vi "Autonomous Independent.vi"() -> ()   [LabVIEW 2016]
doc: "This VI is called when autonomous begins, and will automatically be terminated when autonomous ends. You can carry out timed or sensor driven robot movement independently without needing to return to the caller."
uses:
  <vilib>/Rock Robotics/WPI/Solenoid/WPI_SolenoidValue.ctl
  <vilib>/Rock Robotics/WPI/ThirdParty/CanMotor/TalonSRX/WPI_CANTalonSRX_APIControlMode.ctl
  <vilib>/Rock Robotics/Network Tables/NT Read String.vi
  Robot Global Data.vi
  <vilib>/Rock Robotics/WPI/Solenoid/WPI_SolenoidSetEnum.vi
  <vilib>/Rock Robotics/WPI/Utilities/WPI_GetSetVariantRefNum.vi
  <vilib>/addons/control/pid/pid.llb/PID (DBL).vi
  <vilib>/Rock Robotics/Network Tables/NT Read Number.vi
  <vilib>/addons/control/pid/NI_PID_pid.lvlib
  navX Library v2/navX Library v2.lvlib
panel:
  out "DriveStraight 3":T1(graph)
  out "DriveStraight 2":T1(graph)
  in  "ForwardPID 2":T2={"proportional gain (Kc)"=0.001, "integral time (Ti, min)"=0.1, "derivative time (Td, min)"=0.0}
  in  "YawFactor":dbl=0.01 format="%#_13g"
  out "YawCorrection":dbl(graph)
  out "Left V 5":cluster{"output":dbl, dbl, "Numeric":dbl}(graph)
  out "Right V 5":cluster{"output":dbl, dbl, "Numeric":dbl}(graph)
  out "Yaw 5":cluster{"Numeric":dbl, "Yaw":dbl}(graph)
  out "DriveStraight 7":T1(graph)
  out "Left V 4":cluster{"output":dbl, dbl, "Numeric":dbl}(graph)
  out "Right V 4":cluster{"output":dbl, dbl, "Numeric":dbl}(graph)
  out "Yaw 4":cluster{"Numeric":dbl, "Yaw":dbl}(graph)
  out "DriveStraight 6":T1(graph)
  out "Left V 3":cluster{"output":dbl, dbl, "Numeric":dbl}(graph)
  out "Right V 3":cluster{"output":dbl, dbl, "Numeric":dbl}(graph)
  out "Yaw 3":cluster{"Numeric":dbl, "Yaw":dbl}(graph)
  out "DriveStraight 5":T1(graph)
  out "Left V 2":cluster{"output":dbl, dbl, "Numeric":dbl}(graph)
  out "Right V 2":cluster{"output":dbl, dbl, "Numeric":dbl}(graph)
  out "Yaw 2":cluster{"Numeric":dbl, "Yaw":dbl}(graph)
  in  "RightPID":T2
  out "DriveStraight 4":T1(graph)
  out "Yaw":cluster{"Numeric":dbl, "Yaw":dbl}(graph)
  in  "ForwardPID":T2={"proportional gain (Kc)"=0.001, "integral time (Ti, min)"=0.1, "derivative time (Td, min)"=0.0}
  out "DriveStraight":T1(graph)
  in  "Center":dbl=160.0 format="%#_13g"
  in  "MOE":dbl=25.0 format="%#_13g"
  in  "Speed 2":dbl=0.45 format="%#_13g"
  in  "PID gains L":T2={"proportional gain (Kc)"=0.65, "integral time (Ti, min)"=0.01, "derivative time (Td, min)"=0.0} {"derivative time (Td, min)" format="%.3f"; "integral time (Ti, min)" format="%.6f"; "proportional gain (Kc)" format="%.6f"}
  in  "PID gains R":T2={"proportional gain (Kc)"=0.65, "integral time (Ti, min)"=0.01, "derivative time (Td, min)"=0.0} {"derivative time (Td, min)" format="%.3f"; "integral time (Ti, min)" format="%.6f"; "proportional gain (Kc)" format="%.6f"}
  in  "Range":cluster{"output high":dbl, "output low":dbl}={"output high"=1.0, "output low"=-0.5} {"output low" format="%.2f"; "output high" format="%.2f"}
  out "Left V":cluster{"output":dbl, dbl, "Numeric":dbl}(graph)
  out "Right V":cluster{"output":dbl, dbl, "Numeric":dbl}(graph)
  in  "Speed":dbl=1.0 format="%#_13g"
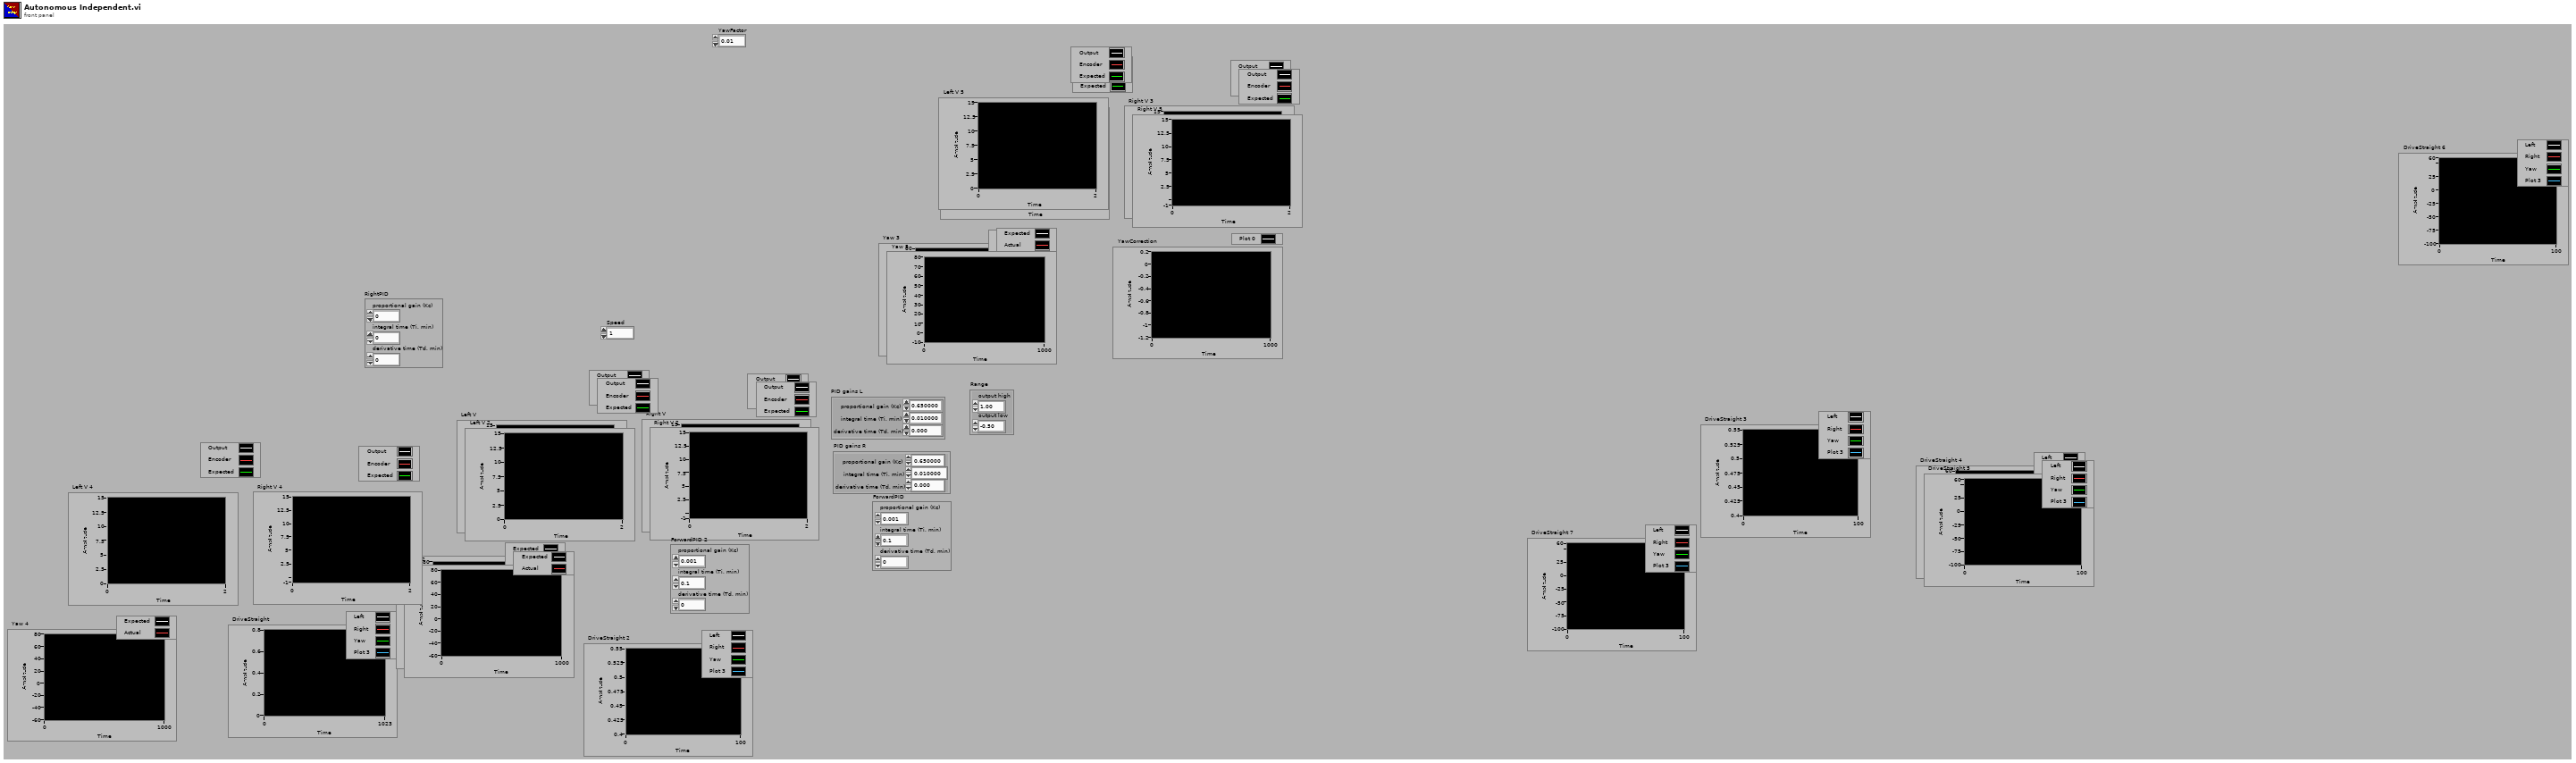
[diagram p1: front panel]
types:
  T1 = cluster{"[0]":dbl, "[1]":dbl, "[2]":dbl, "[3]":dbl, "[4]":dbl, "[5]":dbl, "[6]":dbl, "[7]":dbl, "[8]":dbl}
  T2 = cluster{"proportional gain (Kc)":dbl, "integral time (Ti, min)":dbl, "derivative time (Td, min)":dbl}
  T3 = typedef "WPI_SolenoidValue.ctl" = enum16{"Off", "On", "Forward", "Reverse"}
  T4 = typedef "WPI_CANTalonSRX_APIControlMode.ctl" = enum8{"Percent VBus", "Speed", "Position", "Slave", "Unchanged / Invalid", "Voltage Compensation", "Current", "Motion Profile", "Motion Magic"}
  T5 = typedef "WPI_SolenoidDevRef.ctl" = cluster{"DevStatus":errorcluster, "Pneumatics Control Module":u8, "Forward Solenoid Channel":T6, "Reverse Solenoid Channel":T6}
  T6 = typedef "WPI_SolenoidChannel.ctl" = enum8{"Solenoid 0", "Solenoid 1", "Solenoid 2", "Solenoid 3", "Solenoid 4", "Solenoid 5", "Solenoid 6", "Solenoid 7", "Invalid"}
  T7 = typedef "WPI_EncoderDevRef.ctl" = cluster{"DevStatus":errorcluster, "EncoderIndex":T8, "CounterIndex":T9, "DistancePerCount":dbl, "Decoding Type":T10}
  T8 = typedef "FPGA_EncoderIdx.ctl" = enum8{"Enc 0", "Enc 1", "Enc 2", "Enc 3", "Enc 4", "Enc 5", "Enc 6", "Enc 7", "Invalid"}
  T9 = typedef "FPGA_CounterCtrSystemIndex.ctl" = enum8{"Ctr 0", "Ctr 1", "Ctr 2", "Ctr 3", "Ctr 4", "Ctr 5", "Ctr 6", "Ctr 7", "Invalid"}
  T10 = typedef "WPI_EncoderType.ctl" = enum16{"1x", "2x", "4x"}
  T11 = typedef "navX Library v2.lvlib/Z900_navX_DeviceTypeDef.ctl" = cluster{"Interface":cluster{"Protocol":T12, "Update Rate (4Hz-100Hz)":u8, "navX Open TypeDef":variant}, "Notify Packet":refnum<notifier>, "Loop VI Refnum":refnum<vi>, "Ready to Close Occurrence Refnum":refnum<k4>}
  T12 = typedef "navX Library v2.lvlib/Z900_navX_ProtocolTypeDef.ctl" = enum16{"SERIAL", "I2C", "SPI"}
  T13 = typedef "WPI_RobotDriveDevRef.ctl" = cluster{"DevStatus":errorcluster, "Motors[]":T14[], "Square Inputs":bool, "Max Output":dbl}
  T14 = typedef "WPI_MotorControlDeviceRef.ctl" = cluster{"DeviceStatus":errorcluster, "Type":T15, "PWM":cluster{"PWM Channel":T16, "DeadBand":T17}, "CAN":cluster{"Device Number":u8, "SetOutput VI Ref":variant, "GetOutput VI Ref":variant, "Enable VI Ref":variant, "Disable VI Ref":variant, "Data":variant}, "Invert":bool}
  T15 = typedef "WPI_MotorControlType.ctl" = enum16{"PWM", "CAN"}
  T16 = typedef "FPGA_DIOPWMChannel.ctl" = enum8{"PWM 0", "PWM 1", "PWM 2", "PWM 3", "PWM 4", "PWM 5", "PWM 6", "PWM 7", "PWM 8", "PWM 9", "PWM MXP 0", "PWM MXP 1", "PWM MXP 2", "PWM MXP 3", "PWM MXP 4", "PWM MXP 5", "PWM MXP 6", "PWM MXP 7", "PWM MXP 8", "PWM MXP 9", "Invalid"}
  T17 = typedef "WPI_PWMDeadband.ctl" = cluster{"Name":string, "maxPositivePwm":i32, "minPositivePwm":i32, "centerPwm":i32, "maxNegativePwm":i32, "minNegativePwm":i32, "angularRange":u16}
  T18 = cluster{"Yaw":dbl, "Roll":dbl, "Pitch":dbl, "Heading":dbl, "Fused Heading":dbl}
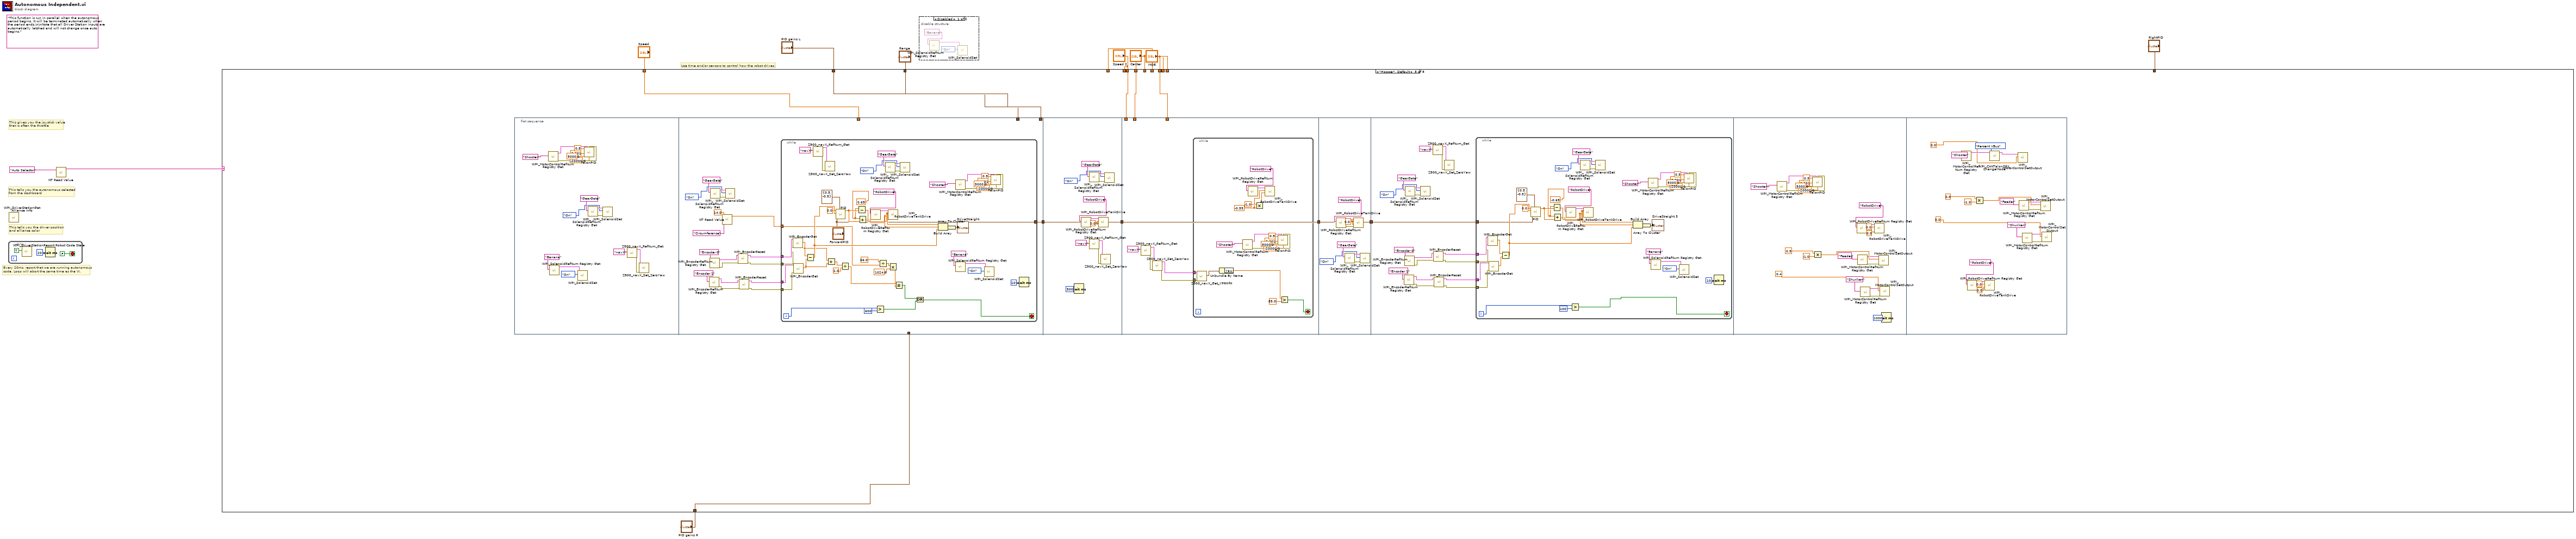
[diagram p0: block diagram]
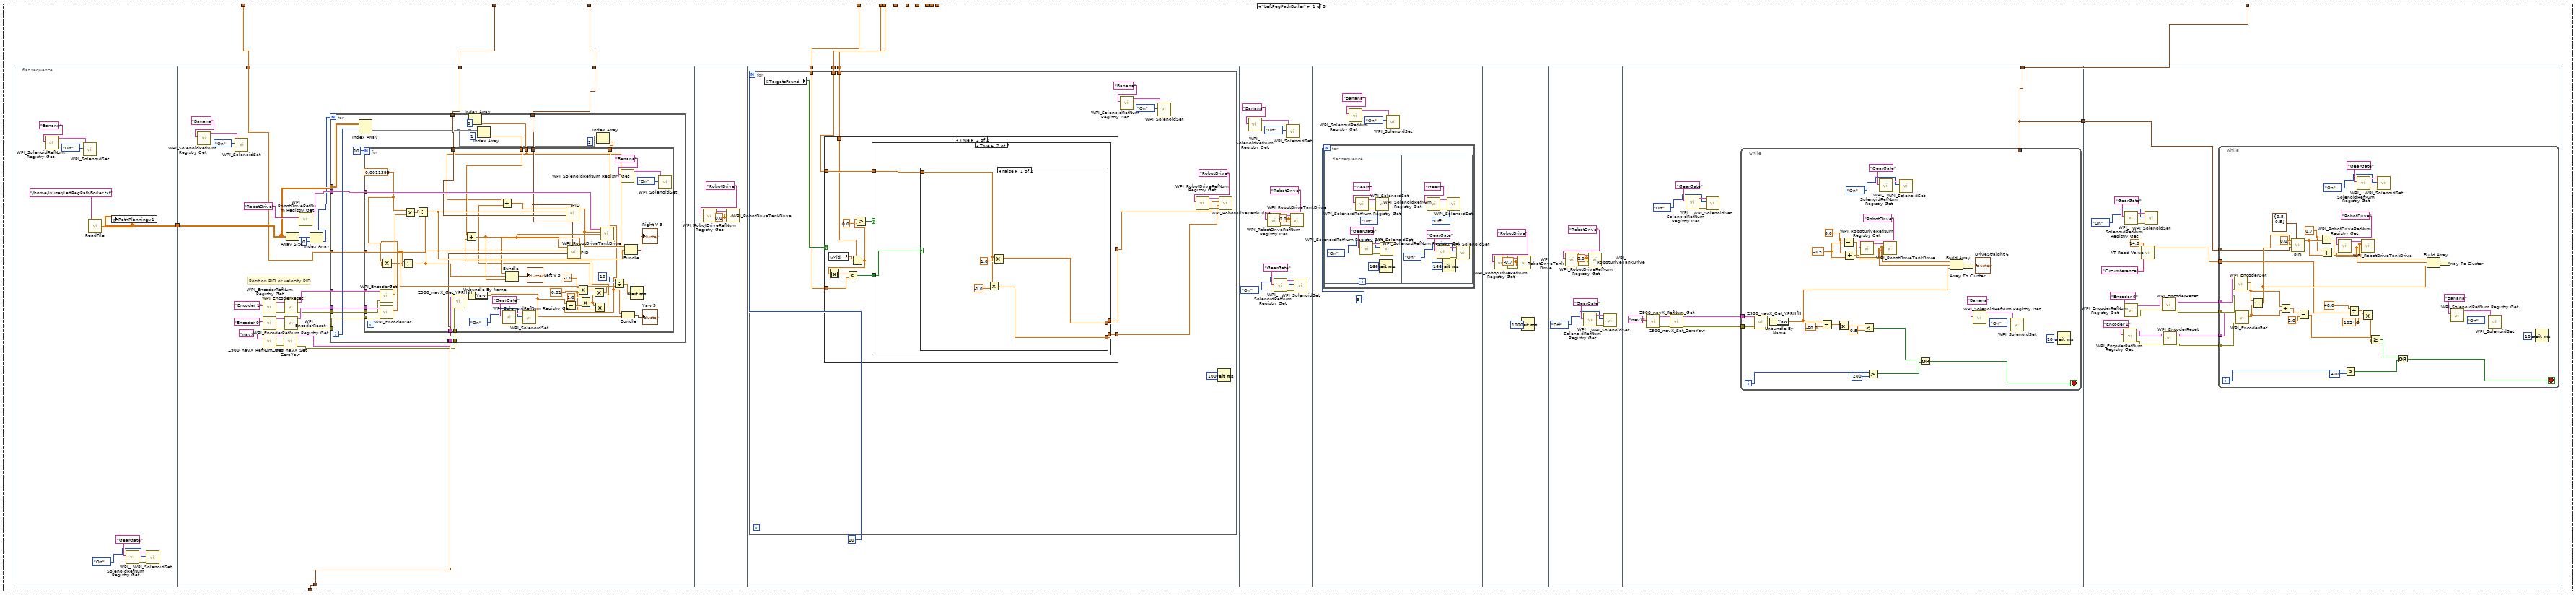
[diagram p3: hidden frame]
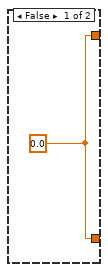
[diagram p4: hidden frame]
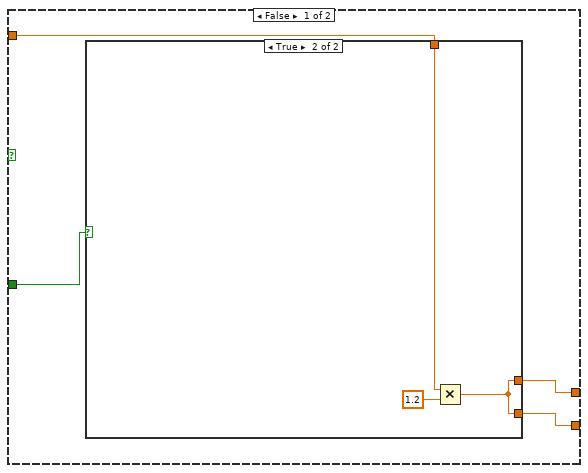
[diagram p5: hidden frame]
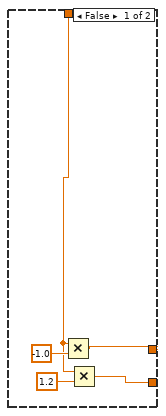
[diagram p6: hidden frame]
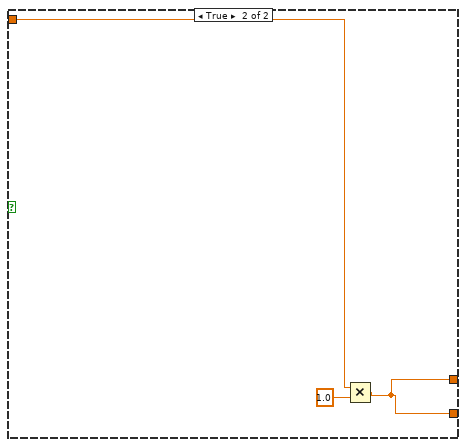
[diagram p7: hidden frame]
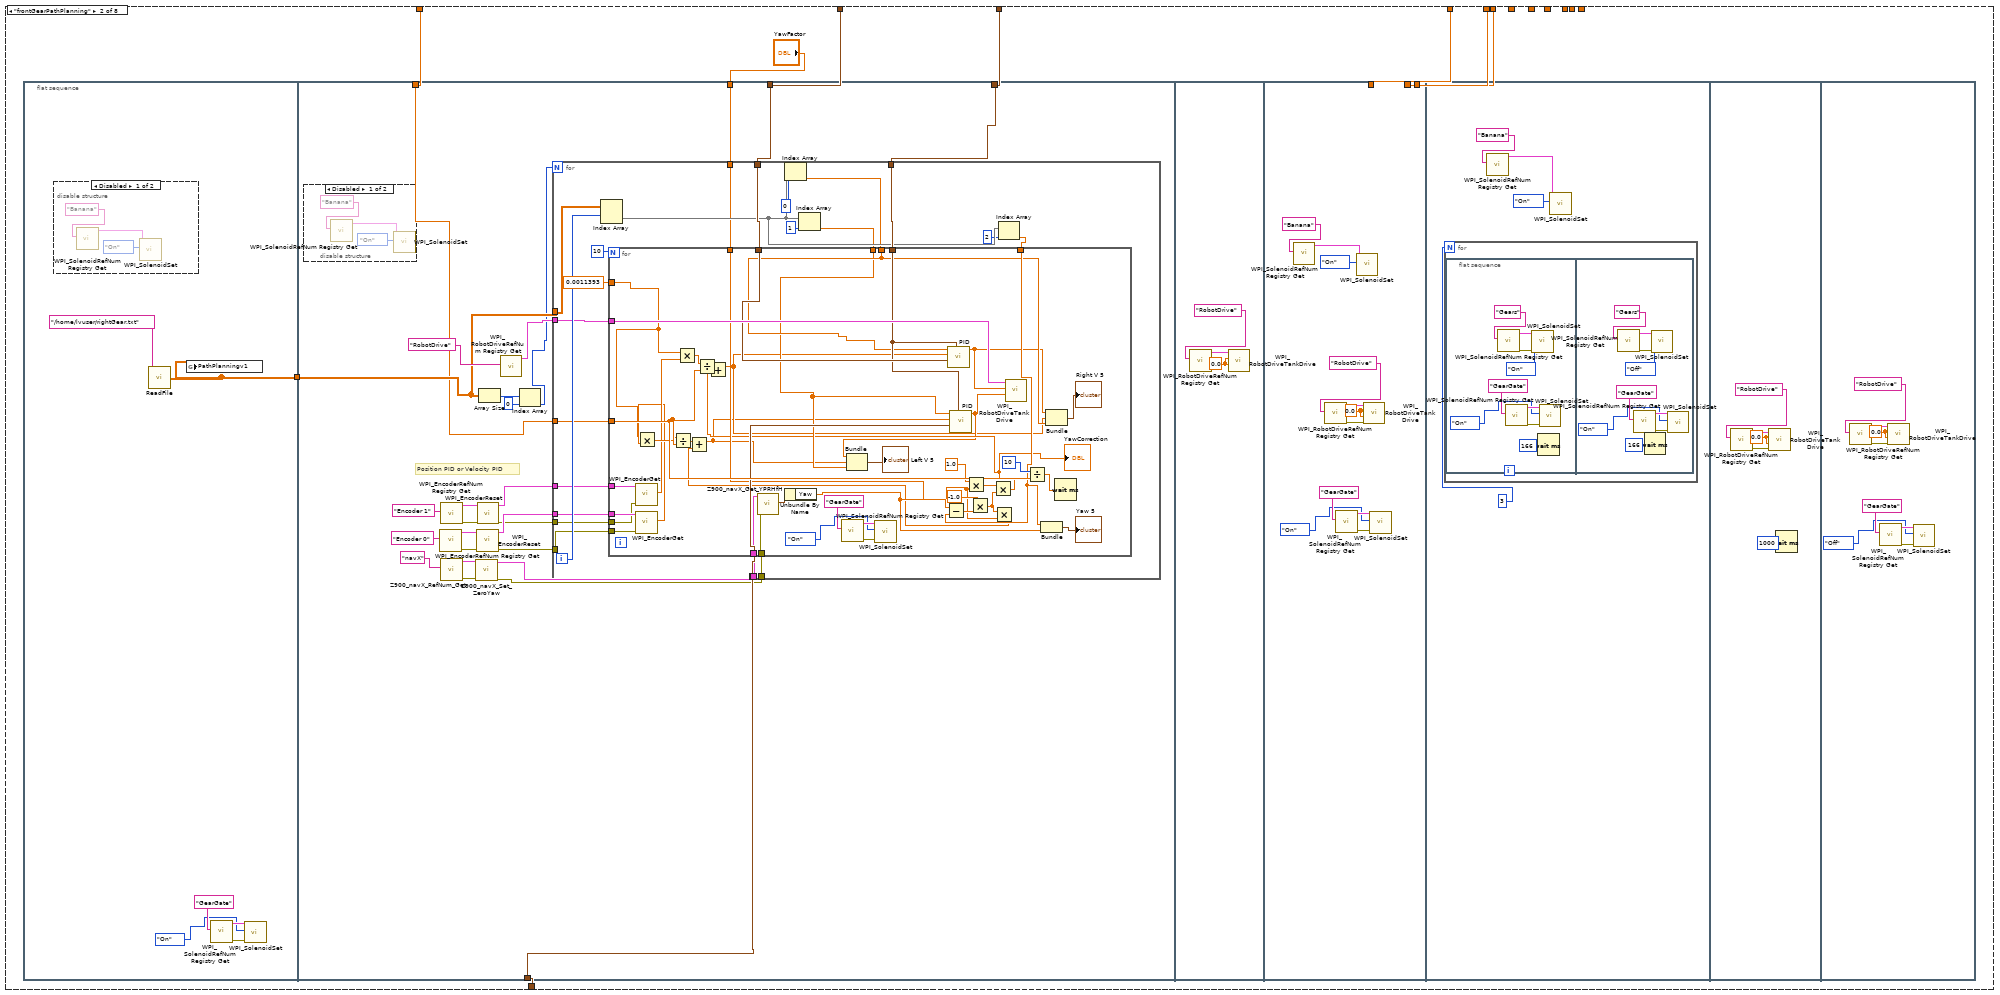
[diagram p8: hidden frame]
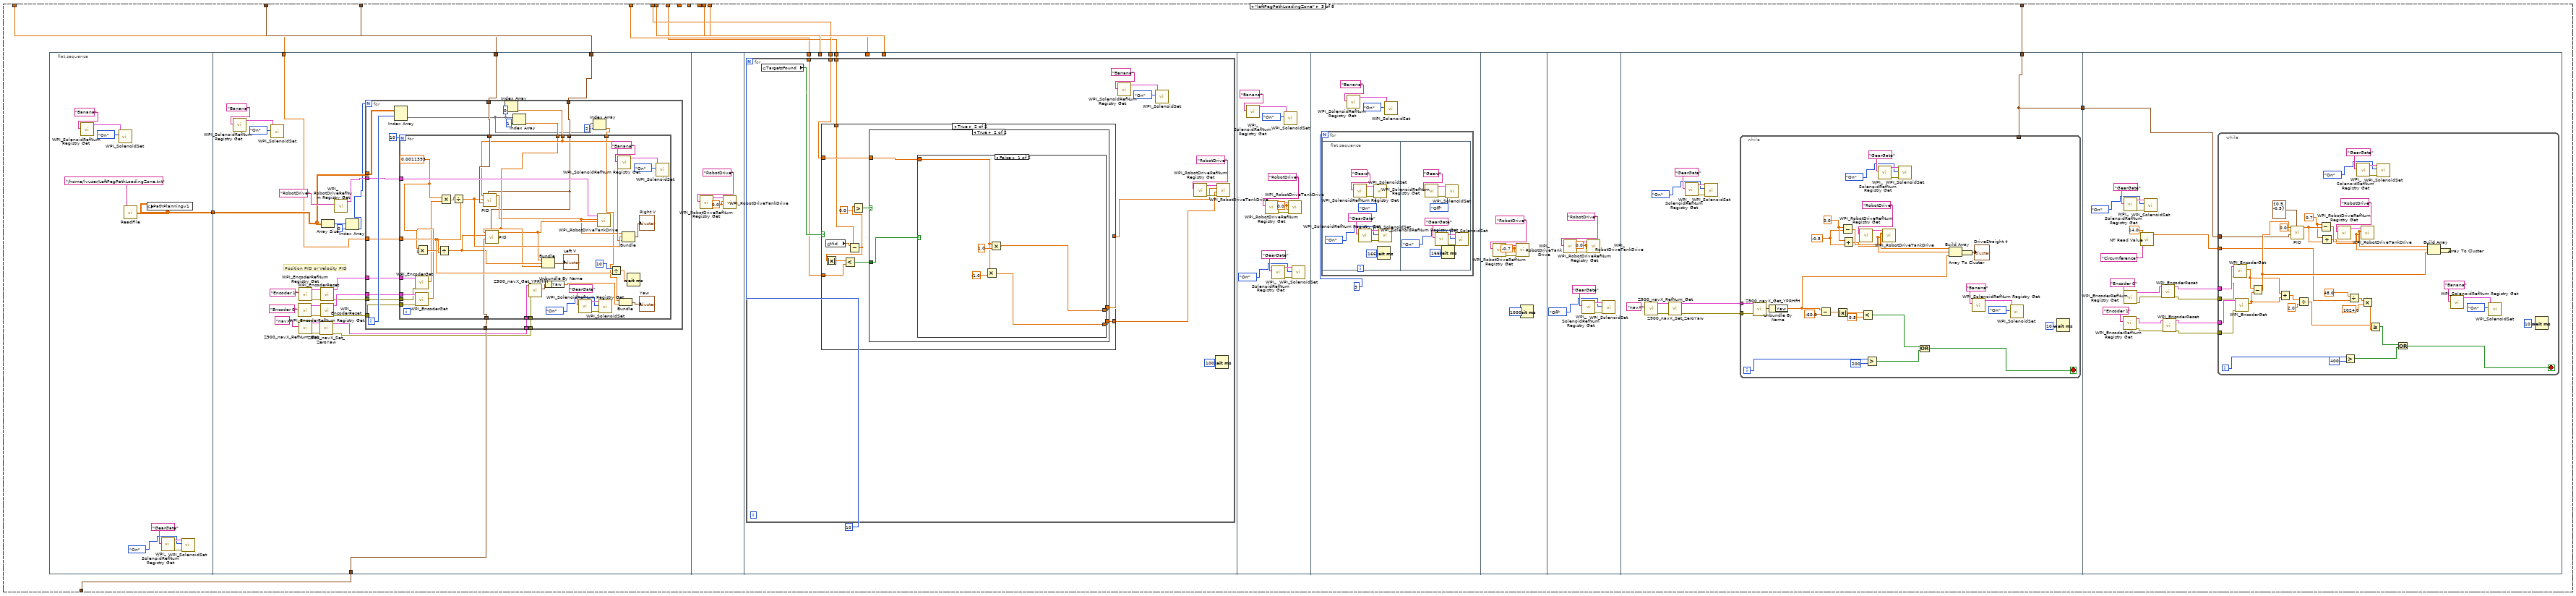
[diagram p11: hidden frame]
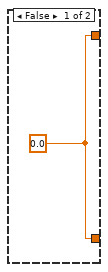
[diagram p12: hidden frame]
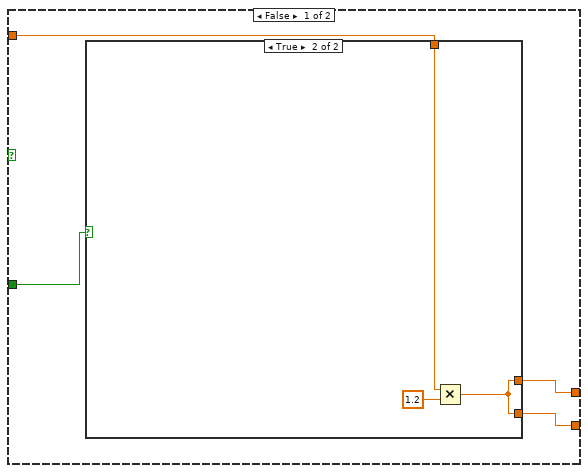
[diagram p13: hidden frame]
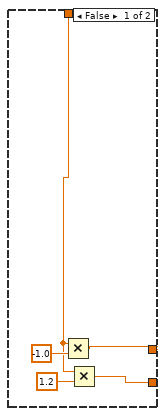
[diagram p14: hidden frame]
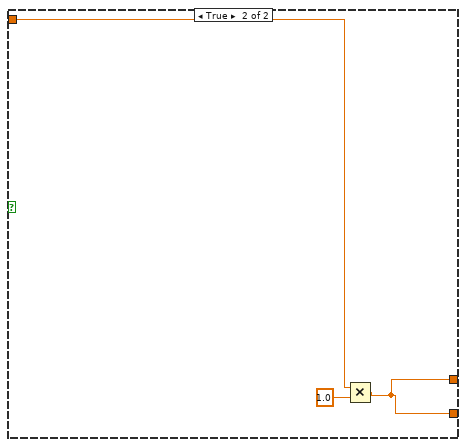
[diagram p15: hidden frame]
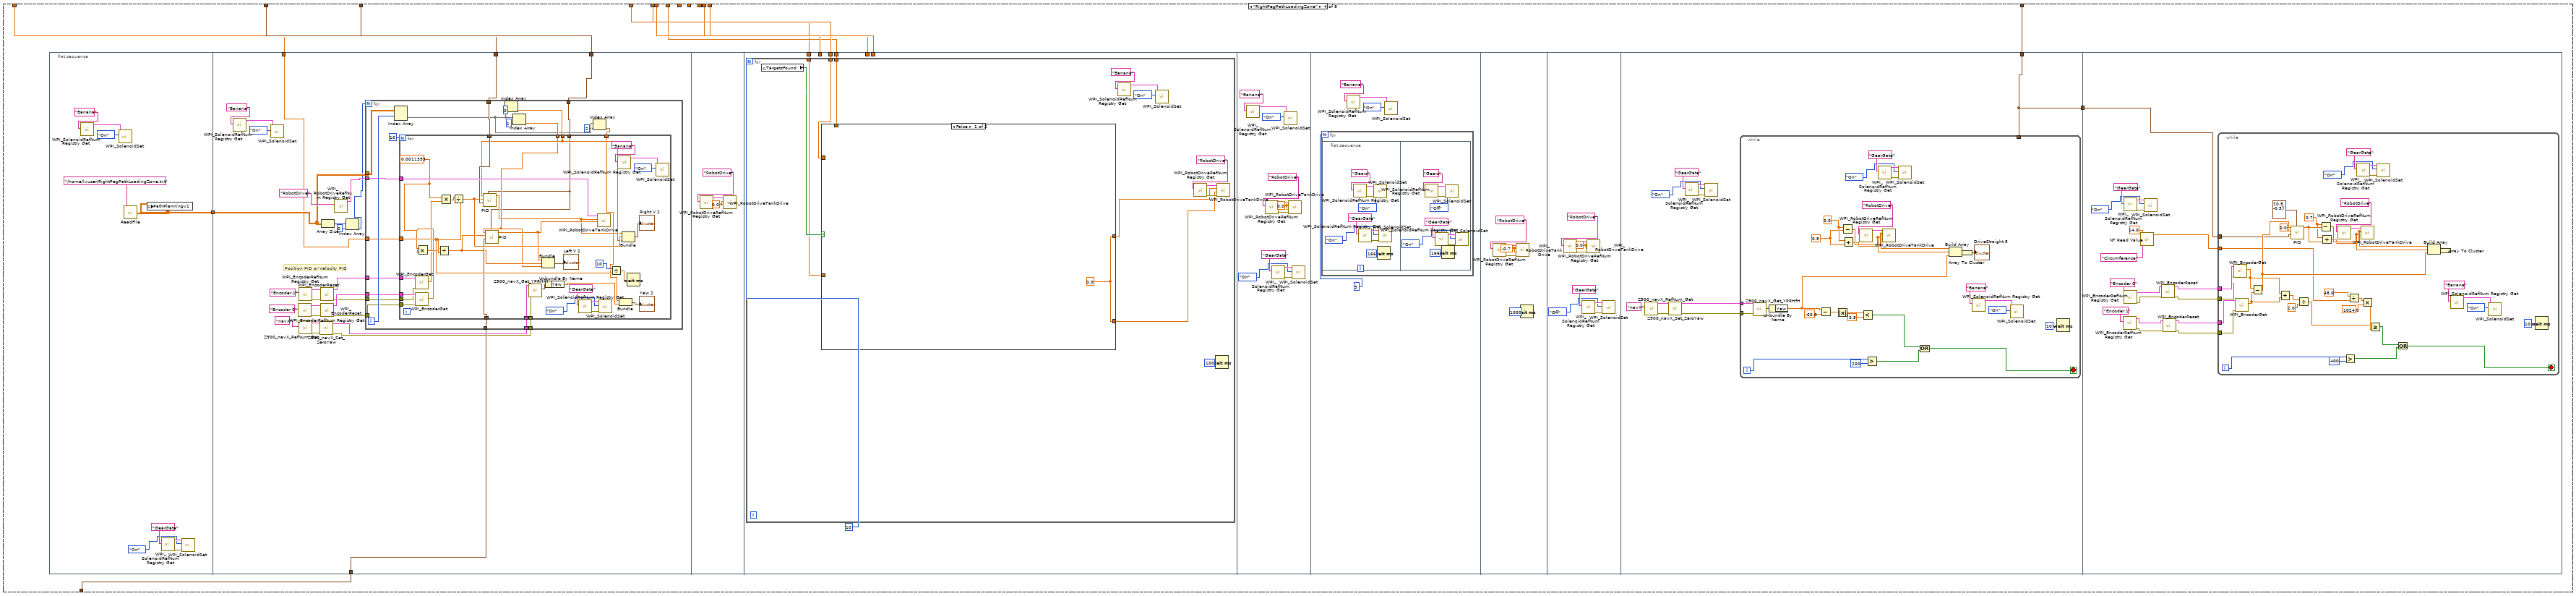
[diagram p16: hidden frame]
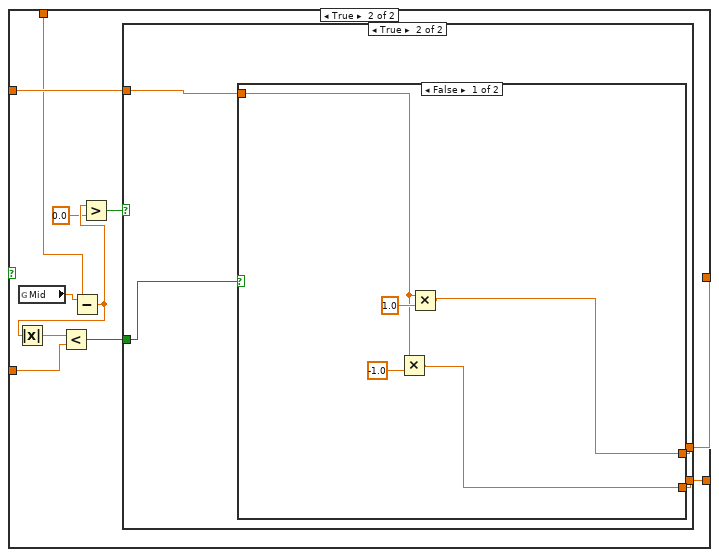
[diagram p17: hidden frame]
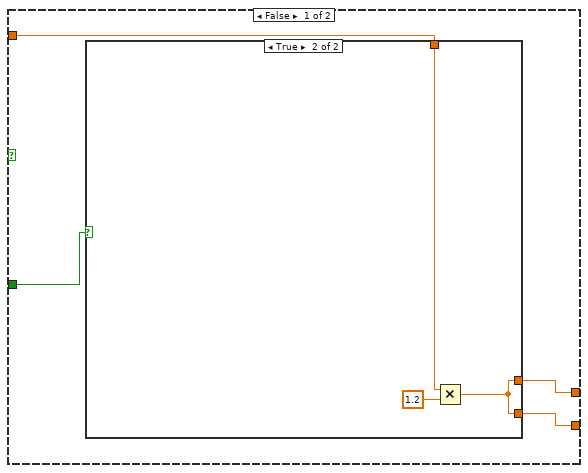
[diagram p18: hidden frame]
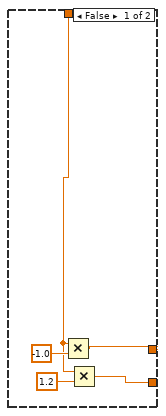
[diagram p19: hidden frame]
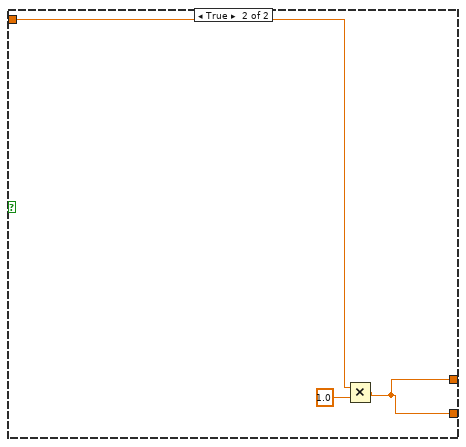
[diagram p20: hidden frame]
diagram:
  (unwired) "This function is run in parallel when the autonomous period begins. It will be terminated automatically when the period ends.\n\nNote that all Driver Station inputs are automatically latched and will not change once auto begins."
  # "This tells you the autonomous selected\nfrom the dashboard"
  # "Every 20ms, report that we are running autonomous\ncode. Loop will abort the same time as the VI."
  # "This gives you the joystick value\nthat is often the throttle"
  # "Use time and/or sensors to control how the robot drives."
  # "This tells you the driver position\nand alliance color"
  n1 = while {
    stop <- FALSE stop-if-true
    n2 = call <vilib>:"WPI_DriverStationReport Robot Code State.vi"("Autonomous"=TRUE) -> ()  [unwired: 10 in, 1 out]
    n3 = Wait (ms)(milliseconds to wait=u32 20) -> ()  [unwired: 1 out]
  }
  n4 = call <vilib>:"WPI_DriverStationGet Alliance Info.vi"() -> ()  [unwired: 12 out]
  n5 = call-poly <vilib>:"NT Read Value.vi"("Name"="Auto Selector") -> ("String"=w9:string)  [unwired: 9 in, 1 out]
  n6 = case shown="\"Hopper\", Default" w9 {
    tunnel: "Range" -> [w19 w331 w500 w805 w1109 w1341 w1587 _]
    tunnel: "PID gains L" -> [w20 w332 w499 w804 w1108 w1340 w1588 _]
    tunnel: "Speed 2" -> [w15 w328 w498 w803 w1107 w1339 w1584 _]
    tunnel: "Center" -> [_ _ w497 w802 _ _ _ _]
    tunnel: "MOE" -> [_ _ w496 w801 _ _ _ _]
    tunnel: "Speed" -> [w21 w333 w489 w800 w1104 w1336 w1589 _]
    tunnel: "Center" -> [_ _ _ _ _ _ _ _]
    tunnel: "MOE" -> [_ _ _ _ _ _ _ _]
    tunnel: "Center" -> [_ _ w493 w797 w1106 w1338 _ _]
    tunnel: "MOE" -> [_ _ _ _ w1105 w1337 _ _]
    tunnel: "PID gains R" -> [w14 w327 w495 w799 w1103 w1335 w1582 _]
    tunnel: "Speed 2" -> [w16 w329 w494 w798 _ _ w1585 _]
    tunnel: "MOE" -> [w17 w330 w492 w796 _ _ w1586 _]
    tunnel: "RightPID" -> [w18 _ w491 w795 _ _ w1583 _]
    frame "LeftPegPathBoiler" {
      n7 = flat-sequence {
        tunnel: [w31] -> w23
        tunnel: w23 -> [w56]
        tunnel: w19 -> [w55]
        tunnel: w20 -> [w54]
        tunnel: w21 -> [w53]
        tunnel: w14 -> [w52]
        tunnel: w16 -> [w134]
        tunnel: w15 -> [w133]
        tunnel: w17 -> [w132]
        tunnel: w18 -> [w231]
        tunnel: [w231] -> w22
        tunnel: w22 -> [w270]
        frame #0 {
          n8 = call <vilib>:"WPI_SolenoidRefNum Registry Get.vi"("refnum name"="Banana") -> ("SolenoidDevRef"=w26:T5)  [unwired: 9 in, 1 out]
          n9 = call-poly <vilib>:"WPI_SolenoidSet.vi"("Value"=WPI_SolenoidValue."On", "SolenoidDevRef"=w26) -> ()  [unwired: 8 in, 2 out]
          n10 = call "ReadFile.vi"("Name"="/home/lvuser/LeftPegPathBoiler.txt") -> ("Array - Numeric"=w31:dbl[][])
          n11 = global write "Robot Global Data.vi" "PathPlanningv1"(w31) -> ()
          n12 = call <vilib>:"WPI_SolenoidRefNum Registry Get.vi"("refnum name"="GearGate") -> ("error out"=w30:errorcluster, "SolenoidDevRef"=w29:T5)  [unwired: 9 in]
          n13 = call-poly <vilib>:"WPI_SolenoidSet.vi"("error in (no error)"=w30, "Value"=WPI_SolenoidValue."On", "SolenoidDevRef"=w29) -> ()  [unwired: 7 in, 2 out]
        }
        frame #1 {
          # "Position PID or Velocity PID"
          n14 = call <vilib>:"WPI_SolenoidRefNum Registry Get.vi"("refnum name"="Banana") -> ("SolenoidDevRef"=w51:T5)  [unwired: 9 in, 1 out]
          n15 = call-poly <vilib>:"WPI_SolenoidSet.vi"("Value"=WPI_SolenoidValue."On", "SolenoidDevRef"=w51) -> ()  [unwired: 8 in, 2 out]
          n16 = call <vilib>:"WPI_EncoderRefNum Registry Get.vi"("refnum name"="Encoder 0") -> ("error out"=w45:errorcluster, "EncoderDevRef"=w44:T7)  [unwired: 9 in]
          n17 = call <vilib>:"WPI_EncoderRefNum Registry Get.vi"("refnum name"="Encoder 1") -> ("error out"=w47:errorcluster, "EncoderDevRef"=w46:T7)  [unwired: 9 in]
          n18 = call "Z900_navX_RefNum_Get.vi"("refnum name"="navX") -> ("error out"=w36:errorcluster, "navX Device"=w37:T11)  [unwired: 9 in]
          n19 = call "Z900_navX_Set_ZeroYaw.vi"("error in (no error)"=w36, "navX Device"=w37) -> ("error out"=w34:errorcluster, "navX Device"=w35:T11)  [unwired: 8 in]
          n20 = call <vilib>:"WPI_EncoderReset.vi"("error in (no error)"=w45, "EncoderDevRef"=w44) -> ("error out"=w41:errorcluster, "EncoderDevRef"=w42:T7)  [unwired: 8 in]
          n21 = call <vilib>:"WPI_EncoderReset.vi"("error in (no error)"=w47, "EncoderDevRef"=w46) -> ("error out"=w40:errorcluster, "EncoderDevRef"=w43:T7)  [unwired: 8 in]
          n22 = Array Size(array=w56) -> (size(s)=w60:i32[])
          n23 = call <vilib>:"WPI_RobotDriveRefNum Registry Get.vi"("refnum name"="RobotDrive") -> ("RobotDriveDevRef"=w57:T13)  [unwired: 9 in, 1 out]
          n24 = Index Array(array=w60, index=0) -> (element=w48:i32)
          n25 = for {
            N: w48 -> [_]
            tunnel: w56 -> [w79]
            tunnel: w52 -> [w76]
            tunnel: w54 -> [w75]
            tunnel: w55 -> [w74]
            tunnel: w57 -> [w73]
            tunnel: w53 -> [w72]
            tunnel: w43 -> [w71]
            tunnel: w42 -> [w70]
            tunnel: w41 -> [w69]
            tunnel: w40 -> [w68]
            tunnel: w35 -> [w65]
            tunnel: w34 -> [w64]
            i -> [w78]
            n26 = Index Array(array=w79, index (row)=w78) -> (element=w63:dbl[])  [unwired: 1 in]
            n27 = Index Array(array=w63, index=0) -> (element=w66:dbl)
            n28 = Index Array(array=w63, index=1) -> (element=w67:dbl)
            n29 = Index Array(array=w63, index=2) -> (element=w61:dbl)
            n30 = for {
              N: 10 -> [_]
              tunnel: w76 -> [w113]
              tunnel: w75 -> [w127]
              tunnel: w74 -> [w100]
              tunnel: w73 -> [w128]
              tunnel: w72 -> [w114]
              tunnel: w71 -> [w108]
              tunnel: w70 -> [w107]
              tunnel: w69 -> [w104]
              tunnel: w68 -> [w103]
              tunnel: w66 -> [w83]
              tunnel: w67 -> [w86]
              tunnel: w65 -> [w99]
              tunnel: w64 -> [w98]
              tunnel: w61 -> [w94]
              w88 = 0.01
              w109 = 0.0011393 ("x")
              n31 = call <vilib>:"WPI_EncoderGet.vi"("error in (no error)"=w103, "EncoderDevRef"=w108) -> ("Distance"=w105:dbl)  [unwired: 4 in, 5 out]
              n32 = call <vilib>:"WPI_EncoderGet.vi"("error in (no error)"=w104, "EncoderDevRef"=w107) -> ("Distance"=w106:dbl)  [unwired: 4 in, 5 out]
              n33 = Multiply(x=w109, y=w106) -> (x*y=w110:dbl)
              n34 = Divide(x=w110, y=w114) -> (x/y=w112:dbl)
              n35 = Multiply(x=w109, y=w105) -> (x*y=w111:dbl)
              n36 = Divide(x=w111, y=w114) -> (x/y=w124:dbl)
              n37 = call "Z900_navX_Get_YPRHfH.vi"("error in (no error)"=w98, "navX Device"=w99) -> ("YRPHfH"=w97:T18)  [unwired: 6 in, 3 out]
              n38 = Unbundle By Name(w97) -> ("Yaw"=w95:dbl)
              n39 = call <vilib>:"WPI_SolenoidRefNum Registry Get.vi"("refnum name"="GearGate") -> ("error out"=w123:errorcluster, "SolenoidDevRef"=w122:T5)  [unwired: 9 in]
              n40 = call-poly <vilib>:"WPI_SolenoidSet.vi"("error in (no error)"=w123, "Value"=WPI_SolenoidValue."On", "SolenoidDevRef"=w122) -> ()  [unwired: 7 in, 2 out]
              n41 = Subtract(x=w95, y=w94) -> (x-y=w93:dbl)
              n42 = Multiply(x=-1.0 ("Speed"), y=w88) -> (x*y=w90:dbl)
              n43 = Multiply(x=1.0, y=w93) -> (x*y=w91:dbl)
              n44 = Multiply(x=w90, y=w91) -> (x*y=w82:dbl)
              n45 = Add(x=w83, y=w82) -> (x+y=w84:dbl)
              n46 = call-poly <vilib>:"PID.vi"("output range"=w100, "PID gains"=w127, "process variable"=w124, "setpoint"=w84) -> ("output"=w101:dbl)  [unwired: 6 in, 1 out]
              n47 = Multiply(x=w91, y=w88) -> (x*y=w85:dbl)
              n48 = Add(x=w86, y=w85) -> (x+y=w87:dbl)
              n49 = call-poly <vilib>:"PID.vi"("output range"=w100, "PID gains"=w113, "process variable"=w112, "setpoint"=w87) -> ("output"=w102:dbl)  [unwired: 6 in, 1 out]
              n50 = Bundle("output"=w102, w112, w87) -> (→"Left V 3":cluster{"output":dbl, dbl, dbl})  [unwired: 1 in]
              n51 = call <vilib>:"WPI_RobotDriveTankDrive.vi"("Right axis value"=w102, "Left axis value"=w101, "RobotDriveDevRef"=w128) -> ()  [unwired: 6 in, 3 out]
              n52 = Divide(x=10, y=w114) -> (x/y=w115:dbl)
              n53 = call <vilib>:"WPI_SolenoidRefNum Registry Get.vi"("refnum name"="Banana") -> ("SolenoidDevRef"=w119:T5)  [unwired: 9 in, 1 out]
              n54 = Bundle("Numeric"=w94, "Yaw"=w95) -> (→"Yaw 3":cluster{"Numeric":dbl, "Yaw":dbl})  [unwired: 1 in]
              n55 = Bundle("output"=w101, w124, "Numeric"=w83) -> (→"Right V 3":cluster{"output":dbl, dbl, "Numeric":dbl})  [unwired: 1 in]
              n56 = Wait (ms)(milliseconds to wait=w115) -> ()  [unwired: 1 out]
              n57 = call-poly <vilib>:"WPI_SolenoidSet.vi"("Value"=WPI_SolenoidValue."On", "SolenoidDevRef"=w119) -> ()  [unwired: 8 in, 2 out]
            }
          }
        }
        frame #2 {
          w130 = 0.0 ("Right axis value")
          n58 = call <vilib>:"WPI_RobotDriveRefNum Registry Get.vi"("refnum name"="RobotDrive") -> ("RobotDriveDevRef"=w131:T13)  [unwired: 9 in, 1 out]
          n59 = call <vilib>:"WPI_RobotDriveTankDrive.vi"("Right axis value"=w130, "Left axis value"=w130, "RobotDriveDevRef"=w131) -> ()  [unwired: 6 in, 3 out]
        }
        frame #3 {
          n60 = for {
            N: 10 -> [_]
            tunnel: w134 -> [w138]
            tunnel: w133 -> [w137]
            tunnel: w132 -> [w136]
            n61 = global read "Robot Global Data.vi" "TargetsFound"() -> (w141:bool)
            n62 = case shown="True" w141 {
              tunnel: [w149 w157] -> w140
              tunnel: [w149 w156] -> w139
              tunnel: w138 -> [_ w152]
              tunnel: w137 -> [_ w151]
              tunnel: w136 -> [_ w150]
              frame False {
                w149 = 0.0
              }
              frame True {
                n63 = global read "Robot Global Data.vi" "Mid"() -> (w160:dbl)
                n64 = Subtract(x=w160, y=w151) -> (x-y=w154:dbl)
                n65 = Absolute Value(x=w154) -> (abs(x)=w159:dbl)
                n66 = Less?(x=w159, y=w150) -> (x < y?=w158:bool)
                n67 = Greater?(x=w154, y=0.0) -> (0:w155:bool)
                n68 = case shown="True" w155 {
                  tunnel: w158 -> [w163 w176]
                  tunnel: [w161 w174] -> w157
                  tunnel: [w162 w175] -> w156
                  tunnel: w152 -> [w164 w173]
                  frame False {
                    n69 = case shown="True" w163 {
                      tunnel: [w169 w172] -> w162
                      tunnel: [w167 w172] -> w161
                      tunnel: w164 -> [w165 w170]
                      frame False {
                        n70 = Multiply(x=w165, y=-1.0) -> (x*y=w169:dbl)
                        n71 = Multiply(x=w165, y=1.2) -> (x*y=w167:dbl)
                      }
                      frame True {
                        n72 = Multiply(x=w170, y=1.2) -> (x*y=w172:dbl)
                      }
                    }
                  }
                  frame True {
                    n73 = case shown="False" w176 {
                      tunnel: [w181 w184] -> w175
                      tunnel: [w179 w184] -> w174
                      tunnel: w173 -> [w177 w182]
                      frame False {
                        n74 = Multiply(x=w177, y=-1.0) -> (x*y=w179:dbl)
                        n75 = Multiply(x=w177, y=1.0) -> (x*y=w181:dbl)
                      }
                      frame True {
                        n76 = Multiply(x=w182, y=1.0) -> (x*y=w184:dbl)
                      }
                    }
                  }
                }
              }
            }
            n77 = call <vilib>:"WPI_SolenoidRefNum Registry Get.vi"("refnum name"="Banana") -> ("SolenoidDevRef"=w144:T5)  [unwired: 9 in, 1 out]
            n78 = call-poly <vilib>:"WPI_SolenoidSet.vi"("Value"=WPI_SolenoidValue."On", "SolenoidDevRef"=w144) -> ()  [unwired: 8 in, 2 out]
            n79 = call <vilib>:"WPI_RobotDriveRefNum Registry Get.vi"("refnum name"="RobotDrive") -> ("error out"=w147:errorcluster, "RobotDriveDevRef"=w148:T13)  [unwired: 9 in]
            n80 = Wait (ms)(milliseconds to wait=100) -> ()  [unwired: 1 out]
            n81 = call <vilib>:"WPI_RobotDriveTankDrive.vi"("error in (no error)"=w147, "Right axis value"=w140, "Left axis value"=w139, "RobotDriveDevRef"=w148) -> ()  [unwired: 5 in, 3 out]
          }
        }
        frame #4 {
          w193 = 0.0 ("Left axis value")
          n82 = call <vilib>:"WPI_SolenoidRefNum Registry Get.vi"("refnum name"="Banana") -> ("SolenoidDevRef"=w187:T5)  [unwired: 9 in, 1 out]
          n83 = call <vilib>:"WPI_RobotDriveRefNum Registry Get.vi"("refnum name"="RobotDrive") -> ("error out"=w194:errorcluster, "RobotDriveDevRef"=w195:T13)  [unwired: 9 in]
          n84 = call <vilib>:"WPI_SolenoidRefNum Registry Get.vi"("refnum name"="GearGate") -> ("error out"=w191:errorcluster, "SolenoidDevRef"=w190:T5)  [unwired: 9 in]
          n85 = call-poly <vilib>:"WPI_SolenoidSet.vi"("Value"=WPI_SolenoidValue."On", "SolenoidDevRef"=w187) -> ()  [unwired: 8 in, 2 out]
          n86 = call <vilib>:"WPI_RobotDriveTankDrive.vi"("error in (no error)"=w194, "Right axis value"=w193, "Left axis value"=w193, "RobotDriveDevRef"=w195) -> ()  [unwired: 5 in, 3 out]
          n87 = call-poly <vilib>:"WPI_SolenoidSet.vi"("error in (no error)"=w191, "Value"=WPI_SolenoidValue."On", "SolenoidDevRef"=w190) -> ()  [unwired: 7 in, 2 out]
        }
        frame #5 {
          n88 = for {
            N: 3 -> [_]
            n89 = flat-sequence {
              frame #0 {
                n90 = call <vilib>:"WPI_SolenoidRefNum Registry Get.vi"("refnum name"="Gears") -> ("error out"=w208:errorcluster, "SolenoidDevRef"=w207:T5)  [unwired: 9 in]
                n91 = call <vilib>:"WPI_SolenoidRefNum Registry Get.vi"("refnum name"="GearGate") -> ("error out"=w203:errorcluster, "SolenoidDevRef"=w202:T5)  [unwired: 9 in]
                n92 = call-poly <vilib>:"WPI_SolenoidSet.vi"("error in (no error)"=w208, "Value"=WPI_SolenoidValue."On", "SolenoidDevRef"=w207) -> ()  [unwired: 7 in, 2 out]
                n93 = Wait (ms)(milliseconds to wait=166) -> ()  [unwired: 1 out]
                n94 = call-poly <vilib>:"WPI_SolenoidSet.vi"("error in (no error)"=w203, "Value"=WPI_SolenoidValue."On", "SolenoidDevRef"=w202) -> ()  [unwired: 7 in, 2 out]
              }
              frame #1 {
                n95 = call <vilib>:"WPI_SolenoidRefNum Registry Get.vi"("refnum name"="Gears") -> ("error out"=w217:errorcluster, "SolenoidDevRef"=w216:T5)  [unwired: 9 in]
                n96 = call <vilib>:"WPI_SolenoidRefNum Registry Get.vi"("refnum name"="GearGate") -> ("error out"=w212:errorcluster, "SolenoidDevRef"=w211:T5)  [unwired: 9 in]
                n97 = Wait (ms)(milliseconds to wait=166) -> ()  [unwired: 1 out]
                n98 = call-poly <vilib>:"WPI_SolenoidSet.vi"("error in (no error)"=w217, "Value"=WPI_SolenoidValue."Off", "SolenoidDevRef"=w216) -> ()  [unwired: 7 in, 2 out]
                n99 = call-poly <vilib>:"WPI_SolenoidSet.vi"("error in (no error)"=w212, "Value"=WPI_SolenoidValue."On", "SolenoidDevRef"=w211) -> ()  [unwired: 7 in, 2 out]
              }
            }
          }
          n100 = call <vilib>:"WPI_SolenoidRefNum Registry Get.vi"("refnum name"="Banana") -> ("SolenoidDevRef"=w198:T5)  [unwired: 9 in, 1 out]
          n101 = call-poly <vilib>:"WPI_SolenoidSet.vi"("Value"=WPI_SolenoidValue."On", "SolenoidDevRef"=w198) -> ()  [unwired: 8 in, 2 out]
        }
        frame #6 {
          w220 = -0.7 ("Left axis value")
          n102 = call <vilib>:"WPI_RobotDriveRefNum Registry Get.vi"("refnum name"="RobotDrive") -> ("error out"=w221:errorcluster, "RobotDriveDevRef"=w222:T13)  [unwired: 9 in]
          n103 = call <vilib>:"WPI_RobotDriveTankDrive.vi"("error in (no error)"=w221, "Right axis value"=w220, "Left axis value"=w220, "RobotDriveDevRef"=w222) -> ()  [unwired: 5 in, 3 out]
          n104 = Wait (ms)(milliseconds to wait=1000) -> ()  [unwired: 1 out]
        }
        frame #7 {
          w228 = 0.0 ("Left axis value")
          n105 = call <vilib>:"WPI_RobotDriveRefNum Registry Get.vi"("refnum name"="RobotDrive") -> ("error out"=w229:errorcluster, "RobotDriveDevRef"=w230:T13)  [unwired: 9 in]
          n106 = call <vilib>:"WPI_SolenoidRefNum Registry Get.vi"("refnum name"="GearGate") -> ("error out"=w226:errorcluster, "SolenoidDevRef"=w225:T5)  [unwired: 9 in]
          n107 = call <vilib>:"WPI_RobotDriveTankDrive.vi"("error in (no error)"=w229, "Right axis value"=w228, "Left axis value"=w228, "RobotDriveDevRef"=w230) -> ()  [unwired: 5 in, 3 out]
          n108 = call-poly <vilib>:"WPI_SolenoidSet.vi"("error in (no error)"=w226, "Value"=WPI_SolenoidValue."Off", "SolenoidDevRef"=w225) -> ()  [unwired: 7 in, 2 out]
        }
        frame #8 {
          n109 = call "Z900_navX_RefNum_Get.vi"("refnum name"="navX") -> ("error out"=w235:errorcluster, "navX Device"=w236:T11)  [unwired: 9 in]
          n110 = call "Z900_navX_Set_ZeroYaw.vi"("error in (no error)"=w235, "navX Device"=w236) -> ("error out"=w232:errorcluster, "navX Device"=w233:T11)  [unwired: 8 in]
          n111 = call <vilib>:"WPI_SolenoidRefNum Registry Get.vi"("refnum name"="GearGate") -> ("error out"=w240:errorcluster, "SolenoidDevRef"=w239:T5)  [unwired: 9 in]
          n112 = call-poly <vilib>:"WPI_SolenoidSet.vi"("error in (no error)"=w240, "Value"=WPI_SolenoidValue."On", "SolenoidDevRef"=w239) -> ()  [unwired: 7 in, 2 out]
          n113 = while {
            tunnel: w233 -> [w250]
            tunnel: w232 -> [w249]
            tunnel: w231 -> [_]
            i -> [w254]
            stop <- w251 stop-if-true
            w241 = -0.5
            w267 = 0.0
            n114 = call "Z900_navX_Get_YPRHfH.vi"("error in (no error)"=w249, "navX Device"=w250) -> ("YRPHfH"=w248:T18)  [unwired: 6 in, 3 out]
            n115 = Unbundle By Name(w248) -> ("Yaw"=w247:dbl)
            n116 = Subtract(x=w247, y=-60.0) -> (x-y=w245:dbl)
            n117 = Absolute Value(x=w245) -> (abs(x)=w244:dbl)
            n118 = Subtract(x=w267, y=w241) -> (x-y=w265:dbl)
            n119 = Add(x=w267, y=w241) -> (x+y=w264:dbl)
            n120 = call <vilib>:"WPI_RobotDriveRefNum Registry Get.vi"("refnum name"="RobotDrive") -> ("RobotDriveDevRef"=w269:T13)  [unwired: 9 in, 1 out]
            n121 = Less?(x=w244, y=0.5) -> (x < y?=w242:bool)
            n122 = Greater?(x=w254, y=200) -> (0:w252:bool)
            n123 = call <vilib>:"WPI_SolenoidRefNum Registry Get.vi"("refnum name"="GearGate") -> ("error out"=w261:errorcluster, "SolenoidDevRef"=w260:T5)  [unwired: 9 in]
            n124 = call <vilib>:"WPI_RobotDriveTankDrive.vi"("Right axis value"=w264, "Left axis value"=w265, "RobotDriveDevRef"=w269) -> ()  [unwired: 6 in, 3 out]
            n125 = call-poly <vilib>:"WPI_SolenoidSet.vi"("error in (no error)"=w261, "Value"=WPI_SolenoidValue."On", "SolenoidDevRef"=w260) -> ()  [unwired: 7 in, 2 out]
            n126 = Or(x=w242, y=w252) -> (x .or. y?=w251:bool)
            n127 = Build Array(w265, w264, w247) -> (w262:dbl[])
            n128 = Array To Cluster(array=w262) -> (cluster=→"DriveStraight 6":T1)
            n129 = call <vilib>:"WPI_SolenoidRefNum Registry Get.vi"("refnum name"="Banana") -> ("SolenoidDevRef"=w257:T5)  [unwired: 9 in, 1 out]
            n130 = call-poly <vilib>:"WPI_SolenoidSet.vi"("Value"=WPI_SolenoidValue."On", "SolenoidDevRef"=w257) -> ()  [unwired: 8 in, 2 out]
            n131 = Wait (ms)(milliseconds to wait=10) -> ()  [unwired: 1 out]
          }
        }
        frame #9 {
          n132 = call <vilib>:"WPI_EncoderRefNum Registry Get.vi"("refnum name"="Encoder 1") -> ("error out"=w282:errorcluster, "EncoderDevRef"=w284:T7)  [unwired: 9 in]
          n133 = call <vilib>:"WPI_EncoderRefNum Registry Get.vi"("refnum name"="Encoder 0") -> ("error out"=w283:errorcluster, "EncoderDevRef"=w285:T7)  [unwired: 9 in]
          n134 = call <vilib>:"WPI_SolenoidRefNum Registry Get.vi"("refnum name"="GearGate") -> ("error out"=w281:errorcluster, "SolenoidDevRef"=w280:T5)  [unwired: 9 in]
          n135 = call-poly <vilib>:"NT Read Value.vi"("Default Value"=14.0, "Name"="Circumference") -> ("Numeric"=w271:dbl)  [unwired: 8 in, 1 out]
          n136 = call-poly <vilib>:"WPI_SolenoidSet.vi"("error in (no error)"=w281, "Value"=WPI_SolenoidValue."On", "SolenoidDevRef"=w280) -> ()  [unwired: 7 in, 2 out]
          n137 = call <vilib>:"WPI_EncoderReset.vi"("error in (no error)"=w283, "EncoderDevRef"=w285) -> ("error out"=w276:errorcluster, "EncoderDevRef"=w277:T7)  [unwired: 8 in]
          n138 = call <vilib>:"WPI_EncoderReset.vi"("error in (no error)"=w282, "EncoderDevRef"=w284) -> ("error out"=w274:errorcluster, "EncoderDevRef"=w275:T7)  [unwired: 8 in]
          n139 = while {
            tunnel: w277 -> [w307]
            tunnel: w276 -> [w306]
            tunnel: w275 -> [w305]
            tunnel: w274 -> [w304]
            tunnel: w271 -> [w289]
            tunnel: w270 -> [w288]
            i -> [w294]
            stop <- w290 stop-if-true
            w322 = 0.7
            n140 = call <vilib>:"WPI_EncoderGet.vi"("error in (no error)"=w306, "EncoderDevRef"=w307) -> ("Distance"=w303:dbl)  [unwired: 4 in, 5 out]
            n141 = call <vilib>:"WPI_EncoderGet.vi"("error in (no error)"=w304, "EncoderDevRef"=w305) -> ("Distance"=w302:dbl)  [unwired: 4 in, 5 out]
            n142 = Subtract(x=w303, y=w302) -> (x-y=w316:dbl)
            n143 = Add(x=w303, y=w302) -> (x+y=w301:dbl)
            n144 = call-poly <vilib>:"PID.vi"("output range"=cluster{"output high":dbl, "output low":dbl} {"output high"=0.5, "output low"=-0.5}, "PID gains"=w288, "process variable"=w316, "setpoint"=0.0) -> ("output"=w323:dbl)  [unwired: 6 in, 1 out]
            n145 = Divide(x=w301, y=2.0) -> (x/y=w296:dbl)
            n146 = Subtract(x=w322, y=w323) -> (x-y=w318:dbl)
            n147 = Add(x=w322, y=w323) -> (x+y=w317:dbl)
            n148 = call <vilib>:"WPI_RobotDriveRefNum Registry Get.vi"("refnum name"="RobotDrive") -> ("RobotDriveDevRef"=w325:T13)  [unwired: 9 in, 1 out]
            n149 = Greater?(x=w294, y=400) -> (0:w291:bool)
            n150 = Divide(x=48.0, y=w289) -> (x/y=w298:dbl)
            n151 = call <vilib>:"WPI_SolenoidRefNum Registry Get.vi"("refnum name"="GearGate") -> ("error out"=w314:errorcluster, "SolenoidDevRef"=w313:T5)  [unwired: 9 in]
            n152 = call <vilib>:"WPI_RobotDriveTankDrive.vi"("Right axis value"=w317, "Left axis value"=w318, "RobotDriveDevRef"=w325) -> ()  [unwired: 6 in, 3 out]
            n153 = Multiply(x=w298, y=1024.0) -> (x*y=w295:dbl)
            n154 = Greater Or Equal?(x=w296, y=w295) -> (x >= y?=w292:bool)
            n155 = call-poly <vilib>:"WPI_SolenoidSet.vi"("error in (no error)"=w314, "Value"=WPI_SolenoidValue."On", "SolenoidDevRef"=w313) -> ()  [unwired: 7 in, 2 out]
            n156 = Or(x=w292, y=w291) -> (x .or. y?=w290:bool)
            n157 = Build Array(w318, w317, w316) -> (w315:dbl[])
            n158 = Array To Cluster(array=w315) -> ()  [unwired: 1 out]
            n159 = call <vilib>:"WPI_SolenoidRefNum Registry Get.vi"("refnum name"="Banana") -> ("SolenoidDevRef"=w310:T5)  [unwired: 9 in, 1 out]
            n160 = call-poly <vilib>:"WPI_SolenoidSet.vi"("Value"=WPI_SolenoidValue."On", "SolenoidDevRef"=w310) -> ()  [unwired: 8 in, 2 out]
            n161 = Wait (ms)(milliseconds to wait=10) -> ()  [unwired: 1 out]
          }
        }
      }
    }
    frame "frontGearPathPlanning" {
      n162 = flat-sequence {
        tunnel: [w339] -> w334
        tunnel: w334 -> [w365]
        tunnel: w331 -> [w364]
        tunnel: w332 -> [w363]
        tunnel: w333 -> [w362]
        tunnel: w327 -> [w361]
        tunnel: "YawFactor" -> [w344]
        tunnel: w330 -> [_]
        tunnel: w328 -> [_]
        tunnel: w329 -> [_]
        frame #0 {
          n163 = disable-structure shown="Disabled" {
            frame Disabled {
              n164 = call <vilib>:"WPI_SolenoidRefNum Registry Get.vi"("refnum name"="Banana") -> ("SolenoidDevRef"=w343:T5)  [unwired: 9 in, 1 out]
              n165 = call-poly <vilib>:"WPI_SolenoidSet.vi"("Value"=WPI_SolenoidValue."On", "SolenoidDevRef"=w343) -> ()  [unwired: 8 in, 2 out]
            }
            frame Enabled {
            }
          }
          n166 = call "ReadFile.vi"("Name"="/home/lvuser/rightGear.txt") -> ("Array - Numeric"=w339:dbl[][])
          n167 = global write "Robot Global Data.vi" "PathPlanningv1"(w339) -> ()
          n168 = call <vilib>:"WPI_SolenoidRefNum Registry Get.vi"("refnum name"="GearGate") -> ("error out"=w338:errorcluster, "SolenoidDevRef"=w337:T5)  [unwired: 9 in]
          n169 = call-poly <vilib>:"WPI_SolenoidSet.vi"("error in (no error)"=w338, "Value"=WPI_SolenoidValue."On", "SolenoidDevRef"=w337) -> ()  [unwired: 7 in, 2 out]
        }
        frame #1 {
          # "Position PID or Velocity PID"
          n170 = disable-structure shown="Disabled" {
            frame Disabled {
              n171 = call <vilib>:"WPI_SolenoidRefNum Registry Get.vi"("refnum name"="Banana") -> ("SolenoidDevRef"=w372:T5)  [unwired: 9 in, 1 out]
              n172 = call-poly <vilib>:"WPI_SolenoidSet.vi"("Value"=WPI_SolenoidValue."On", "SolenoidDevRef"=w372) -> ()  [unwired: 8 in, 2 out]
            }
            frame Enabled {
            }
          }
          n173 = call <vilib>:"WPI_EncoderRefNum Registry Get.vi"("refnum name"="Encoder 0") -> ("error out"=w357:errorcluster, "EncoderDevRef"=w356:T7)  [unwired: 9 in]
          n174 = call <vilib>:"WPI_EncoderRefNum Registry Get.vi"("refnum name"="Encoder 1") -> ("error out"=w359:errorcluster, "EncoderDevRef"=w358:T7)  [unwired: 9 in]
          n175 = call "Z900_navX_RefNum_Get.vi"("refnum name"="navX") -> ("error out"=w348:errorcluster, "navX Device"=w349:T11)  [unwired: 9 in]
          n176 = call "Z900_navX_Set_ZeroYaw.vi"("error in (no error)"=w348, "navX Device"=w349) -> ("error out"=w346:errorcluster, "navX Device"=w347:T11)  [unwired: 8 in]
          n177 = call <vilib>:"WPI_EncoderReset.vi"("error in (no error)"=w357, "EncoderDevRef"=w356) -> ("error out"=w353:errorcluster, "EncoderDevRef"=w354:T7)  [unwired: 8 in]
          n178 = call <vilib>:"WPI_EncoderReset.vi"("error in (no error)"=w359, "EncoderDevRef"=w358) -> ("error out"=w352:errorcluster, "EncoderDevRef"=w355:T7)  [unwired: 8 in]
          n179 = Array Size(array=w365) -> (size(s)=w369:i32[])
          n180 = call <vilib>:"WPI_RobotDriveRefNum Registry Get.vi"("refnum name"="RobotDrive") -> ("RobotDriveDevRef"=w366:T13)  [unwired: 9 in, 1 out]
          n181 = Index Array(array=w369, index=0) -> (element=w360:i32)
          n182 = for {
            N: w360 -> [_]
            tunnel: w365 -> [w393]
            tunnel: w361 -> [w390]
            tunnel: w363 -> [w389]
            tunnel: w364 -> [w388]
            tunnel: w366 -> [w387]
            tunnel: w362 -> [w386]
            tunnel: w355 -> [w377]
            tunnel: w354 -> [w376]
            tunnel: w353 -> [w374]
            tunnel: w352 -> [w375]
            tunnel: w347 -> [w385]
            tunnel: w346 -> [w384]
            tunnel: w344 -> [w380]
            i -> [w392]
            n183 = Index Array(array=w393, index (row)=w392) -> (element=w383:dbl[])  [unwired: 1 in]
            n184 = Index Array(array=w383, index=0) -> (element=w379:dbl)
            n185 = Index Array(array=w383, index=1) -> (element=w378:dbl)
            n186 = Index Array(array=w383, index=2) -> (element=w381:dbl)
            n187 = for {
              N: 10 -> [_]
              tunnel: w390 -> [w427]
              tunnel: w389 -> [w438]
              tunnel: w388 -> [w419]
              tunnel: w387 -> [w439]
              tunnel: w386 -> [w428]
              tunnel: w377 -> [w423]
              tunnel: w376 -> [w422]
              tunnel: w374 -> [w421]
              tunnel: w375 -> [w420]
              tunnel: w379 -> [w407]
              tunnel: w378 -> [w406]
              tunnel: w385 -> [w418]
              tunnel: w384 -> [w417]
              tunnel: w381 -> [w413]
              tunnel: w380 -> [w405]
              tunnel: 0.0011393 ("x") -> [w396]
              n188 = call <vilib>:"WPI_EncoderGet.vi"("error in (no error)"=w420, "EncoderDevRef"=w423) -> ("Distance"=w398:dbl)  [unwired: 4 in, 5 out]
              n189 = call <vilib>:"WPI_EncoderGet.vi"("error in (no error)"=w421, "EncoderDevRef"=w422) -> ("Distance"=w397:dbl)  [unwired: 4 in, 5 out]
              n190 = Multiply(x=w396, y=w397) -> (x*y=w424:dbl)
              n191 = Divide(x=w424, y=w428) -> (x/y=w426:dbl)
              n192 = Multiply(x=w396, y=w398) -> (x*y=w425:dbl)
              n193 = Divide(x=w425, y=w428) -> (x/y=w435:dbl)
              n194 = call "Z900_navX_Get_YPRHfH.vi"("error in (no error)"=w417, "navX Device"=w418) -> ("YRPHfH"=w416:T18)  [unwired: 6 in, 3 out]
              n195 = Unbundle By Name(w416) -> ("Yaw"=w414:dbl)
              n196 = call <vilib>:"WPI_SolenoidRefNum Registry Get.vi"("refnum name"="GearGate") -> ("error out"=w434:errorcluster, "SolenoidDevRef"=w433:T5)  [unwired: 9 in]
              n197 = call-poly <vilib>:"WPI_SolenoidSet.vi"("error in (no error)"=w434, "Value"=WPI_SolenoidValue."On", "SolenoidDevRef"=w433) -> ()  [unwired: 7 in, 2 out]
              n198 = Subtract(x=w414, y=w413) -> (x-y=w412:dbl)
              n199 = Multiply(x=1.0 ("Speed"), y=w405) -> (x*y=w409:dbl)
              n200 = Multiply(x=-1.0, y=w412) -> (x*y=w410:dbl)
              n201 = Multiply(x=w409, y=w410) -> (x*y=w403:dbl)
              "YawCorrection" <- w403
              n202 = Add(x=w435, y=w403) -> (x+y=w400:dbl)
              n203 = call-poly <vilib>:"PID.vi"("output range"=w419, "PID gains"=w438, "process variable"=w400, "setpoint"=w407) -> ("output"=w402:dbl)  [unwired: 6 in, 1 out]
              n204 = Multiply(x=w410, y=w405) -> (x*y=w404:dbl)
              n205 = Add(x=w426, y=w404) -> (x+y=w399:dbl)
              n206 = call-poly <vilib>:"PID.vi"("output range"=w419, "PID gains"=w427, "process variable"=w399, "setpoint"=w406) -> ("output"=w401:dbl)  [unwired: 6 in, 1 out]
              n207 = Bundle("output"=w401, w399, "Numeric"=w406) -> (→"Left V 5":cluster{"output":dbl, dbl, "Numeric":dbl})  [unwired: 1 in]
              n208 = call <vilib>:"WPI_RobotDriveTankDrive.vi"("Right axis value"=w401, "Left axis value"=w402, "RobotDriveDevRef"=w439) -> ()  [unwired: 6 in, 3 out]
              n209 = Divide(x=10, y=w428) -> (x/y=w429:dbl)
              n210 = Bundle("Numeric"=w413, "Yaw"=w414) -> (→"Yaw 5":cluster{"Numeric":dbl, "Yaw":dbl})  [unwired: 1 in]
              n211 = Bundle("output"=w402, w400, "Numeric"=w407) -> (→"Right V 5":cluster{"output":dbl, dbl, "Numeric":dbl})  [unwired: 1 in]
              n212 = Wait (ms)(milliseconds to wait=w429) -> ()  [unwired: 1 out]
            }
          }
        }
        frame #2 {
          w441 = 0.0 ("Right axis value")
          n213 = call <vilib>:"WPI_RobotDriveRefNum Registry Get.vi"("refnum name"="RobotDrive") -> ("RobotDriveDevRef"=w442:T13)  [unwired: 9 in, 1 out]
          n214 = call <vilib>:"WPI_RobotDriveTankDrive.vi"("Right axis value"=w441, "Left axis value"=w441, "RobotDriveDevRef"=w442) -> ()  [unwired: 6 in, 3 out]
        }
        frame #3 {
          w451 = 0.0 ("Left axis value")
          n215 = call <vilib>:"WPI_SolenoidRefNum Registry Get.vi"("refnum name"="Banana") -> ("SolenoidDevRef"=w445:T5)  [unwired: 9 in, 1 out]
          n216 = call <vilib>:"WPI_RobotDriveRefNum Registry Get.vi"("refnum name"="RobotDrive") -> ("error out"=w452:errorcluster, "RobotDriveDevRef"=w453:T13)  [unwired: 9 in]
          n217 = call <vilib>:"WPI_SolenoidRefNum Registry Get.vi"("refnum name"="GearGate") -> ("error out"=w449:errorcluster, "SolenoidDevRef"=w448:T5)  [unwired: 9 in]
          n218 = call-poly <vilib>:"WPI_SolenoidSet.vi"("Value"=WPI_SolenoidValue."On", "SolenoidDevRef"=w445) -> ()  [unwired: 8 in, 2 out]
          n219 = call <vilib>:"WPI_RobotDriveTankDrive.vi"("error in (no error)"=w452, "Right axis value"=w451, "Left axis value"=w451, "RobotDriveDevRef"=w453) -> ()  [unwired: 5 in, 3 out]
          n220 = call-poly <vilib>:"WPI_SolenoidSet.vi"("error in (no error)"=w449, "Value"=WPI_SolenoidValue."On", "SolenoidDevRef"=w448) -> ()  [unwired: 7 in, 2 out]
        }
        frame #4 {
          n221 = for {
            N: 3 -> [_]
            n222 = flat-sequence {
              frame #0 {
                n223 = call <vilib>:"WPI_SolenoidRefNum Registry Get.vi"("refnum name"="Gears") -> ("error out"=w466:errorcluster, "SolenoidDevRef"=w465:T5)  [unwired: 9 in]
                n224 = call <vilib>:"WPI_SolenoidRefNum Registry Get.vi"("refnum name"="GearGate") -> ("error out"=w461:errorcluster, "SolenoidDevRef"=w460:T5)  [unwired: 9 in]
                n225 = call-poly <vilib>:"WPI_SolenoidSet.vi"("error in (no error)"=w466, "Value"=WPI_SolenoidValue."On", "SolenoidDevRef"=w465) -> ()  [unwired: 7 in, 2 out]
                n226 = Wait (ms)(milliseconds to wait=166) -> ()  [unwired: 1 out]
                n227 = call-poly <vilib>:"WPI_SolenoidSet.vi"("error in (no error)"=w461, "Value"=WPI_SolenoidValue."On", "SolenoidDevRef"=w460) -> ()  [unwired: 7 in, 2 out]
              }
              frame #1 {
                n228 = call <vilib>:"WPI_SolenoidRefNum Registry Get.vi"("refnum name"="Gears") -> ("error out"=w475:errorcluster, "SolenoidDevRef"=w474:T5)  [unwired: 9 in]
                n229 = call <vilib>:"WPI_SolenoidRefNum Registry Get.vi"("refnum name"="GearGate") -> ("error out"=w470:errorcluster, "SolenoidDevRef"=w469:T5)  [unwired: 9 in]
                n230 = Wait (ms)(milliseconds to wait=166) -> ()  [unwired: 1 out]
                n231 = call-poly <vilib>:"WPI_SolenoidSet.vi"("error in (no error)"=w475, "Value"=WPI_SolenoidValue."Off", "SolenoidDevRef"=w474) -> ()  [unwired: 7 in, 2 out]
                n232 = call-poly <vilib>:"WPI_SolenoidSet.vi"("error in (no error)"=w470, "Value"=WPI_SolenoidValue."On", "SolenoidDevRef"=w469) -> ()  [unwired: 7 in, 2 out]
              }
            }
          }
          n233 = call <vilib>:"WPI_SolenoidRefNum Registry Get.vi"("refnum name"="Banana") -> ("SolenoidDevRef"=w456:T5)  [unwired: 9 in, 1 out]
          n234 = call-poly <vilib>:"WPI_SolenoidSet.vi"("Value"=WPI_SolenoidValue."On", "SolenoidDevRef"=w456) -> ()  [unwired: 8 in, 2 out]
        }
        frame #5 {
          w478 = 0.0 ("Left axis value")
          n235 = call <vilib>:"WPI_RobotDriveRefNum Registry Get.vi"("refnum name"="RobotDrive") -> ("error out"=w479:errorcluster, "RobotDriveDevRef"=w480:T13)  [unwired: 9 in]
          n236 = call <vilib>:"WPI_RobotDriveTankDrive.vi"("error in (no error)"=w479, "Right axis value"=w478, "Left axis value"=w478, "RobotDriveDevRef"=w480) -> ()  [unwired: 5 in, 3 out]
          n237 = Wait (ms)(milliseconds to wait=1000) -> ()  [unwired: 1 out]
        }
        frame #6 {
          w486 = 0.0 ("Left axis value")
          n238 = call <vilib>:"WPI_RobotDriveRefNum Registry Get.vi"("refnum name"="RobotDrive") -> ("error out"=w487:errorcluster, "RobotDriveDevRef"=w488:T13)  [unwired: 9 in]
          n239 = call <vilib>:"WPI_SolenoidRefNum Registry Get.vi"("refnum name"="GearGate") -> ("error out"=w484:errorcluster, "SolenoidDevRef"=w483:T5)  [unwired: 9 in]
          n240 = call <vilib>:"WPI_RobotDriveTankDrive.vi"("error in (no error)"=w487, "Right axis value"=w486, "Left axis value"=w486, "RobotDriveDevRef"=w488) -> ()  [unwired: 5 in, 3 out]
          n241 = call-poly <vilib>:"WPI_SolenoidSet.vi"("error in (no error)"=w484, "Value"=WPI_SolenoidValue."Off", "SolenoidDevRef"=w483) -> ()  [unwired: 7 in, 2 out]
        }
      }
    }
    frame "leftPegPathLoadingZone" {
      n242 = flat-sequence {
        tunnel: [w509] -> w501
        tunnel: w501 -> [w534]
        tunnel: w500 -> [w533]
        tunnel: w499 -> [w532]
        tunnel: w489 -> [w531]
        tunnel: w495 -> [w530]
        tunnel: w498 -> [_]
        tunnel: w497 -> [_]
        tunnel: w496 -> [_]
        tunnel: w494 -> [w602]
        tunnel: w493 -> [w601]
        tunnel: w492 -> [w600]
        tunnel: w491 -> [w699]
        tunnel: [w699] -> w490
        tunnel: w490 -> [w738]
        frame #0 {
          n243 = call <vilib>:"WPI_SolenoidRefNum Registry Get.vi"("refnum name"="Banana") -> ("SolenoidDevRef"=w504:T5)  [unwired: 9 in, 1 out]
          n244 = call-poly <vilib>:"WPI_SolenoidSet.vi"("Value"=WPI_SolenoidValue."On", "SolenoidDevRef"=w504) -> ()  [unwired: 8 in, 2 out]
          n245 = call "ReadFile.vi"("Name"="/home/lvuser/LeftPegPathLoadingZone.txt") -> ("Array - Numeric"=w509:dbl[][])
          n246 = global write "Robot Global Data.vi" "PathPlanningv1"(w509) -> ()
          n247 = call <vilib>:"WPI_SolenoidRefNum Registry Get.vi"("refnum name"="GearGate") -> ("error out"=w508:errorcluster, "SolenoidDevRef"=w507:T5)  [unwired: 9 in]
          n248 = call-poly <vilib>:"WPI_SolenoidSet.vi"("error in (no error)"=w508, "Value"=WPI_SolenoidValue."On", "SolenoidDevRef"=w507) -> ()  [unwired: 7 in, 2 out]
        }
        frame #1 {
          # "Position PID or Velocity PID"
          n249 = call <vilib>:"WPI_SolenoidRefNum Registry Get.vi"("refnum name"="Banana") -> ("SolenoidDevRef"=w529:T5)  [unwired: 9 in, 1 out]
          n250 = call-poly <vilib>:"WPI_SolenoidSet.vi"("Value"=WPI_SolenoidValue."On", "SolenoidDevRef"=w529) -> ()  [unwired: 8 in, 2 out]
          n251 = call <vilib>:"WPI_EncoderRefNum Registry Get.vi"("refnum name"="Encoder 0") -> ("error out"=w523:errorcluster, "EncoderDevRef"=w522:T7)  [unwired: 9 in]
          n252 = call <vilib>:"WPI_EncoderRefNum Registry Get.vi"("refnum name"="Encoder 1") -> ("error out"=w525:errorcluster, "EncoderDevRef"=w524:T7)  [unwired: 9 in]
          n253 = call "Z900_navX_RefNum_Get.vi"("refnum name"="navX") -> ("error out"=w514:errorcluster, "navX Device"=w515:T11)  [unwired: 9 in]
          n254 = call "Z900_navX_Set_ZeroYaw.vi"("error in (no error)"=w514, "navX Device"=w515) -> ("error out"=w512:errorcluster, "navX Device"=w513:T11)  [unwired: 8 in]
          n255 = call <vilib>:"WPI_EncoderReset.vi"("error in (no error)"=w523, "EncoderDevRef"=w522) -> ("error out"=w519:errorcluster, "EncoderDevRef"=w520:T7)  [unwired: 8 in]
          n256 = call <vilib>:"WPI_EncoderReset.vi"("error in (no error)"=w525, "EncoderDevRef"=w524) -> ("error out"=w518:errorcluster, "EncoderDevRef"=w521:T7)  [unwired: 8 in]
          n257 = Array Size(array=w534) -> (size(s)=w538:i32[])
          n258 = call <vilib>:"WPI_RobotDriveRefNum Registry Get.vi"("refnum name"="RobotDrive") -> ("RobotDriveDevRef"=w535:T13)  [unwired: 9 in, 1 out]
          n259 = Index Array(array=w538, index=0) -> (element=w526:i32)
          n260 = for {
            N: w526 -> [_]
            tunnel: w534 -> [w557]
            tunnel: w530 -> [w554]
            tunnel: w532 -> [w553]
            tunnel: w533 -> [w552]
            tunnel: w535 -> [w551]
            tunnel: w531 -> [w550]
            tunnel: w521 -> [w549]
            tunnel: w520 -> [w548]
            tunnel: w519 -> [w547]
            tunnel: w518 -> [w546]
            tunnel: w513 -> [w543]
            tunnel: w512 -> [w542]
            i -> [w556]
            n261 = Index Array(array=w557, index (row)=w556) -> (element=w541:dbl[])  [unwired: 1 in]
            n262 = Index Array(array=w541, index=0) -> (element=w544:dbl)
            n263 = Index Array(array=w541, index=1) -> (element=w545:dbl)
            n264 = Index Array(array=w541, index=2) -> (element=w539:dbl)
            n265 = for {
              N: 10 -> [_]
              tunnel: w554 -> [w581]
              tunnel: w553 -> [w595]
              tunnel: w552 -> [w566]
              tunnel: w551 -> [w596]
              tunnel: w550 -> [w582]
              tunnel: w549 -> [w576]
              tunnel: w548 -> [w575]
              tunnel: w547 -> [w572]
              tunnel: w546 -> [w571]
              tunnel: w544 -> [w570]
              tunnel: w545 -> [w569]
              tunnel: w543 -> [w565]
              tunnel: w542 -> [w564]
              tunnel: w539 -> [w560]
              w577 = 0.0011393 ("x")
              n266 = call <vilib>:"WPI_EncoderGet.vi"("error in (no error)"=w571, "EncoderDevRef"=w576) -> ("Distance"=w573:dbl)  [unwired: 4 in, 5 out]
              n267 = call <vilib>:"WPI_EncoderGet.vi"("error in (no error)"=w572, "EncoderDevRef"=w575) -> ("Distance"=w574:dbl)  [unwired: 4 in, 5 out]
              n268 = Multiply(x=w577, y=w574) -> (x*y=w578:dbl)
              n269 = Divide(x=w578, y=w582) -> (x/y=w580:dbl)
              n270 = Multiply(x=w577, y=w573) -> (x*y=w579:dbl)
              n271 = Divide(x=w579, y=w582) -> (x/y=w592:dbl)
              n272 = call-poly <vilib>:"PID.vi"("output range"=w566, "PID gains"=w595, "process variable"=w592, "setpoint"=w570) -> ("output"=w567:dbl)  [unwired: 6 in, 1 out]
              n273 = call-poly <vilib>:"PID.vi"("output range"=w566, "PID gains"=w581, "process variable"=w580, "setpoint"=w569) -> ("output"=w568:dbl)  [unwired: 6 in, 1 out]
              n274 = call "Z900_navX_Get_YPRHfH.vi"("error in (no error)"=w564, "navX Device"=w565) -> ("YRPHfH"=w563:T18)  [unwired: 6 in, 3 out]
              n275 = Bundle("output"=w568, w580, "Numeric"=w569) -> (→"Left V":cluster{"output":dbl, dbl, "Numeric":dbl})  [unwired: 1 in]
              n276 = Unbundle By Name(w563) -> ("Yaw"=w561:dbl)
              n277 = call <vilib>:"WPI_SolenoidRefNum Registry Get.vi"("refnum name"="GearGate") -> ("error out"=w591:errorcluster, "SolenoidDevRef"=w590:T5)  [unwired: 9 in]
              n278 = call <vilib>:"WPI_RobotDriveTankDrive.vi"("Right axis value"=w568, "Left axis value"=w567, "RobotDriveDevRef"=w596) -> ()  [unwired: 6 in, 3 out]
              n279 = call-poly <vilib>:"WPI_SolenoidSet.vi"("error in (no error)"=w591, "Value"=WPI_SolenoidValue."On", "SolenoidDevRef"=w590) -> ()  [unwired: 7 in, 2 out]
              n280 = Divide(x=10, y=w582) -> (x/y=w583:dbl)
              n281 = call <vilib>:"WPI_SolenoidRefNum Registry Get.vi"("refnum name"="Banana") -> ("SolenoidDevRef"=w587:T5)  [unwired: 9 in, 1 out]
              n282 = Bundle("Numeric"=w560, "Yaw"=w561) -> (→"Yaw":cluster{"Numeric":dbl, "Yaw":dbl})  [unwired: 1 in]
              n283 = Bundle("output"=w567, w592, "Numeric"=w570) -> (→"Right V":cluster{"output":dbl, dbl, "Numeric":dbl})  [unwired: 1 in]
              n284 = Wait (ms)(milliseconds to wait=w583) -> ()  [unwired: 1 out]
              n285 = call-poly <vilib>:"WPI_SolenoidSet.vi"("Value"=WPI_SolenoidValue."On", "SolenoidDevRef"=w587) -> ()  [unwired: 8 in, 2 out]
            }
          }
        }
        frame #2 {
          w598 = 0.0 ("Right axis value")
          n286 = call <vilib>:"WPI_RobotDriveRefNum Registry Get.vi"("refnum name"="RobotDrive") -> ("RobotDriveDevRef"=w599:T13)  [unwired: 9 in, 1 out]
          n287 = call <vilib>:"WPI_RobotDriveTankDrive.vi"("Right axis value"=w598, "Left axis value"=w598, "RobotDriveDevRef"=w599) -> ()  [unwired: 6 in, 3 out]
        }
        frame #3 {
          n288 = for {
            N: 10 -> [_]
            tunnel: w602 -> [w606]
            tunnel: w601 -> [w605]
            tunnel: w600 -> [w604]
            n289 = global read "Robot Global Data.vi" "TargetsFound"() -> (w609:bool)
            n290 = case shown="True" w609 {
              tunnel: [w617 w625] -> w608
              tunnel: [w617 w624] -> w607
              tunnel: w606 -> [_ w620]
              tunnel: w605 -> [_ w619]
              tunnel: w604 -> [_ w618]
              frame False {
                w617 = 0.0
              }
              frame True {
                n291 = global read "Robot Global Data.vi" "Mid"() -> (w628:dbl)
                n292 = Subtract(x=w628, y=w619) -> (x-y=w622:dbl)
                n293 = Absolute Value(x=w622) -> (abs(x)=w627:dbl)
                n294 = Less?(x=w627, y=w618) -> (x < y?=w626:bool)
                n295 = Greater?(x=w622, y=0.0) -> (0:w623:bool)
                n296 = case shown="True" w623 {
                  tunnel: w626 -> [w631 w644]
                  tunnel: [w629 w642] -> w625
                  tunnel: [w630 w643] -> w624
                  tunnel: w620 -> [w632 w641]
                  frame False {
                    n297 = case shown="True" w631 {
                      tunnel: [w637 w640] -> w630
                      tunnel: [w635 w640] -> w629
                      tunnel: w632 -> [w633 w638]
                      frame False {
                        n298 = Multiply(x=w633, y=-1.0) -> (x*y=w637:dbl)
                        n299 = Multiply(x=w633, y=1.2) -> (x*y=w635:dbl)
                      }
                      frame True {
                        n300 = Multiply(x=w638, y=1.2) -> (x*y=w640:dbl)
                      }
                    }
                  }
                  frame True {
                    n301 = case shown="False" w644 {
                      tunnel: [w649 w652] -> w643
                      tunnel: [w647 w652] -> w642
                      tunnel: w641 -> [w645 w650]
                      frame False {
                        n302 = Multiply(x=w645, y=-1.0) -> (x*y=w647:dbl)
                        n303 = Multiply(x=w645, y=1.0) -> (x*y=w649:dbl)
                      }
                      frame True {
                        n304 = Multiply(x=w650, y=1.0) -> (x*y=w652:dbl)
                      }
                    }
                  }
                }
              }
            }
            n305 = call <vilib>:"WPI_SolenoidRefNum Registry Get.vi"("refnum name"="Banana") -> ("SolenoidDevRef"=w612:T5)  [unwired: 9 in, 1 out]
            n306 = call-poly <vilib>:"WPI_SolenoidSet.vi"("Value"=WPI_SolenoidValue."On", "SolenoidDevRef"=w612) -> ()  [unwired: 8 in, 2 out]
            n307 = call <vilib>:"WPI_RobotDriveRefNum Registry Get.vi"("refnum name"="RobotDrive") -> ("error out"=w615:errorcluster, "RobotDriveDevRef"=w616:T13)  [unwired: 9 in]
            n308 = Wait (ms)(milliseconds to wait=100) -> ()  [unwired: 1 out]
            n309 = call <vilib>:"WPI_RobotDriveTankDrive.vi"("error in (no error)"=w615, "Right axis value"=w608, "Left axis value"=w607, "RobotDriveDevRef"=w616) -> ()  [unwired: 5 in, 3 out]
          }
        }
        frame #4 {
          w661 = 0.0 ("Left axis value")
          n310 = call <vilib>:"WPI_SolenoidRefNum Registry Get.vi"("refnum name"="Banana") -> ("SolenoidDevRef"=w655:T5)  [unwired: 9 in, 1 out]
          n311 = call <vilib>:"WPI_RobotDriveRefNum Registry Get.vi"("refnum name"="RobotDrive") -> ("error out"=w662:errorcluster, "RobotDriveDevRef"=w663:T13)  [unwired: 9 in]
          n312 = call <vilib>:"WPI_SolenoidRefNum Registry Get.vi"("refnum name"="GearGate") -> ("error out"=w659:errorcluster, "SolenoidDevRef"=w658:T5)  [unwired: 9 in]
          n313 = call-poly <vilib>:"WPI_SolenoidSet.vi"("Value"=WPI_SolenoidValue."On", "SolenoidDevRef"=w655) -> ()  [unwired: 8 in, 2 out]
          n314 = call <vilib>:"WPI_RobotDriveTankDrive.vi"("error in (no error)"=w662, "Right axis value"=w661, "Left axis value"=w661, "RobotDriveDevRef"=w663) -> ()  [unwired: 5 in, 3 out]
          n315 = call-poly <vilib>:"WPI_SolenoidSet.vi"("error in (no error)"=w659, "Value"=WPI_SolenoidValue."On", "SolenoidDevRef"=w658) -> ()  [unwired: 7 in, 2 out]
        }
        frame #5 {
          n316 = for {
            N: 3 -> [_]
            n317 = flat-sequence {
              frame #0 {
                n318 = call <vilib>:"WPI_SolenoidRefNum Registry Get.vi"("refnum name"="Gears") -> ("error out"=w676:errorcluster, "SolenoidDevRef"=w675:T5)  [unwired: 9 in]
                n319 = call <vilib>:"WPI_SolenoidRefNum Registry Get.vi"("refnum name"="GearGate") -> ("error out"=w671:errorcluster, "SolenoidDevRef"=w670:T5)  [unwired: 9 in]
                n320 = call-poly <vilib>:"WPI_SolenoidSet.vi"("error in (no error)"=w676, "Value"=WPI_SolenoidValue."On", "SolenoidDevRef"=w675) -> ()  [unwired: 7 in, 2 out]
                n321 = Wait (ms)(milliseconds to wait=166) -> ()  [unwired: 1 out]
                n322 = call-poly <vilib>:"WPI_SolenoidSet.vi"("error in (no error)"=w671, "Value"=WPI_SolenoidValue."On", "SolenoidDevRef"=w670) -> ()  [unwired: 7 in, 2 out]
              }
              frame #1 {
                n323 = call <vilib>:"WPI_SolenoidRefNum Registry Get.vi"("refnum name"="Gears") -> ("error out"=w685:errorcluster, "SolenoidDevRef"=w684:T5)  [unwired: 9 in]
                n324 = call <vilib>:"WPI_SolenoidRefNum Registry Get.vi"("refnum name"="GearGate") -> ("error out"=w680:errorcluster, "SolenoidDevRef"=w679:T5)  [unwired: 9 in]
                n325 = Wait (ms)(milliseconds to wait=166) -> ()  [unwired: 1 out]
                n326 = call-poly <vilib>:"WPI_SolenoidSet.vi"("error in (no error)"=w685, "Value"=WPI_SolenoidValue."Off", "SolenoidDevRef"=w684) -> ()  [unwired: 7 in, 2 out]
                n327 = call-poly <vilib>:"WPI_SolenoidSet.vi"("error in (no error)"=w680, "Value"=WPI_SolenoidValue."On", "SolenoidDevRef"=w679) -> ()  [unwired: 7 in, 2 out]
              }
            }
          }
          n328 = call <vilib>:"WPI_SolenoidRefNum Registry Get.vi"("refnum name"="Banana") -> ("SolenoidDevRef"=w666:T5)  [unwired: 9 in, 1 out]
          n329 = call-poly <vilib>:"WPI_SolenoidSet.vi"("Value"=WPI_SolenoidValue."On", "SolenoidDevRef"=w666) -> ()  [unwired: 8 in, 2 out]
        }
        frame #6 {
          w688 = -0.7 ("Left axis value")
          n330 = call <vilib>:"WPI_RobotDriveRefNum Registry Get.vi"("refnum name"="RobotDrive") -> ("error out"=w689:errorcluster, "RobotDriveDevRef"=w690:T13)  [unwired: 9 in]
          n331 = call <vilib>:"WPI_RobotDriveTankDrive.vi"("error in (no error)"=w689, "Right axis value"=w688, "Left axis value"=w688, "RobotDriveDevRef"=w690) -> ()  [unwired: 5 in, 3 out]
          n332 = Wait (ms)(milliseconds to wait=1000) -> ()  [unwired: 1 out]
        }
        frame #7 {
          w696 = 0.0 ("Left axis value")
          n333 = call <vilib>:"WPI_RobotDriveRefNum Registry Get.vi"("refnum name"="RobotDrive") -> ("error out"=w697:errorcluster, "RobotDriveDevRef"=w698:T13)  [unwired: 9 in]
          n334 = call <vilib>:"WPI_SolenoidRefNum Registry Get.vi"("refnum name"="GearGate") -> ("error out"=w694:errorcluster, "SolenoidDevRef"=w693:T5)  [unwired: 9 in]
          n335 = call <vilib>:"WPI_RobotDriveTankDrive.vi"("error in (no error)"=w697, "Right axis value"=w696, "Left axis value"=w696, "RobotDriveDevRef"=w698) -> ()  [unwired: 5 in, 3 out]
          n336 = call-poly <vilib>:"WPI_SolenoidSet.vi"("error in (no error)"=w694, "Value"=WPI_SolenoidValue."Off", "SolenoidDevRef"=w693) -> ()  [unwired: 7 in, 2 out]
        }
        frame #8 {
          n337 = call "Z900_navX_RefNum_Get.vi"("refnum name"="navX") -> ("error out"=w703:errorcluster, "navX Device"=w704:T11)  [unwired: 9 in]
          n338 = call "Z900_navX_Set_ZeroYaw.vi"("error in (no error)"=w703, "navX Device"=w704) -> ("error out"=w700:errorcluster, "navX Device"=w701:T11)  [unwired: 8 in]
          n339 = call <vilib>:"WPI_SolenoidRefNum Registry Get.vi"("refnum name"="GearGate") -> ("error out"=w708:errorcluster, "SolenoidDevRef"=w707:T5)  [unwired: 9 in]
          n340 = call-poly <vilib>:"WPI_SolenoidSet.vi"("error in (no error)"=w708, "Value"=WPI_SolenoidValue."On", "SolenoidDevRef"=w707) -> ()  [unwired: 7 in, 2 out]
          n341 = while {
            tunnel: w701 -> [w718]
            tunnel: w700 -> [w717]
            tunnel: w699 -> [_]
            i -> [w722]
            stop <- w719 stop-if-true
            w709 = -0.5
            w735 = 0.0
            n342 = call "Z900_navX_Get_YPRHfH.vi"("error in (no error)"=w717, "navX Device"=w718) -> ("YRPHfH"=w716:T18)  [unwired: 6 in, 3 out]
            n343 = Unbundle By Name(w716) -> ("Yaw"=w715:dbl)
            n344 = Subtract(x=w715, y=-60.0) -> (x-y=w713:dbl)
            n345 = Absolute Value(x=w713) -> (abs(x)=w712:dbl)
            n346 = Subtract(x=w735, y=w709) -> (x-y=w733:dbl)
            n347 = Add(x=w735, y=w709) -> (x+y=w732:dbl)
            n348 = call <vilib>:"WPI_RobotDriveRefNum Registry Get.vi"("refnum name"="RobotDrive") -> ("RobotDriveDevRef"=w737:T13)  [unwired: 9 in, 1 out]
            n349 = Less?(x=w712, y=0.5) -> (x < y?=w710:bool)
            n350 = Greater?(x=w722, y=200) -> (0:w720:bool)
            n351 = call <vilib>:"WPI_SolenoidRefNum Registry Get.vi"("refnum name"="GearGate") -> ("error out"=w729:errorcluster, "SolenoidDevRef"=w728:T5)  [unwired: 9 in]
            n352 = call <vilib>:"WPI_RobotDriveTankDrive.vi"("Right axis value"=w732, "Left axis value"=w733, "RobotDriveDevRef"=w737) -> ()  [unwired: 6 in, 3 out]
            n353 = call-poly <vilib>:"WPI_SolenoidSet.vi"("error in (no error)"=w729, "Value"=WPI_SolenoidValue."On", "SolenoidDevRef"=w728) -> ()  [unwired: 7 in, 2 out]
            n354 = Or(x=w710, y=w720) -> (x .or. y?=w719:bool)
            n355 = Build Array(w733, w732, w715) -> (w730:dbl[])
            n356 = Array To Cluster(array=w730) -> (cluster=→"DriveStraight 4":T1)
            n357 = call <vilib>:"WPI_SolenoidRefNum Registry Get.vi"("refnum name"="Banana") -> ("SolenoidDevRef"=w725:T5)  [unwired: 9 in, 1 out]
            n358 = call-poly <vilib>:"WPI_SolenoidSet.vi"("Value"=WPI_SolenoidValue."On", "SolenoidDevRef"=w725) -> ()  [unwired: 8 in, 2 out]
            n359 = Wait (ms)(milliseconds to wait=10) -> ()  [unwired: 1 out]
          }
        }
        frame #9 {
          n360 = call <vilib>:"WPI_EncoderRefNum Registry Get.vi"("refnum name"="Encoder 1") -> ("error out"=w750:errorcluster, "EncoderDevRef"=w752:T7)  [unwired: 9 in]
          n361 = call <vilib>:"WPI_EncoderRefNum Registry Get.vi"("refnum name"="Encoder 0") -> ("error out"=w751:errorcluster, "EncoderDevRef"=w753:T7)  [unwired: 9 in]
          n362 = call <vilib>:"WPI_SolenoidRefNum Registry Get.vi"("refnum name"="GearGate") -> ("error out"=w749:errorcluster, "SolenoidDevRef"=w748:T5)  [unwired: 9 in]
          n363 = call-poly <vilib>:"NT Read Value.vi"("Default Value"=14.0, "Name"="Circumference") -> ("Numeric"=w739:dbl)  [unwired: 8 in, 1 out]
          n364 = call-poly <vilib>:"WPI_SolenoidSet.vi"("error in (no error)"=w749, "Value"=WPI_SolenoidValue."On", "SolenoidDevRef"=w748) -> ()  [unwired: 7 in, 2 out]
          n365 = call <vilib>:"WPI_EncoderReset.vi"("error in (no error)"=w751, "EncoderDevRef"=w753) -> ("error out"=w744:errorcluster, "EncoderDevRef"=w745:T7)  [unwired: 8 in]
          n366 = call <vilib>:"WPI_EncoderReset.vi"("error in (no error)"=w750, "EncoderDevRef"=w752) -> ("error out"=w742:errorcluster, "EncoderDevRef"=w743:T7)  [unwired: 8 in]
          n367 = while {
            tunnel: w745 -> [w775]
            tunnel: w744 -> [w774]
            tunnel: w743 -> [w773]
            tunnel: w742 -> [w772]
            tunnel: w739 -> [w757]
            tunnel: w738 -> [w756]
            i -> [w762]
            stop <- w758 stop-if-true
            w790 = 0.7
            n368 = call <vilib>:"WPI_EncoderGet.vi"("error in (no error)"=w774, "EncoderDevRef"=w775) -> ("Distance"=w771:dbl)  [unwired: 4 in, 5 out]
            n369 = call <vilib>:"WPI_EncoderGet.vi"("error in (no error)"=w772, "EncoderDevRef"=w773) -> ("Distance"=w770:dbl)  [unwired: 4 in, 5 out]
            n370 = Subtract(x=w771, y=w770) -> (x-y=w784:dbl)
            n371 = Add(x=w771, y=w770) -> (x+y=w769:dbl)
            n372 = call-poly <vilib>:"PID.vi"("output range"=cluster{"output high":dbl, "output low":dbl} {"output high"=0.5, "output low"=-0.5}, "PID gains"=w756, "process variable"=w784, "setpoint"=0.0) -> ("output"=w791:dbl)  [unwired: 6 in, 1 out]
            n373 = Divide(x=w769, y=2.0) -> (x/y=w764:dbl)
            n374 = Subtract(x=w790, y=w791) -> (x-y=w786:dbl)
            n375 = Add(x=w790, y=w791) -> (x+y=w785:dbl)
            n376 = call <vilib>:"WPI_RobotDriveRefNum Registry Get.vi"("refnum name"="RobotDrive") -> ("RobotDriveDevRef"=w793:T13)  [unwired: 9 in, 1 out]
            n377 = Greater?(x=w762, y=400) -> (0:w759:bool)
            n378 = Divide(x=48.0, y=w757) -> (x/y=w766:dbl)
            n379 = call <vilib>:"WPI_SolenoidRefNum Registry Get.vi"("refnum name"="GearGate") -> ("error out"=w782:errorcluster, "SolenoidDevRef"=w781:T5)  [unwired: 9 in]
            n380 = call <vilib>:"WPI_RobotDriveTankDrive.vi"("Right axis value"=w785, "Left axis value"=w786, "RobotDriveDevRef"=w793) -> ()  [unwired: 6 in, 3 out]
            n381 = Multiply(x=w766, y=1024.0) -> (x*y=w763:dbl)
            n382 = Greater Or Equal?(x=w764, y=w763) -> (x >= y?=w760:bool)
            n383 = call-poly <vilib>:"WPI_SolenoidSet.vi"("error in (no error)"=w782, "Value"=WPI_SolenoidValue."On", "SolenoidDevRef"=w781) -> ()  [unwired: 7 in, 2 out]
            n384 = Or(x=w760, y=w759) -> (x .or. y?=w758:bool)
            n385 = Build Array(w786, w785, w784) -> (w783:dbl[])
            n386 = Array To Cluster(array=w783) -> ()  [unwired: 1 out]
            n387 = call <vilib>:"WPI_SolenoidRefNum Registry Get.vi"("refnum name"="Banana") -> ("SolenoidDevRef"=w778:T5)  [unwired: 9 in, 1 out]
            n388 = call-poly <vilib>:"WPI_SolenoidSet.vi"("Value"=WPI_SolenoidValue."On", "SolenoidDevRef"=w778) -> ()  [unwired: 8 in, 2 out]
            n389 = Wait (ms)(milliseconds to wait=10) -> ()  [unwired: 1 out]
          }
        }
      }
    }
    frame "RightPegPathLoadingZone" {
      n390 = flat-sequence {
        tunnel: [w814] -> w806
        tunnel: w806 -> [w839]
        tunnel: w805 -> [w838]
        tunnel: w804 -> [w837]
        tunnel: w800 -> [w836]
        tunnel: w799 -> [w835]
        tunnel: w803 -> [_]
        tunnel: w802 -> [_]
        tunnel: w801 -> [_]
        tunnel: w798 -> [w907]
        tunnel: w797 -> [w906]
        tunnel: w796 -> [w905]
        tunnel: w795 -> [w1004]
        tunnel: [w1004] -> w794
        tunnel: w794 -> [w1043]
        frame #0 {
          n391 = call <vilib>:"WPI_SolenoidRefNum Registry Get.vi"("refnum name"="Banana") -> ("SolenoidDevRef"=w809:T5)  [unwired: 9 in, 1 out]
          n392 = call-poly <vilib>:"WPI_SolenoidSet.vi"("Value"=WPI_SolenoidValue."On", "SolenoidDevRef"=w809) -> ()  [unwired: 8 in, 2 out]
          n393 = call "ReadFile.vi"("Name"="/home/lvuser/RightPegPathLoadingZone.txt") -> ("Array - Numeric"=w814:dbl[][])
          n394 = global write "Robot Global Data.vi" "PathPlanningv1"(w814) -> ()
          n395 = call <vilib>:"WPI_SolenoidRefNum Registry Get.vi"("refnum name"="GearGate") -> ("error out"=w813:errorcluster, "SolenoidDevRef"=w812:T5)  [unwired: 9 in]
          n396 = call-poly <vilib>:"WPI_SolenoidSet.vi"("error in (no error)"=w813, "Value"=WPI_SolenoidValue."On", "SolenoidDevRef"=w812) -> ()  [unwired: 7 in, 2 out]
        }
        frame #1 {
          # "Position PID or Velocity PID"
          n397 = call <vilib>:"WPI_SolenoidRefNum Registry Get.vi"("refnum name"="Banana") -> ("SolenoidDevRef"=w834:T5)  [unwired: 9 in, 1 out]
          n398 = call-poly <vilib>:"WPI_SolenoidSet.vi"("Value"=WPI_SolenoidValue."On", "SolenoidDevRef"=w834) -> ()  [unwired: 8 in, 2 out]
          n399 = call <vilib>:"WPI_EncoderRefNum Registry Get.vi"("refnum name"="Encoder 0") -> ("error out"=w828:errorcluster, "EncoderDevRef"=w827:T7)  [unwired: 9 in]
          n400 = call <vilib>:"WPI_EncoderRefNum Registry Get.vi"("refnum name"="Encoder 1") -> ("error out"=w830:errorcluster, "EncoderDevRef"=w829:T7)  [unwired: 9 in]
          n401 = call "Z900_navX_RefNum_Get.vi"("refnum name"="navX") -> ("error out"=w819:errorcluster, "navX Device"=w820:T11)  [unwired: 9 in]
          n402 = call "Z900_navX_Set_ZeroYaw.vi"("error in (no error)"=w819, "navX Device"=w820) -> ("error out"=w817:errorcluster, "navX Device"=w818:T11)  [unwired: 8 in]
          n403 = call <vilib>:"WPI_EncoderReset.vi"("error in (no error)"=w828, "EncoderDevRef"=w827) -> ("error out"=w824:errorcluster, "EncoderDevRef"=w825:T7)  [unwired: 8 in]
          n404 = call <vilib>:"WPI_EncoderReset.vi"("error in (no error)"=w830, "EncoderDevRef"=w829) -> ("error out"=w823:errorcluster, "EncoderDevRef"=w826:T7)  [unwired: 8 in]
          n405 = Array Size(array=w839) -> (size(s)=w843:i32[])
          n406 = call <vilib>:"WPI_RobotDriveRefNum Registry Get.vi"("refnum name"="RobotDrive") -> ("RobotDriveDevRef"=w840:T13)  [unwired: 9 in, 1 out]
          n407 = Index Array(array=w843, index=0) -> (element=w831:i32)
          n408 = for {
            N: w831 -> [_]
            tunnel: w839 -> [w862]
            tunnel: w835 -> [w859]
            tunnel: w837 -> [w858]
            tunnel: w838 -> [w857]
            tunnel: w840 -> [w856]
            tunnel: w836 -> [w855]
            tunnel: w826 -> [w854]
            tunnel: w825 -> [w853]
            tunnel: w824 -> [w852]
            tunnel: w823 -> [w851]
            tunnel: w818 -> [w848]
            tunnel: w817 -> [w847]
            i -> [w861]
            n409 = Index Array(array=w862, index (row)=w861) -> (element=w846:dbl[])  [unwired: 1 in]
            n410 = Index Array(array=w846, index=0) -> (element=w849:dbl)
            n411 = Index Array(array=w846, index=1) -> (element=w850:dbl)
            n412 = Index Array(array=w846, index=2) -> (element=w844:dbl)
            n413 = for {
              N: 10 -> [_]
              tunnel: w859 -> [w886]
              tunnel: w858 -> [w900]
              tunnel: w857 -> [w871]
              tunnel: w856 -> [w901]
              tunnel: w855 -> [w887]
              tunnel: w854 -> [w881]
              tunnel: w853 -> [w880]
              tunnel: w852 -> [w877]
              tunnel: w851 -> [w876]
              tunnel: w849 -> [w875]
              tunnel: w850 -> [w874]
              tunnel: w848 -> [w870]
              tunnel: w847 -> [w869]
              tunnel: w844 -> [w865]
              w882 = 0.0011393 ("x")
              n414 = call <vilib>:"WPI_EncoderGet.vi"("error in (no error)"=w876, "EncoderDevRef"=w881) -> ("Distance"=w878:dbl)  [unwired: 4 in, 5 out]
              n415 = call <vilib>:"WPI_EncoderGet.vi"("error in (no error)"=w877, "EncoderDevRef"=w880) -> ("Distance"=w879:dbl)  [unwired: 4 in, 5 out]
              n416 = Multiply(x=w882, y=w879) -> (x*y=w883:dbl)
              n417 = Divide(x=w883, y=w887) -> (x/y=w885:dbl)
              n418 = Multiply(x=w882, y=w878) -> (x*y=w884:dbl)
              n419 = Divide(x=w884, y=w887) -> (x/y=w897:dbl)
              n420 = call-poly <vilib>:"PID.vi"("output range"=w871, "PID gains"=w900, "process variable"=w897, "setpoint"=w875) -> ("output"=w872:dbl)  [unwired: 6 in, 1 out]
              n421 = call-poly <vilib>:"PID.vi"("output range"=w871, "PID gains"=w886, "process variable"=w885, "setpoint"=w874) -> ("output"=w873:dbl)  [unwired: 6 in, 1 out]
              n422 = call "Z900_navX_Get_YPRHfH.vi"("error in (no error)"=w869, "navX Device"=w870) -> ("YRPHfH"=w868:T18)  [unwired: 6 in, 3 out]
              n423 = Bundle("output"=w873, w885, "Numeric"=w874) -> (→"Left V 2":cluster{"output":dbl, dbl, "Numeric":dbl})  [unwired: 1 in]
              n424 = Unbundle By Name(w868) -> ("Yaw"=w866:dbl)
              n425 = call <vilib>:"WPI_SolenoidRefNum Registry Get.vi"("refnum name"="GearGate") -> ("error out"=w896:errorcluster, "SolenoidDevRef"=w895:T5)  [unwired: 9 in]
              n426 = call <vilib>:"WPI_RobotDriveTankDrive.vi"("Right axis value"=w873, "Left axis value"=w872, "RobotDriveDevRef"=w901) -> ()  [unwired: 6 in, 3 out]
              n427 = call-poly <vilib>:"WPI_SolenoidSet.vi"("error in (no error)"=w896, "Value"=WPI_SolenoidValue."On", "SolenoidDevRef"=w895) -> ()  [unwired: 7 in, 2 out]
              n428 = Divide(x=10, y=w887) -> (x/y=w888:dbl)
              n429 = call <vilib>:"WPI_SolenoidRefNum Registry Get.vi"("refnum name"="Banana") -> ("SolenoidDevRef"=w892:T5)  [unwired: 9 in, 1 out]
              n430 = Bundle("Numeric"=w865, "Yaw"=w866) -> (→"Yaw 2":cluster{"Numeric":dbl, "Yaw":dbl})  [unwired: 1 in]
              n431 = Bundle("output"=w872, w897, "Numeric"=w875) -> (→"Right V 2":cluster{"output":dbl, dbl, "Numeric":dbl})  [unwired: 1 in]
              n432 = Wait (ms)(milliseconds to wait=w888) -> ()  [unwired: 1 out]
              n433 = call-poly <vilib>:"WPI_SolenoidSet.vi"("Value"=WPI_SolenoidValue."On", "SolenoidDevRef"=w892) -> ()  [unwired: 8 in, 2 out]
            }
          }
        }
        frame #2 {
          w903 = 0.0 ("Right axis value")
          n434 = call <vilib>:"WPI_RobotDriveRefNum Registry Get.vi"("refnum name"="RobotDrive") -> ("RobotDriveDevRef"=w904:T13)  [unwired: 9 in, 1 out]
          n435 = call <vilib>:"WPI_RobotDriveTankDrive.vi"("Right axis value"=w903, "Left axis value"=w903, "RobotDriveDevRef"=w904) -> ()  [unwired: 6 in, 3 out]
        }
        frame #3 {
          n436 = for {
            N: 10 -> [_]
            tunnel: w907 -> [w911]
            tunnel: w906 -> [w910]
            tunnel: w905 -> [w909]
            n437 = global read "Robot Global Data.vi" "TargetsFound"() -> (w914:bool)
            n438 = case shown="False" w914 {
              tunnel: [w922 w930] -> w913
              tunnel: [w922 w929] -> w912
              tunnel: w911 -> [_ w925]
              tunnel: w910 -> [_ w924]
              tunnel: w909 -> [_ w923]
              frame False {
                w922 = 0.0
              }
              frame True {
                n439 = global read "Robot Global Data.vi" "Mid"() -> (w933:dbl)
                n440 = Subtract(x=w933, y=w924) -> (x-y=w927:dbl)
                n441 = Absolute Value(x=w927) -> (abs(x)=w932:dbl)
                n442 = Less?(x=w932, y=w923) -> (x < y?=w931:bool)
                n443 = Greater?(x=w927, y=0.0) -> (0:w928:bool)
                n444 = case shown="True" w928 {
                  tunnel: w931 -> [w936 w949]
                  tunnel: [w934 w947] -> w930
                  tunnel: [w935 w948] -> w929
                  tunnel: w925 -> [w937 w946]
                  frame False {
                    n445 = case shown="True" w936 {
                      tunnel: [w942 w945] -> w935
                      tunnel: [w940 w945] -> w934
                      tunnel: w937 -> [w938 w943]
                      frame False {
                        n446 = Multiply(x=w938, y=-1.0) -> (x*y=w942:dbl)
                        n447 = Multiply(x=w938, y=1.2) -> (x*y=w940:dbl)
                      }
                      frame True {
                        n448 = Multiply(x=w943, y=1.2) -> (x*y=w945:dbl)
                      }
                    }
                  }
                  frame True {
                    n449 = case shown="False" w949 {
                      tunnel: [w954 w957] -> w948
                      tunnel: [w952 w957] -> w947
                      tunnel: w946 -> [w950 w955]
                      frame False {
                        n450 = Multiply(x=w950, y=-1.0) -> (x*y=w952:dbl)
                        n451 = Multiply(x=w950, y=1.0) -> (x*y=w954:dbl)
                      }
                      frame True {
                        n452 = Multiply(x=w955, y=1.0) -> (x*y=w957:dbl)
                      }
                    }
                  }
                }
              }
            }
            n453 = call <vilib>:"WPI_SolenoidRefNum Registry Get.vi"("refnum name"="Banana") -> ("SolenoidDevRef"=w917:T5)  [unwired: 9 in, 1 out]
            n454 = call-poly <vilib>:"WPI_SolenoidSet.vi"("Value"=WPI_SolenoidValue."On", "SolenoidDevRef"=w917) -> ()  [unwired: 8 in, 2 out]
            n455 = call <vilib>:"WPI_RobotDriveRefNum Registry Get.vi"("refnum name"="RobotDrive") -> ("error out"=w920:errorcluster, "RobotDriveDevRef"=w921:T13)  [unwired: 9 in]
            n456 = Wait (ms)(milliseconds to wait=100) -> ()  [unwired: 1 out]
            n457 = call <vilib>:"WPI_RobotDriveTankDrive.vi"("error in (no error)"=w920, "Right axis value"=w913, "Left axis value"=w912, "RobotDriveDevRef"=w921) -> ()  [unwired: 5 in, 3 out]
          }
        }
        frame #4 {
          w966 = 0.0 ("Left axis value")
          n458 = call <vilib>:"WPI_SolenoidRefNum Registry Get.vi"("refnum name"="Banana") -> ("SolenoidDevRef"=w960:T5)  [unwired: 9 in, 1 out]
          n459 = call <vilib>:"WPI_RobotDriveRefNum Registry Get.vi"("refnum name"="RobotDrive") -> ("error out"=w967:errorcluster, "RobotDriveDevRef"=w968:T13)  [unwired: 9 in]
          n460 = call <vilib>:"WPI_SolenoidRefNum Registry Get.vi"("refnum name"="GearGate") -> ("error out"=w964:errorcluster, "SolenoidDevRef"=w963:T5)  [unwired: 9 in]
          n461 = call-poly <vilib>:"WPI_SolenoidSet.vi"("Value"=WPI_SolenoidValue."On", "SolenoidDevRef"=w960) -> ()  [unwired: 8 in, 2 out]
          n462 = call <vilib>:"WPI_RobotDriveTankDrive.vi"("error in (no error)"=w967, "Right axis value"=w966, "Left axis value"=w966, "RobotDriveDevRef"=w968) -> ()  [unwired: 5 in, 3 out]
          n463 = call-poly <vilib>:"WPI_SolenoidSet.vi"("error in (no error)"=w964, "Value"=WPI_SolenoidValue."On", "SolenoidDevRef"=w963) -> ()  [unwired: 7 in, 2 out]
        }
        frame #5 {
          n464 = for {
            N: 3 -> [_]
            n465 = flat-sequence {
              frame #0 {
                n466 = call <vilib>:"WPI_SolenoidRefNum Registry Get.vi"("refnum name"="Gears") -> ("error out"=w981:errorcluster, "SolenoidDevRef"=w980:T5)  [unwired: 9 in]
                n467 = call <vilib>:"WPI_SolenoidRefNum Registry Get.vi"("refnum name"="GearGate") -> ("error out"=w976:errorcluster, "SolenoidDevRef"=w975:T5)  [unwired: 9 in]
                n468 = call-poly <vilib>:"WPI_SolenoidSet.vi"("error in (no error)"=w981, "Value"=WPI_SolenoidValue."On", "SolenoidDevRef"=w980) -> ()  [unwired: 7 in, 2 out]
                n469 = Wait (ms)(milliseconds to wait=166) -> ()  [unwired: 1 out]
                n470 = call-poly <vilib>:"WPI_SolenoidSet.vi"("error in (no error)"=w976, "Value"=WPI_SolenoidValue."On", "SolenoidDevRef"=w975) -> ()  [unwired: 7 in, 2 out]
              }
              frame #1 {
                n471 = call <vilib>:"WPI_SolenoidRefNum Registry Get.vi"("refnum name"="Gears") -> ("error out"=w990:errorcluster, "SolenoidDevRef"=w989:T5)  [unwired: 9 in]
                n472 = call <vilib>:"WPI_SolenoidRefNum Registry Get.vi"("refnum name"="GearGate") -> ("error out"=w985:errorcluster, "SolenoidDevRef"=w984:T5)  [unwired: 9 in]
                n473 = Wait (ms)(milliseconds to wait=166) -> ()  [unwired: 1 out]
                n474 = call-poly <vilib>:"WPI_SolenoidSet.vi"("error in (no error)"=w990, "Value"=WPI_SolenoidValue."Off", "SolenoidDevRef"=w989) -> ()  [unwired: 7 in, 2 out]
                n475 = call-poly <vilib>:"WPI_SolenoidSet.vi"("error in (no error)"=w985, "Value"=WPI_SolenoidValue."On", "SolenoidDevRef"=w984) -> ()  [unwired: 7 in, 2 out]
              }
            }
          }
          n476 = call <vilib>:"WPI_SolenoidRefNum Registry Get.vi"("refnum name"="Banana") -> ("SolenoidDevRef"=w971:T5)  [unwired: 9 in, 1 out]
          n477 = call-poly <vilib>:"WPI_SolenoidSet.vi"("Value"=WPI_SolenoidValue."On", "SolenoidDevRef"=w971) -> ()  [unwired: 8 in, 2 out]
        }
        frame #6 {
          w993 = -0.7 ("Left axis value")
          n478 = call <vilib>:"WPI_RobotDriveRefNum Registry Get.vi"("refnum name"="RobotDrive") -> ("error out"=w994:errorcluster, "RobotDriveDevRef"=w995:T13)  [unwired: 9 in]
          n479 = call <vilib>:"WPI_RobotDriveTankDrive.vi"("error in (no error)"=w994, "Right axis value"=w993, "Left axis value"=w993, "RobotDriveDevRef"=w995) -> ()  [unwired: 5 in, 3 out]
          n480 = Wait (ms)(milliseconds to wait=1000) -> ()  [unwired: 1 out]
        }
        frame #7 {
          w1001 = 0.0 ("Left axis value")
          n481 = call <vilib>:"WPI_RobotDriveRefNum Registry Get.vi"("refnum name"="RobotDrive") -> ("error out"=w1002:errorcluster, "RobotDriveDevRef"=w1003:T13)  [unwired: 9 in]
          n482 = call <vilib>:"WPI_SolenoidRefNum Registry Get.vi"("refnum name"="GearGate") -> ("error out"=w999:errorcluster, "SolenoidDevRef"=w998:T5)  [unwired: 9 in]
          n483 = call <vilib>:"WPI_RobotDriveTankDrive.vi"("error in (no error)"=w1002, "Right axis value"=w1001, "Left axis value"=w1001, "RobotDriveDevRef"=w1003) -> ()  [unwired: 5 in, 3 out]
          n484 = call-poly <vilib>:"WPI_SolenoidSet.vi"("error in (no error)"=w999, "Value"=WPI_SolenoidValue."Off", "SolenoidDevRef"=w998) -> ()  [unwired: 7 in, 2 out]
        }
        frame #8 {
          n485 = call "Z900_navX_RefNum_Get.vi"("refnum name"="navX") -> ("error out"=w1008:errorcluster, "navX Device"=w1009:T11)  [unwired: 9 in]
          n486 = call "Z900_navX_Set_ZeroYaw.vi"("error in (no error)"=w1008, "navX Device"=w1009) -> ("error out"=w1005:errorcluster, "navX Device"=w1006:T11)  [unwired: 8 in]
          n487 = call <vilib>:"WPI_SolenoidRefNum Registry Get.vi"("refnum name"="GearGate") -> ("error out"=w1013:errorcluster, "SolenoidDevRef"=w1012:T5)  [unwired: 9 in]
          n488 = call-poly <vilib>:"WPI_SolenoidSet.vi"("error in (no error)"=w1013, "Value"=WPI_SolenoidValue."On", "SolenoidDevRef"=w1012) -> ()  [unwired: 7 in, 2 out]
          n489 = while {
            tunnel: w1006 -> [w1023]
            tunnel: w1005 -> [w1022]
            tunnel: w1004 -> [_]
            i -> [w1027]
            stop <- w1024 stop-if-true
            w1014 = 0.5
            w1040 = 0.0
            n490 = call "Z900_navX_Get_YPRHfH.vi"("error in (no error)"=w1022, "navX Device"=w1023) -> ("YRPHfH"=w1021:T18)  [unwired: 6 in, 3 out]
            n491 = Unbundle By Name(w1021) -> ("Yaw"=w1020:dbl)
            n492 = Subtract(x=w1020, y=-60.0) -> (x-y=w1018:dbl)
            n493 = Absolute Value(x=w1018) -> (abs(x)=w1017:dbl)
            n494 = Subtract(x=w1040, y=w1014) -> (x-y=w1038:dbl)
            n495 = Add(x=w1040, y=w1014) -> (x+y=w1037:dbl)
            n496 = call <vilib>:"WPI_RobotDriveRefNum Registry Get.vi"("refnum name"="RobotDrive") -> ("RobotDriveDevRef"=w1042:T13)  [unwired: 9 in, 1 out]
            n497 = Less?(x=w1017, y=0.5) -> (x < y?=w1015:bool)
            n498 = Greater?(x=w1027, y=200) -> (0:w1025:bool)
            n499 = call <vilib>:"WPI_SolenoidRefNum Registry Get.vi"("refnum name"="GearGate") -> ("error out"=w1034:errorcluster, "SolenoidDevRef"=w1033:T5)  [unwired: 9 in]
            n500 = call <vilib>:"WPI_RobotDriveTankDrive.vi"("Right axis value"=w1037, "Left axis value"=w1038, "RobotDriveDevRef"=w1042) -> ()  [unwired: 6 in, 3 out]
            n501 = call-poly <vilib>:"WPI_SolenoidSet.vi"("error in (no error)"=w1034, "Value"=WPI_SolenoidValue."On", "SolenoidDevRef"=w1033) -> ()  [unwired: 7 in, 2 out]
            n502 = Or(x=w1015, y=w1025) -> (x .or. y?=w1024:bool)
            n503 = Build Array(w1038, w1037, w1020) -> (w1035:dbl[])
            n504 = Array To Cluster(array=w1035) -> (cluster=→"DriveStraight 5":T1)
            n505 = call <vilib>:"WPI_SolenoidRefNum Registry Get.vi"("refnum name"="Banana") -> ("SolenoidDevRef"=w1030:T5)  [unwired: 9 in, 1 out]
            n506 = call-poly <vilib>:"WPI_SolenoidSet.vi"("Value"=WPI_SolenoidValue."On", "SolenoidDevRef"=w1030) -> ()  [unwired: 8 in, 2 out]
            n507 = Wait (ms)(milliseconds to wait=10) -> ()  [unwired: 1 out]
          }
        }
        frame #9 {
          n508 = call <vilib>:"WPI_EncoderRefNum Registry Get.vi"("refnum name"="Encoder 1") -> ("error out"=w1055:errorcluster, "EncoderDevRef"=w1057:T7)  [unwired: 9 in]
          n509 = call <vilib>:"WPI_EncoderRefNum Registry Get.vi"("refnum name"="Encoder 0") -> ("error out"=w1056:errorcluster, "EncoderDevRef"=w1058:T7)  [unwired: 9 in]
          n510 = call <vilib>:"WPI_SolenoidRefNum Registry Get.vi"("refnum name"="GearGate") -> ("error out"=w1054:errorcluster, "SolenoidDevRef"=w1053:T5)  [unwired: 9 in]
          n511 = call-poly <vilib>:"NT Read Value.vi"("Default Value"=14.0, "Name"="Circumference") -> ("Numeric"=w1044:dbl)  [unwired: 8 in, 1 out]
          n512 = call-poly <vilib>:"WPI_SolenoidSet.vi"("error in (no error)"=w1054, "Value"=WPI_SolenoidValue."On", "SolenoidDevRef"=w1053) -> ()  [unwired: 7 in, 2 out]
          n513 = call <vilib>:"WPI_EncoderReset.vi"("error in (no error)"=w1056, "EncoderDevRef"=w1058) -> ("error out"=w1049:errorcluster, "EncoderDevRef"=w1050:T7)  [unwired: 8 in]
          n514 = call <vilib>:"WPI_EncoderReset.vi"("error in (no error)"=w1055, "EncoderDevRef"=w1057) -> ("error out"=w1047:errorcluster, "EncoderDevRef"=w1048:T7)  [unwired: 8 in]
          n515 = while {
            tunnel: w1050 -> [w1080]
            tunnel: w1049 -> [w1079]
            tunnel: w1048 -> [w1078]
            tunnel: w1047 -> [w1077]
            tunnel: w1044 -> [w1062]
            tunnel: w1043 -> [w1061]
            i -> [w1067]
            stop <- w1063 stop-if-true
            w1095 = 0.7
            n516 = call <vilib>:"WPI_EncoderGet.vi"("error in (no error)"=w1079, "EncoderDevRef"=w1080) -> ("Distance"=w1076:dbl)  [unwired: 4 in, 5 out]
            n517 = call <vilib>:"WPI_EncoderGet.vi"("error in (no error)"=w1077, "EncoderDevRef"=w1078) -> ("Distance"=w1075:dbl)  [unwired: 4 in, 5 out]
            n518 = Subtract(x=w1076, y=w1075) -> (x-y=w1089:dbl)
            n519 = Add(x=w1076, y=w1075) -> (x+y=w1074:dbl)
            n520 = call-poly <vilib>:"PID.vi"("output range"=cluster{"output high":dbl, "output low":dbl} {"output high"=0.5, "output low"=-0.5}, "PID gains"=w1061, "process variable"=w1089, "setpoint"=0.0) -> ("output"=w1096:dbl)  [unwired: 6 in, 1 out]
            n521 = Divide(x=w1074, y=2.0) -> (x/y=w1069:dbl)
            n522 = Subtract(x=w1095, y=w1096) -> (x-y=w1091:dbl)
            n523 = Add(x=w1095, y=w1096) -> (x+y=w1090:dbl)
            n524 = call <vilib>:"WPI_RobotDriveRefNum Registry Get.vi"("refnum name"="RobotDrive") -> ("RobotDriveDevRef"=w1098:T13)  [unwired: 9 in, 1 out]
            n525 = Greater?(x=w1067, y=400) -> (0:w1064:bool)
            n526 = Divide(x=48.0, y=w1062) -> (x/y=w1071:dbl)
            n527 = call <vilib>:"WPI_SolenoidRefNum Registry Get.vi"("refnum name"="GearGate") -> ("error out"=w1087:errorcluster, "SolenoidDevRef"=w1086:T5)  [unwired: 9 in]
            n528 = call <vilib>:"WPI_RobotDriveTankDrive.vi"("Right axis value"=w1090, "Left axis value"=w1091, "RobotDriveDevRef"=w1098) -> ()  [unwired: 6 in, 3 out]
            n529 = Multiply(x=w1071, y=1024.0) -> (x*y=w1068:dbl)
            n530 = Greater Or Equal?(x=w1069, y=w1068) -> (x >= y?=w1065:bool)
            n531 = call-poly <vilib>:"WPI_SolenoidSet.vi"("error in (no error)"=w1087, "Value"=WPI_SolenoidValue."On", "SolenoidDevRef"=w1086) -> ()  [unwired: 7 in, 2 out]
            n532 = Or(x=w1065, y=w1064) -> (x .or. y?=w1063:bool)
            n533 = Build Array(w1091, w1090, w1089) -> (w1088:dbl[])
            n534 = Array To Cluster(array=w1088) -> ()  [unwired: 1 out]
            n535 = call <vilib>:"WPI_SolenoidRefNum Registry Get.vi"("refnum name"="Banana") -> ("SolenoidDevRef"=w1083:T5)  [unwired: 9 in, 1 out]
            n536 = call-poly <vilib>:"WPI_SolenoidSet.vi"("Value"=WPI_SolenoidValue."On", "SolenoidDevRef"=w1083) -> ()  [unwired: 8 in, 2 out]
            n537 = Wait (ms)(milliseconds to wait=10) -> ()  [unwired: 1 out]
          }
        }
      }
    }
    frame "Hopper", Default {
      n538 = flat-sequence {
        tunnel: w1109 -> [_]
        tunnel: w1108 -> [_]
        tunnel: w1104 -> [_]
        tunnel: w1103 -> [_]
        tunnel: [w1127] -> w1099
        tunnel: [w1197] -> w1100
        tunnel: w1099 -> [w1197]
        tunnel: w1107 -> [_]
        tunnel: w1106 -> [_]
        tunnel: w1105 -> [_]
        tunnel: [w1208] -> w1101
        tunnel: w1100 -> [w1208]
        tunnel: [w1230] -> w1102
        tunnel: w1101 -> [w1230]
        tunnel: w1102 -> [w1242]
        frame #0 {
          n539 = call <vilib>:"WPI_MotorControlRefNum Registry Get.vi"("refnum name"="Shooter" ("Name")) -> ("error out"=w1117:errorcluster, "MotorControlDevRef"=w1118:T14)  [unwired: 9 in]
          n540 = call <vilib>:"WPI_SolenoidRefNum Registry Get.vi"("refnum name"="Banana") -> ("SolenoidDevRef"=w1122:T5)  [unwired: 9 in, 1 out]
          n541 = call-poly <vilib>:"WPI_SolenoidSet.vi"("Value"=WPI_SolenoidValue."On", "SolenoidDevRef"=w1122) -> ()  [unwired: 8 in, 2 out]
          n542 = call "TalonPID.vi"("P"=0.5, "Ref In"=w1118, "Error in"=w1117, "I"=0.001, "I Zone"=5000.0, "Output"=-20000.0) -> ()  [unwired: 8 in, 2 out]
          n543 = call <vilib>:"WPI_SolenoidRefNum Registry Get.vi"("refnum name"="GearGate") -> ("error out"=w1126:errorcluster, "SolenoidDevRef"=w1125:T5)  [unwired: 9 in]
          n544 = call-poly <vilib>:"WPI_SolenoidSet.vi"("error in (no error)"=w1126, "Value"=WPI_SolenoidValue."On", "SolenoidDevRef"=w1125) -> ()  [unwired: 7 in, 2 out]
          n545 = call "Z900_navX_RefNum_Get.vi"("refnum name"="navX") -> ("error out"=w1111:errorcluster, "navX Device"=w1112:T11)  [unwired: 9 in]
          n546 = call "Z900_navX_Set_ZeroYaw.vi"("error in (no error)"=w1111, "navX Device"=w1112) -> ()  [unwired: 8 in, 2 out]
        }
        frame #1 {
          n547 = call <vilib>:"WPI_EncoderRefNum Registry Get.vi"("refnum name"="Encoder 1") -> ("error out"=w1139:errorcluster, "EncoderDevRef"=w1141:T7)  [unwired: 9 in]
          n548 = call <vilib>:"WPI_EncoderRefNum Registry Get.vi"("refnum name"="Encoder 0") -> ("error out"=w1140:errorcluster, "EncoderDevRef"=w1142:T7)  [unwired: 9 in]
          n549 = call <vilib>:"WPI_SolenoidRefNum Registry Get.vi"("refnum name"="GearGate") -> ("error out"=w1138:errorcluster, "SolenoidDevRef"=w1137:T5)  [unwired: 9 in]
          n550 = call-poly <vilib>:"NT Read Value.vi"("Default Value"=14.0, "Name"="Circumference") -> ("Numeric"=w1128:dbl)  [unwired: 8 in, 1 out]
          n551 = call-poly <vilib>:"WPI_SolenoidSet.vi"("error in (no error)"=w1138, "Value"=WPI_SolenoidValue."On", "SolenoidDevRef"=w1137) -> ()  [unwired: 7 in, 2 out]
          n552 = call <vilib>:"WPI_EncoderReset.vi"("error in (no error)"=w1140, "EncoderDevRef"=w1142) -> ("error out"=w1133:errorcluster, "EncoderDevRef"=w1134:T7)  [unwired: 8 in]
          n553 = call <vilib>:"WPI_EncoderReset.vi"("error in (no error)"=w1139, "EncoderDevRef"=w1141) -> ("error out"=w1131:errorcluster, "EncoderDevRef"=w1132:T7)  [unwired: 8 in]
          n554 = while {
            tunnel: w1134 -> [w1175]
            tunnel: w1133 -> [w1174]
            tunnel: w1132 -> [w1173]
            tunnel: w1131 -> [w1172]
            tunnel: w1128 -> [w1157]
            tunnel: ["ForwardPID"] -> w1127
            i -> [w1162]
            stop <- w1158 stop-if-true
            w1156 = 0.65 ("x")
            n555 = call <vilib>:"WPI_EncoderGet.vi"("error in (no error)"=w1174, "EncoderDevRef"=w1175) -> ("Distance"=w1171:dbl)  [unwired: 4 in, 5 out]
            n556 = call <vilib>:"WPI_EncoderGet.vi"("error in (no error)"=w1172, "EncoderDevRef"=w1173) -> ("Distance"=w1170:dbl)  [unwired: 4 in, 5 out]
            n557 = Subtract(x=w1171, y=w1170) -> (x-y=w1185:dbl)
            n558 = call "Z900_navX_RefNum_Get.vi"("refnum name"="navX") -> ("error out"=w1146:errorcluster, "navX Device"=w1147:T11)  [unwired: 9 in]
            n559 = call "Z900_navX_Set_ZeroYaw.vi"("error in (no error)"=w1146, "navX Device"=w1147) -> ()  [unwired: 8 in, 2 out]
            n560 = Add(x=w1171, y=w1170) -> (x+y=w1169:dbl)
            n561 = call-poly <vilib>:"PID.vi"("output range"=cluster{"output high":dbl, "output low":dbl} {"output high"=0.5, "output low"=-0.5}, "PID gains"="ForwardPID", "process variable"=w1185, "setpoint"=0.0) -> ("output"=w1191:dbl)  [unwired: 6 in, 1 out]
            n562 = Divide(x=w1169, y=2.0) -> (x/y=w1164:dbl)
            n563 = Subtract(x=w1156, y=w1191) -> (x-y=w1187:dbl)
            n564 = Add(x=w1156, y=w1191) -> (x+y=w1186:dbl)
            n565 = call <vilib>:"WPI_RobotDriveRefNum Registry Get.vi"("refnum name"="RobotDrive") -> ("RobotDriveDevRef"=w1193:T13)  [unwired: 9 in, 1 out]
            n566 = Greater?(x=w1162, y=600) -> (0:w1159:bool)
            n567 = Divide(x=66.0, y=w1157) -> (x/y=w1166:dbl)
            n568 = call <vilib>:"WPI_SolenoidRefNum Registry Get.vi"("refnum name"="GearGate") -> ("error out"=w1182:errorcluster, "SolenoidDevRef"=w1181:T5)  [unwired: 9 in]
            n569 = call <vilib>:"WPI_RobotDriveTankDrive.vi"("Right axis value"=w1186, "Left axis value"=w1187, "RobotDriveDevRef"=w1193) -> ()  [unwired: 6 in, 3 out]
            n570 = Multiply(x=w1166, y=1024.0) -> (x*y=w1163:dbl)
            n571 = Greater Or Equal?(x=w1164, y=w1163) -> (x >= y?=w1160:bool)
            n572 = call-poly <vilib>:"WPI_SolenoidSet.vi"("error in (no error)"=w1182, "Value"=WPI_SolenoidValue."On", "SolenoidDevRef"=w1181) -> ()  [unwired: 7 in, 2 out]
            n573 = Or(x=w1160, y=w1159) -> (x .or. y?=w1158:bool)
            n574 = Build Array(w1187, w1186, w1185) -> (w1183:dbl[])
            n575 = Array To Cluster(array=w1183) -> (cluster=→"DriveStraight":T1)
            n576 = call <vilib>:"WPI_MotorControlRefNum Registry Get.vi"("refnum name"="Shooter" ("Name")) -> ("error out"=w1152:errorcluster, "MotorControlDevRef"=w1153:T14)  [unwired: 9 in]
            n577 = call <vilib>:"WPI_SolenoidRefNum Registry Get.vi"("refnum name"="Banana") -> ("SolenoidDevRef"=w1178:T5)  [unwired: 9 in, 1 out]
            n578 = call-poly <vilib>:"WPI_SolenoidSet.vi"("Value"=WPI_SolenoidValue."On", "SolenoidDevRef"=w1178) -> ()  [unwired: 8 in, 2 out]
            n579 = call "TalonPID.vi"("P"=0.3, "Ref In"=w1153, "Error in"=w1152, "I"=0.001, "I Zone"=5000.0, "Output"=-20000.0) -> ()  [unwired: 8 in, 2 out]
            n580 = Wait (ms)(milliseconds to wait=10) -> ()  [unwired: 1 out]
          }
        }
        frame #2 {
          w1204 = 0.0 ("Right axis value")
          n581 = Wait (ms)(milliseconds to wait=500) -> ()  [unwired: 1 out]
          n582 = call <vilib>:"WPI_RobotDriveRefNum Registry Get.vi"("refnum name"="RobotDrive") -> ("RobotDriveDevRef"=w1205:T13)  [unwired: 9 in, 1 out]
          n583 = call <vilib>:"WPI_SolenoidRefNum Registry Get.vi"("refnum name"="GearGate") -> ("error out"=w1202:errorcluster, "SolenoidDevRef"=w1201:T5)  [unwired: 9 in]
          n584 = call "Z900_navX_RefNum_Get.vi"("refnum name"="navX") -> ("error out"=w1195:errorcluster, "navX Device"=w1196:T11)  [unwired: 9 in]
          n585 = call <vilib>:"WPI_RobotDriveTankDrive.vi"("Right axis value"=w1204, "Left axis value"=w1204, "RobotDriveDevRef"=w1205) -> ()  [unwired: 6 in, 3 out]
          n586 = call "Z900_navX_Set_ZeroYaw.vi"("error in (no error)"=w1195, "navX Device"=w1196) -> ()  [unwired: 8 in, 2 out]
          n587 = call-poly <vilib>:"WPI_SolenoidSet.vi"("error in (no error)"=w1202, "Value"=WPI_SolenoidValue."On", "SolenoidDevRef"=w1201) -> ()  [unwired: 7 in, 2 out]
        }
        frame #3 {
          n588 = call "Z900_navX_RefNum_Get.vi"("refnum name"="navX") -> ("error out"=w1210:errorcluster, "navX Device"=w1211:T11)  [unwired: 9 in]
          n589 = call "Z900_navX_Set_ZeroYaw.vi"("error in (no error)"=w1210, "navX Device"=w1211) -> ("error out"=w1206:errorcluster, "navX Device"=w1207:T11)  [unwired: 8 in]
          n590 = while {
            tunnel: w1207 -> [w1213]
            tunnel: w1206 -> [w1212]
            stop <- w1214 stop-if-true
            w1224 = -0.55 ("Right axis value")
            n591 = call "Z900_navX_Get_YPRHfH.vi"("error in (no error)"=w1212, "navX Device"=w1213) -> ("YRPHfH"=w1216:T18)  [unwired: 6 in, 3 out]
            n592 = Unbundle By Name(w1216) -> ("Yaw"=w1215:dbl)
            n593 = call <vilib>:"WPI_MotorControlRefNum Registry Get.vi"("refnum name"="Shooter" ("Name")) -> ("error out"=w1221:errorcluster, "MotorControlDevRef"=w1222:T14)  [unwired: 9 in]
            n594 = call <vilib>:"WPI_RobotDriveRefNum Registry Get.vi"("refnum name"="RobotDrive") -> ("RobotDriveDevRef"=w1228:T13)  [unwired: 9 in, 1 out]
            n595 = Multiply(x=-1.0, y=w1224) -> (x*y=w1225:dbl)
            n596 = call <vilib>:"WPI_RobotDriveTankDrive.vi"("Right axis value"=w1225, "Left axis value"=w1224, "RobotDriveDevRef"=w1228) -> ()  [unwired: 6 in, 3 out]
            n597 = call "TalonPID.vi"("P"=0.5, "Ref In"=w1222, "Error in"=w1221, "I"=0.001, "I Zone"=5000.0, "Output"=-20000.0) -> ()  [unwired: 8 in, 2 out]
            n598 = Greater?(x=w1215, y=85.0) -> (0:w1214:bool)
          }
        }
        frame #4 {
          w1236 = 0.0 ("Left axis value")
          n599 = call <vilib>:"WPI_RobotDriveRefNum Registry Get.vi"("refnum name"="RobotDrive") -> ("error out"=w1237:errorcluster, "RobotDriveDevRef"=w1238:T13)  [unwired: 9 in]
          n600 = call <vilib>:"WPI_SolenoidRefNum Registry Get.vi"("refnum name"="GearGate") -> ("error out"=w1234:errorcluster, "SolenoidDevRef"=w1233:T5)  [unwired: 9 in]
          n601 = call <vilib>:"WPI_RobotDriveTankDrive.vi"("error in (no error)"=w1237, "Right axis value"=w1236, "Left axis value"=w1236, "RobotDriveDevRef"=w1238) -> ()  [unwired: 5 in, 3 out]
          n602 = call-poly <vilib>:"WPI_SolenoidSet.vi"("error in (no error)"=w1234, "Value"=WPI_SolenoidValue."On", "SolenoidDevRef"=w1233) -> ()  [unwired: 7 in, 2 out]
        }
        frame #5 {
          n603 = call <vilib>:"WPI_EncoderRefNum Registry Get.vi"("refnum name"="Encoder 1") -> ("error out"=w1251:errorcluster, "EncoderDevRef"=w1253:T7)  [unwired: 9 in]
          n604 = call <vilib>:"WPI_EncoderRefNum Registry Get.vi"("refnum name"="Encoder 0") -> ("error out"=w1252:errorcluster, "EncoderDevRef"=w1254:T7)  [unwired: 9 in]
          n605 = call <vilib>:"WPI_SolenoidRefNum Registry Get.vi"("refnum name"="GearGate") -> ("error out"=w1250:errorcluster, "SolenoidDevRef"=w1249:T5)  [unwired: 9 in]
          n606 = call-poly <vilib>:"WPI_SolenoidSet.vi"("error in (no error)"=w1250, "Value"=WPI_SolenoidValue."On", "SolenoidDevRef"=w1249) -> ()  [unwired: 7 in, 2 out]
          n607 = call "Z900_navX_RefNum_Get.vi"("refnum name"="navX") -> ("error out"=w1240:errorcluster, "navX Device"=w1241:T11)  [unwired: 9 in]
          n608 = call <vilib>:"WPI_EncoderReset.vi"("error in (no error)"=w1252, "EncoderDevRef"=w1254) -> ("error out"=w1245:errorcluster, "EncoderDevRef"=w1246:T7)  [unwired: 8 in]
          n609 = call <vilib>:"WPI_EncoderReset.vi"("error in (no error)"=w1251, "EncoderDevRef"=w1253) -> ("error out"=w1243:errorcluster, "EncoderDevRef"=w1244:T7)  [unwired: 8 in]
          n610 = call "Z900_navX_Set_ZeroYaw.vi"("error in (no error)"=w1240, "navX Device"=w1241) -> ()  [unwired: 8 in, 2 out]
          n611 = while {
            tunnel: w1246 -> [w1274]
            tunnel: w1245 -> [w1273]
            tunnel: w1244 -> [w1272]
            tunnel: w1243 -> [w1271]
            tunnel: w1242 -> [w1265]
            i -> [w1268]
            stop <- w1257 stop-if-true
            w1266 = -0.65 ("x")
            n612 = call <vilib>:"WPI_EncoderGet.vi"("error in (no error)"=w1273, "EncoderDevRef"=w1274) -> ("Distance"=w1270:dbl)  [unwired: 4 in, 5 out]
            n613 = call <vilib>:"WPI_EncoderGet.vi"("error in (no error)"=w1271, "EncoderDevRef"=w1272) -> ("Distance"=w1269:dbl)  [unwired: 4 in, 5 out]
            n614 = Subtract(x=w1270, y=w1269) -> (x-y=w1284:dbl)
            n615 = call-poly <vilib>:"PID.vi"("output range"=cluster{"output high":dbl, "output low":dbl} {"output high"=0.5, "output low"=-0.5}, "PID gains"=w1265, "process variable"=w1284, "setpoint"=0.0) -> ("output"=w1290:dbl)  [unwired: 6 in, 1 out]
            n616 = Subtract(x=w1266, y=w1290) -> (x-y=w1286:dbl)
            n617 = Add(x=w1266, y=w1290) -> (x+y=w1285:dbl)
            n618 = call <vilib>:"WPI_RobotDriveRefNum Registry Get.vi"("refnum name"="RobotDrive") -> ("RobotDriveDevRef"=w1292:T13)  [unwired: 9 in, 1 out]
            n619 = Greater?(x=w1268, y=100) -> (0:w1257:bool)
            n620 = call <vilib>:"WPI_SolenoidRefNum Registry Get.vi"("refnum name"="GearGate") -> ("error out"=w1281:errorcluster, "SolenoidDevRef"=w1280:T5)  [unwired: 9 in]
            n621 = call <vilib>:"WPI_RobotDriveTankDrive.vi"("Right axis value"=w1285, "Left axis value"=w1286, "RobotDriveDevRef"=w1292) -> ()  [unwired: 6 in, 3 out]
            n622 = call-poly <vilib>:"WPI_SolenoidSet.vi"("error in (no error)"=w1281, "Value"=WPI_SolenoidValue."On", "SolenoidDevRef"=w1280) -> ()  [unwired: 7 in, 2 out]
            n623 = Build Array(w1286, w1285, w1284) -> (w1282:dbl[])
            n624 = Array To Cluster(array=w1282) -> (cluster=→"DriveStraight 3":T1)
            n625 = call <vilib>:"WPI_MotorControlRefNum Registry Get.vi"("refnum name"="Shooter" ("Name")) -> ("error out"=w1262:errorcluster, "MotorControlDevRef"=w1263:T14)  [unwired: 9 in]
            n626 = call <vilib>:"WPI_SolenoidRefNum Registry Get.vi"("refnum name"="Banana") -> ("SolenoidDevRef"=w1277:T5)  [unwired: 9 in, 1 out]
            n627 = call-poly <vilib>:"WPI_SolenoidSet.vi"("Value"=WPI_SolenoidValue."On", "SolenoidDevRef"=w1277) -> ()  [unwired: 8 in, 2 out]
            n628 = call "TalonPID.vi"("P"=0.3, "Ref In"=w1263, "Error in"=w1262, "I"=0.001, "I Zone"=5000.0, "Output"=-20000.0) -> ()  [unwired: 8 in, 2 out]
            n629 = Wait (ms)(milliseconds to wait=10) -> ()  [unwired: 1 out]
          }
        }
        frame #6 {
          (unwired) 0.0 ("Right axis value")
          n630 = call <vilib>:"WPI_MotorControlRefNum Registry Get.vi"("refnum name"="Shooter" ("Name")) -> ("error out"=w1297:errorcluster, "MotorControlDevRef"=w1298:T14)  [unwired: 9 in]
          n631 = call "TalonPID.vi"("P"=0.3, "Ref In"=w1298, "Error in"=w1297, "I"=0.001, "I Zone"=5000.0, "Output"=-20000.0) -> ()  [unwired: 8 in, 2 out]
          n632 = Multiply(x=0.9, y=-1.0) -> (x*y=w1311:dbl)
          n633 = call <vilib>:"WPI_RobotDriveRefNum Registry Get.vi"("refnum name"="RobotDrive") -> ("error out"=w1301:errorcluster, "RobotDriveDevRef"=w1300:T13)  [unwired: 9 in]
          n634 = call <vilib>:"WPI_MotorControlRefNum Registry Get.vi"("refnum name"="Feeder") -> ("error out"=w1309:errorcluster, "MotorControlDevRef"=w1308:T14)  [unwired: 9 in]
          n635 = call <vilib>:"WPI_MotorControlRefNum Registry Get.vi"("refnum name"="Shuriken") -> ("error out"=w1307:errorcluster, "MotorControlDevRef"=w1306:T14)  [unwired: 9 in]
          n636 = call <vilib>:"WPI_RobotDriveTankDrive.vi"("error in (no error)"=w1301, "Left axis value"=0.0, "RobotDriveDevRef"=w1300) -> ()  [unwired: 6 in, 3 out]
          n637 = call <vilib>:"WPI_MotorControlSetOutput.vi"("error in (no error)"=w1309, "Output"=w1311, "MotorControlDevRef"=w1308) -> ()  [unwired: 6 in, 3 out]
          n638 = call <vilib>:"WPI_MotorControlSetOutput.vi"("error in (no error)"=w1307, "Output"=0.4, "MotorControlDevRef"=w1306) -> ()  [unwired: 6 in, 3 out]
          n639 = Wait (ms)(milliseconds to wait=1000) -> ()  [unwired: 1 out]
        }
        frame #7 {
          n640 = call <vilib>:"WPI_MotorControlRefNum Registry Get.vi"("refnum name"="Shooter") -> ("MotorControlDevRef"=w1333:T14)  [unwired: 9 in, 1 out]
          n641 = call <vilib>:"WPI_RobotDriveRefNum Registry Get.vi"("refnum name"="RobotDrive") -> ("error out"=w1316:errorcluster, "RobotDriveDevRef"=w1315:T13)  [unwired: 9 in]
          n642 = Multiply(x=0.0, y=-1.0) -> (x*y=w1322:dbl)
          n643 = call <vilib>:"WPI_RobotDriveTankDrive.vi"("error in (no error)"=w1316, "Right axis value"=0.0, "Left axis value"=0.0, "RobotDriveDevRef"=w1315) -> ()  [unwired: 5 in, 3 out]
          n644 = call <vilib>:"WPI_CANTalonSRX_ChangeMode.vi"("Control Mode"=WPI_CANTalonSRX_APIControlMode."Percent VBus", "CAN Talon SRX Ref"=w1333) -> ("CAN Talon SRX Ref"=w1332:T14)  [unwired: 8 in, 1 out]
          n645 = call <vilib>:"WPI_MotorControlSetOutput.vi"("Output"=0.0, "MotorControlDevRef"=w1332) -> ()  [unwired: 7 in, 3 out]
          n646 = call <vilib>:"WPI_MotorControlRefNum Registry Get.vi"("refnum name"="Feeder") -> ("error out"=w1324:errorcluster, "MotorControlDevRef"=w1325:T14)  [unwired: 9 in]
          n647 = call <vilib>:"WPI_MotorControlRefNum Registry Get.vi"("refnum name"="Shuriken") -> ("error out"=w1326:errorcluster, "MotorControlDevRef"=w1327:T14)  [unwired: 9 in]
          n648 = call <vilib>:"WPI_MotorControlSetOutput.vi"("error in (no error)"=w1324, "Output"=w1322, "MotorControlDevRef"=w1325) -> ()  [unwired: 6 in, 3 out]
          n649 = call <vilib>:"WPI_MotorControlSetOutput.vi"("error in (no error)"=w1326, "Output"=0.0, "MotorControlDevRef"=w1327) -> ()  [unwired: 6 in, 3 out]
        }
      }
    }
    frame "frontGear" {
      n650 = flat-sequence {
        tunnel: w1341 -> [_]
        tunnel: w1340 -> [_]
        tunnel: w1336 -> [_]
        tunnel: w1335 -> [_]
        tunnel: w1339 -> [w1426]
        tunnel: w1338 -> [w1425]
        tunnel: w1337 -> [w1424]
        frame #0 {
          n651 = call <vilib>:"WPI_SolenoidRefNum Registry Get.vi"("refnum name"="Banana") -> ("SolenoidDevRef"=w1349:T5)  [unwired: 9 in, 1 out]
          n652 = call-poly <vilib>:"WPI_SolenoidSet.vi"("Value"=WPI_SolenoidValue."On", "SolenoidDevRef"=w1349) -> ()  [unwired: 8 in, 2 out]
          n653 = call <vilib>:"WPI_MotorControlRefNum Registry Get.vi"("refnum name"="Shooter") -> ("MotorControlDevRef"=w1345:T14)  [unwired: 9 in, 1 out]
          n654 = call <vilib>:"WPI_SolenoidRefNum Registry Get.vi"("refnum name"="GearGate") -> ("error out"=w1353:errorcluster, "SolenoidDevRef"=w1352:T5)  [unwired: 9 in]
          n655 = call-poly <vilib>:"WPI_SolenoidSet.vi"("error in (no error)"=w1353, "Value"=WPI_SolenoidValue."On", "SolenoidDevRef"=w1352) -> ()  [unwired: 7 in, 2 out]
          n656 = call <vilib>:"WPI_CANTalonSRX_ChangeMode.vi"("Control Mode"=WPI_CANTalonSRX_APIControlMode."Percent VBus", "CAN Talon SRX Ref"=w1345) -> ("CAN Talon SRX Ref"=w1344:T14)  [unwired: 8 in, 1 out]
          n657 = call <vilib>:"WPI_MotorControlSetOutput.vi"("Output"=-0.4, "MotorControlDevRef"=w1344) -> ()  [unwired: 7 in, 3 out]
        }
        frame #1 {
          n658 = call <vilib>:"WPI_EncoderRefNum Registry Get.vi"("refnum name"="Encoder 1") -> ("error out"=w1365:errorcluster, "EncoderDevRef"=w1367:T7)  [unwired: 9 in]
          n659 = call <vilib>:"WPI_EncoderRefNum Registry Get.vi"("refnum name"="Encoder 0") -> ("error out"=w1366:errorcluster, "EncoderDevRef"=w1368:T7)  [unwired: 9 in]
          n660 = call <vilib>:"WPI_SolenoidRefNum Registry Get.vi"("refnum name"="GearGate") -> ("error out"=w1364:errorcluster, "SolenoidDevRef"=w1363:T5)  [unwired: 9 in]
          n661 = call-poly <vilib>:"NT Read Value.vi"("Default Value"=14.0, "Name"="Circumference") -> ("Numeric"=w1354:dbl)  [unwired: 8 in, 1 out]
          n662 = call-poly <vilib>:"WPI_SolenoidSet.vi"("error in (no error)"=w1364, "Value"=WPI_SolenoidValue."On", "SolenoidDevRef"=w1363) -> ()  [unwired: 7 in, 2 out]
          n663 = call <vilib>:"WPI_EncoderReset.vi"("error in (no error)"=w1366, "EncoderDevRef"=w1368) -> ("error out"=w1359:errorcluster, "EncoderDevRef"=w1360:T7)  [unwired: 8 in]
          n664 = call <vilib>:"WPI_EncoderReset.vi"("error in (no error)"=w1365, "EncoderDevRef"=w1367) -> ("error out"=w1357:errorcluster, "EncoderDevRef"=w1358:T7)  [unwired: 8 in]
          n665 = while {
            tunnel: w1360 -> [w1395]
            tunnel: w1359 -> [w1394]
            tunnel: w1358 -> [w1393]
            tunnel: w1357 -> [w1392]
            tunnel: w1354 -> [w1377]
            i -> [w1382]
            stop <- w1378 stop-if-true
            w1371 = 0.5 ("x")
            n666 = call <vilib>:"WPI_EncoderGet.vi"("error in (no error)"=w1394, "EncoderDevRef"=w1395) -> ("Distance"=w1391:dbl)  [unwired: 4 in, 5 out]
            n667 = call <vilib>:"WPI_EncoderGet.vi"("error in (no error)"=w1392, "EncoderDevRef"=w1393) -> ("Distance"=w1390:dbl)  [unwired: 4 in, 5 out]
            n668 = Subtract(x=w1391, y=w1390) -> (x-y=w1405:dbl)
            n669 = Add(x=w1391, y=w1390) -> (x+y=w1389:dbl)
            n670 = call-poly <vilib>:"PID.vi"("output range"=cluster{"output high":dbl, "output low":dbl} {"output high"=0.5, "output low"=-0.5}, "PID gains"="ForwardPID 2", "process variable"=w1405, "setpoint"=0.0) -> ("output"=w1412:dbl)  [unwired: 6 in, 1 out]
            n671 = Divide(x=w1389, y=2.0) -> (x/y=w1384:dbl)
            n672 = Subtract(x=w1371, y=w1412) -> (x-y=w1407:dbl)
            n673 = Add(x=w1371, y=w1412) -> (x+y=w1406:dbl)
            n674 = call <vilib>:"WPI_RobotDriveRefNum Registry Get.vi"("refnum name"="RobotDrive") -> ("RobotDriveDevRef"=w1414:T13)  [unwired: 9 in, 1 out]
            n675 = Greater?(x=w1382, y=600) -> (0:w1379:bool)
            n676 = Divide(x=78.297, y=w1377) -> (x/y=w1386:dbl)
            n677 = call <vilib>:"WPI_SolenoidRefNum Registry Get.vi"("refnum name"="GearGate") -> ("error out"=w1402:errorcluster, "SolenoidDevRef"=w1401:T5)  [unwired: 9 in]
            n678 = call <vilib>:"WPI_RobotDriveTankDrive.vi"("Right axis value"=w1406, "Left axis value"=w1407, "RobotDriveDevRef"=w1414) -> ()  [unwired: 6 in, 3 out]
            n679 = Multiply(x=w1386, y=1024.0) -> (x*y=w1383:dbl)
            n680 = Greater Or Equal?(x=w1384, y=w1383) -> (x >= y?=w1380:bool)
            n681 = call-poly <vilib>:"WPI_SolenoidSet.vi"("error in (no error)"=w1402, "Value"=WPI_SolenoidValue."On", "SolenoidDevRef"=w1401) -> ()  [unwired: 7 in, 2 out]
            n682 = Or(x=w1380, y=w1379) -> (x .or. y?=w1378:bool)
            n683 = Build Array(w1407, w1406, w1405) -> (w1403:dbl[])
            n684 = Array To Cluster(array=w1403) -> (cluster=→"DriveStraight 2":T1)
            n685 = call <vilib>:"WPI_SolenoidRefNum Registry Get.vi"("refnum name"="Banana") -> ("SolenoidDevRef"=w1398:T5)  [unwired: 9 in, 1 out]
            n686 = call <vilib>:"WPI_MotorControlRefNum Registry Get.vi"("refnum name"="Shooter") -> ("MotorControlDevRef"=w1375:T14)  [unwired: 9 in, 1 out]
            n687 = call-poly <vilib>:"WPI_SolenoidSet.vi"("Value"=WPI_SolenoidValue."On", "SolenoidDevRef"=w1398) -> ()  [unwired: 8 in, 2 out]
            n688 = call <vilib>:"WPI_CANTalonSRX_ChangeMode.vi"("Control Mode"=WPI_CANTalonSRX_APIControlMode."Percent VBus", "CAN Talon SRX Ref"=w1375) -> ("CAN Talon SRX Ref"=w1374:T14)  [unwired: 8 in, 1 out]
            n689 = call <vilib>:"WPI_MotorControlSetOutput.vi"("Output"=-0.4, "MotorControlDevRef"=w1374) -> ()  [unwired: 7 in, 3 out]
            n690 = Wait (ms)(milliseconds to wait=10) -> ()  [unwired: 1 out]
          }
        }
        frame #2 {
          w1421 = 0.0 ("Right axis value")
          n691 = call <vilib>:"WPI_RobotDriveRefNum Registry Get.vi"("refnum name"="RobotDrive") -> ("RobotDriveDevRef"=w1422:T13)  [unwired: 9 in, 1 out]
          n692 = call <vilib>:"WPI_SolenoidRefNum Registry Get.vi"("refnum name"="GearGate") -> ("error out"=w1419:errorcluster, "SolenoidDevRef"=w1418:T5)  [unwired: 9 in]
          n693 = call <vilib>:"WPI_RobotDriveTankDrive.vi"("Right axis value"=w1421, "Left axis value"=w1421, "RobotDriveDevRef"=w1422) -> ()  [unwired: 6 in, 3 out]
          n694 = call-poly <vilib>:"WPI_SolenoidSet.vi"("error in (no error)"=w1419, "Value"=WPI_SolenoidValue."On", "SolenoidDevRef"=w1418) -> ()  [unwired: 7 in, 2 out]
          n695 = Wait (ms)(milliseconds to wait=500) -> ()  [unwired: 1 out]
        }
        frame #3 {
          n696 = for {
            N: 0 -> [_]
            tunnel: w1426 -> [w1432]
            tunnel: w1425 -> [w1431]
            tunnel: w1424 -> [w1430]
            n697 = global read "Robot Global Data.vi" "TargetsFound"() -> (w1433:bool)
            n698 = case shown="True" w1433 {
              tunnel: [w1441 w1457] -> w1436
              tunnel: [w1441 w1456] -> w1437
              tunnel: TRUE -> [_ w1452]
              tunnel: w1432 -> [_ w1451]
              tunnel: w1431 -> [_ w1450]
              tunnel: w1430 -> [_ w1449]
              frame False {
                w1441 = 0.0
              }
              frame True {
                n699 = call <vilib>:"WPI_SolenoidRefNum Registry Get.vi"("refnum name"="Banana") -> ("SolenoidDevRef"=w1444:T5)  [unwired: 9 in, 1 out]
                n700 = global read "Robot Global Data.vi" "Mid"() -> (w1460:dbl)
                n701 = Subtract(x=w1460, y=w1450) -> (x-y=w1454:dbl)
                n702 = Absolute Value(x=w1454) -> (abs(x)=w1459:dbl)
                n703 = Less?(x=w1459, y=w1449) -> (x < y?=w1458:bool)
                n704 = Greater?(x=w1454, y=0.0) -> (0:w1455:bool)
                n705 = call-poly <vilib>:"WPI_SolenoidSet.vi"("Value"=WPI_SolenoidValue."On", "SolenoidDevRef"=w1444) -> ()  [unwired: 8 in, 2 out]
                n706 = case shown="False" w1455 {
                  tunnel: w1458 -> [w1461 w1476]
                  tunnel: [w1462 w1474] -> w1457
                  tunnel: [w1463 w1475] -> w1456
                  tunnel: w1452 -> [_ _]
                  tunnel: w1451 -> [w1464 w1473]
                  frame False {
                    n707 = case shown="True" w1461 {
                      tunnel: [w1469 w1472] -> w1463
                      tunnel: [w1467 w1472] -> w1462
                      tunnel: w1464 -> [w1465 w1470]
                      frame False {
                        n708 = Multiply(x=w1465, y=1.0) -> (x*y=w1469:dbl)
                        n709 = Multiply(x=w1465, y=-1.2) -> (x*y=w1467:dbl)
                      }
                      frame True {
                        n710 = Multiply(x=w1470, y=1.2) -> (x*y=w1472:dbl)
                      }
                    }
                  }
                  frame True {
                    n711 = case shown="True" w1476 {
                      tunnel: [w1481 w1484] -> w1475
                      tunnel: [w1479 w1484] -> w1474
                      tunnel: w1473 -> [w1477 w1482]
                      frame False {
                        n712 = Multiply(x=w1477, y=1.0) -> (x*y=w1479:dbl)
                        n713 = Multiply(x=w1477, y=-1.0) -> (x*y=w1481:dbl)
                      }
                      frame True {
                        n714 = Multiply(x=w1482, y=1.2) -> (x*y=w1484:dbl)
                      }
                    }
                  }
                }
                n715 = call <vilib>:"WPI_SolenoidRefNum Registry Get.vi"("refnum name"="GearGate") -> ("error out"=w1448:errorcluster, "SolenoidDevRef"=w1447:T5)  [unwired: 9 in]
                n716 = call-poly <vilib>:"WPI_SolenoidSet.vi"("error in (no error)"=w1448, "Value"=WPI_SolenoidValue."On", "SolenoidDevRef"=w1447) -> ()  [unwired: 7 in, 2 out]
              }
            }
            n717 = call <vilib>:"WPI_SolenoidRefNum Registry Get.vi"("refnum name"="Banana") -> ("SolenoidDevRef"=w1429:T5)  [unwired: 9 in, 1 out]
            n718 = call-poly <vilib>:"WPI_SolenoidSet.vi"("Value"=WPI_SolenoidValue."On", "SolenoidDevRef"=w1429) -> ()  [unwired: 8 in, 2 out]
            n719 = call <vilib>:"WPI_RobotDriveRefNum Registry Get.vi"("refnum name"="RobotDrive") -> ("error out"=w1438:errorcluster, "RobotDriveDevRef"=w1439:T13)  [unwired: 9 in]
            n720 = Wait (ms)(milliseconds to wait=10) -> ()  [unwired: 1 out]
            n721 = call <vilib>:"WPI_RobotDriveTankDrive.vi"("error in (no error)"=w1438, "Right axis value"=w1436, "Left axis value"=w1437, "RobotDriveDevRef"=w1439) -> ()  [unwired: 5 in, 3 out]
          }
        }
        frame #4 {
          w1490 = 0.0 ("Left axis value")
          n722 = call <vilib>:"WPI_RobotDriveRefNum Registry Get.vi"("refnum name"="RobotDrive") -> ("error out"=w1491:errorcluster, "RobotDriveDevRef"=w1492:T13)  [unwired: 9 in]
          n723 = call <vilib>:"WPI_SolenoidRefNum Registry Get.vi"("refnum name"="GearGate") -> ("error out"=w1488:errorcluster, "SolenoidDevRef"=w1487:T5)  [unwired: 9 in]
          n724 = call <vilib>:"WPI_RobotDriveTankDrive.vi"("error in (no error)"=w1491, "Right axis value"=w1490, "Left axis value"=w1490, "RobotDriveDevRef"=w1492) -> ()  [unwired: 5 in, 3 out]
          n725 = call-poly <vilib>:"WPI_SolenoidSet.vi"("error in (no error)"=w1488, "Value"=WPI_SolenoidValue."On", "SolenoidDevRef"=w1487) -> ()  [unwired: 7 in, 2 out]
        }
        frame #5 {
          n726 = for {
            N: 3 -> [_]
            n727 = flat-sequence {
              frame #0 {
                n728 = call <vilib>:"WPI_SolenoidRefNum Registry Get.vi"("refnum name"="Gears") -> ("error out"=w1510:errorcluster, "SolenoidDevRef"=w1509:T5)  [unwired: 9 in]
                n729 = call <vilib>:"WPI_SolenoidRefNum Registry Get.vi"("refnum name"="GearGate") -> ("error out"=w1505:errorcluster, "SolenoidDevRef"=w1504:T5)  [unwired: 9 in]
                n730 = call-poly <vilib>:"WPI_SolenoidSet.vi"("error in (no error)"=w1510, "Value"=WPI_SolenoidValue."On", "SolenoidDevRef"=w1509) -> ()  [unwired: 7 in, 2 out]
                n731 = Wait (ms)(milliseconds to wait=166) -> ()  [unwired: 1 out]
                n732 = call-poly <vilib>:"WPI_SolenoidSet.vi"("error in (no error)"=w1505, "Value"=WPI_SolenoidValue."On", "SolenoidDevRef"=w1504) -> ()  [unwired: 7 in, 2 out]
              }
              frame #1 {
                n733 = call <vilib>:"WPI_SolenoidRefNum Registry Get.vi"("refnum name"="Gears") -> ("error out"=w1519:errorcluster, "SolenoidDevRef"=w1518:T5)  [unwired: 9 in]
                n734 = call <vilib>:"WPI_SolenoidRefNum Registry Get.vi"("refnum name"="GearGate") -> ("error out"=w1514:errorcluster, "SolenoidDevRef"=w1513:T5)  [unwired: 9 in]
                n735 = Wait (ms)(milliseconds to wait=166) -> ()  [unwired: 1 out]
                n736 = call-poly <vilib>:"WPI_SolenoidSet.vi"("error in (no error)"=w1519, "Value"=WPI_SolenoidValue."Off", "SolenoidDevRef"=w1518) -> ()  [unwired: 7 in, 2 out]
                n737 = call-poly <vilib>:"WPI_SolenoidSet.vi"("error in (no error)"=w1514, "Value"=WPI_SolenoidValue."On", "SolenoidDevRef"=w1513) -> ()  [unwired: 7 in, 2 out]
              }
            }
          }
          n738 = call <vilib>:"WPI_SolenoidRefNum Registry Get.vi"("refnum name"="Banana") -> ("SolenoidDevRef"=w1500:T5)  [unwired: 9 in, 1 out]
          n739 = call <vilib>:"WPI_MotorControlRefNum Registry Get.vi"("refnum name"="Shooter") -> ("MotorControlDevRef"=w1496:T14)  [unwired: 9 in, 1 out]
          n740 = call-poly <vilib>:"WPI_SolenoidSet.vi"("Value"=WPI_SolenoidValue."On", "SolenoidDevRef"=w1500) -> ()  [unwired: 8 in, 2 out]
          n741 = call <vilib>:"WPI_CANTalonSRX_ChangeMode.vi"("Control Mode"=WPI_CANTalonSRX_APIControlMode."Percent VBus", "CAN Talon SRX Ref"=w1496) -> ("CAN Talon SRX Ref"=w1495:T14)  [unwired: 8 in, 1 out]
          n742 = call <vilib>:"WPI_MotorControlSetOutput.vi"("Output"=-0.4, "MotorControlDevRef"=w1495) -> ()  [unwired: 7 in, 3 out]
        }
        frame #6 {
          w1527 = -0.5 ("Left axis value")
          n743 = call <vilib>:"WPI_RobotDriveRefNum Registry Get.vi"("refnum name"="RobotDrive") -> ("error out"=w1528:errorcluster, "RobotDriveDevRef"=w1529:T13)  [unwired: 9 in]
          n744 = call <vilib>:"WPI_RobotDriveTankDrive.vi"("error in (no error)"=w1528, "Right axis value"=w1527, "Left axis value"=w1527, "RobotDriveDevRef"=w1529) -> ()  [unwired: 5 in, 3 out]
          n745 = call <vilib>:"WPI_MotorControlRefNum Registry Get.vi"("refnum name"="Shooter") -> ("MotorControlDevRef"=w1524:T14)  [unwired: 9 in, 1 out]
          n746 = call <vilib>:"WPI_CANTalonSRX_ChangeMode.vi"("Control Mode"=WPI_CANTalonSRX_APIControlMode."Percent VBus", "CAN Talon SRX Ref"=w1524) -> ("CAN Talon SRX Ref"=w1523:T14)  [unwired: 8 in, 1 out]
          n747 = Wait (ms)(milliseconds to wait=4000) -> ()  [unwired: 1 out]
          n748 = call <vilib>:"WPI_MotorControlSetOutput.vi"("Output"=-0.4, "MotorControlDevRef"=w1523) -> ()  [unwired: 7 in, 3 out]
        }
        frame #7 {
          n749 = call <vilib>:"WPI_RobotDriveRefNum Registry Get.vi"("refnum name"="RobotDrive") -> ("error out"=w1539:errorcluster, "RobotDriveDevRef"=w1540:T13)  [unwired: 9 in]
          n750 = call <vilib>:"WPI_MotorControlRefNum Registry Get.vi"("refnum name"="Shooter") -> ("MotorControlDevRef"=w1533:T14)  [unwired: 9 in, 1 out]
          n751 = call <vilib>:"WPI_RobotDriveTankDrive.vi"("error in (no error)"=w1539, "Right axis value"=0.5, "Left axis value"=0.0, "RobotDriveDevRef"=w1540) -> ()  [unwired: 5 in, 3 out]
          n752 = Wait (ms)(milliseconds to wait=1000) -> ()  [unwired: 1 out]
          n753 = call <vilib>:"WPI_CANTalonSRX_ChangeMode.vi"("Control Mode"=WPI_CANTalonSRX_APIControlMode."Percent VBus", "CAN Talon SRX Ref"=w1533) -> ("CAN Talon SRX Ref"=w1532:T14)  [unwired: 8 in, 1 out]
          n754 = call <vilib>:"WPI_MotorControlSetOutput.vi"("Output"=-0.4, "MotorControlDevRef"=w1532) -> ()  [unwired: 7 in, 3 out]
        }
        frame #8 {
          n755 = Wait (ms)(milliseconds to wait=4000) -> ()  [unwired: 1 out]
          n756 = call <vilib>:"WPI_MotorControlRefNum Registry Get.vi"("refnum name"="Shooter") -> ("MotorControlDevRef"=w1555:T14)  [unwired: 9 in, 1 out]
          n757 = Multiply(x=0.9, y=-1.0) -> (x*y=w1544:dbl)
          n758 = call <vilib>:"WPI_CANTalonSRX_ChangeMode.vi"("Control Mode"=WPI_CANTalonSRX_APIControlMode."Percent VBus", "CAN Talon SRX Ref"=w1555) -> ("CAN Talon SRX Ref"=w1554:T14)  [unwired: 8 in, 1 out]
          n759 = call <vilib>:"WPI_MotorControlSetOutput.vi"("Output"=-0.4, "MotorControlDevRef"=w1554) -> ()  [unwired: 7 in, 3 out]
          n760 = call <vilib>:"WPI_MotorControlRefNum Registry Get.vi"("refnum name"="Feeder") -> ("error out"=w1546:errorcluster, "MotorControlDevRef"=w1547:T14)  [unwired: 9 in]
          n761 = call <vilib>:"WPI_MotorControlRefNum Registry Get.vi"("refnum name"="Shuriken") -> ("error out"=w1548:errorcluster, "MotorControlDevRef"=w1549:T14)  [unwired: 9 in]
          n762 = call <vilib>:"WPI_RobotDriveRefNum Registry Get.vi"("refnum name"="RobotDrive") -> ("error out"=w1560:errorcluster, "RobotDriveDevRef"=w1561:T13)  [unwired: 9 in]
          n763 = call <vilib>:"WPI_MotorControlSetOutput.vi"("error in (no error)"=w1546, "Output"=w1544, "MotorControlDevRef"=w1547) -> ()  [unwired: 6 in, 3 out]
          n764 = call <vilib>:"WPI_MotorControlSetOutput.vi"("error in (no error)"=w1548, "Output"=0.4, "MotorControlDevRef"=w1549) -> ()  [unwired: 6 in, 3 out]
          n765 = call <vilib>:"WPI_RobotDriveTankDrive.vi"("error in (no error)"=w1560, "Right axis value"=0.0, "Left axis value"=0.0, "RobotDriveDevRef"=w1561) -> ()  [unwired: 5 in, 3 out]
        }
        frame #9 {
          n766 = call <vilib>:"WPI_MotorControlRefNum Registry Get.vi"("refnum name"="Shooter") -> ("MotorControlDevRef"=w1580:T14)  [unwired: 9 in, 1 out]
          n767 = call <vilib>:"WPI_RobotDriveRefNum Registry Get.vi"("refnum name"="RobotDrive") -> ("error out"=w1563:errorcluster, "RobotDriveDevRef"=w1562:T13)  [unwired: 9 in]
          n768 = Multiply(x=0.0, y=-1.0) -> (x*y=w1569:dbl)
          n769 = call <vilib>:"WPI_RobotDriveTankDrive.vi"("error in (no error)"=w1563, "Right axis value"=0.0, "Left axis value"=0.0, "RobotDriveDevRef"=w1562) -> ()  [unwired: 5 in, 3 out]
          n770 = call <vilib>:"WPI_CANTalonSRX_ChangeMode.vi"("Control Mode"=WPI_CANTalonSRX_APIControlMode."Percent VBus", "CAN Talon SRX Ref"=w1580) -> ("CAN Talon SRX Ref"=w1579:T14)  [unwired: 8 in, 1 out]
          n771 = call <vilib>:"WPI_MotorControlSetOutput.vi"("Output"=0.0, "MotorControlDevRef"=w1579) -> ()  [unwired: 7 in, 3 out]
          n772 = call <vilib>:"WPI_MotorControlRefNum Registry Get.vi"("refnum name"="Feeder") -> ("error out"=w1571:errorcluster, "MotorControlDevRef"=w1572:T14)  [unwired: 9 in]
          n773 = call <vilib>:"WPI_MotorControlRefNum Registry Get.vi"("refnum name"="Shuriken") -> ("error out"=w1573:errorcluster, "MotorControlDevRef"=w1574:T14)  [unwired: 9 in]
          n774 = call <vilib>:"WPI_MotorControlSetOutput.vi"("error in (no error)"=w1571, "Output"=w1569, "MotorControlDevRef"=w1572) -> ()  [unwired: 6 in, 3 out]
          n775 = call <vilib>:"WPI_MotorControlSetOutput.vi"("error in (no error)"=w1573, "Output"=0.0, "MotorControlDevRef"=w1574) -> ()  [unwired: 6 in, 3 out]
        }
      }
    }
    frame "RightPegPathBoiler" {
      n776 = flat-sequence {
        tunnel: [w1599] -> w1591
        tunnel: w1591 -> [w1624]
        tunnel: w1587 -> [w1623]
        tunnel: w1588 -> [w1622]
        tunnel: w1589 -> [w1621]
        tunnel: w1582 -> [w1620]
        tunnel: w1585 -> [w1692]
        tunnel: w1584 -> [w1691]
        tunnel: w1586 -> [w1690]
        tunnel: w1583 -> [w1789]
        tunnel: [w1789] -> w1590
        tunnel: w1590 -> [w1828]
        frame #0 {
          n777 = call <vilib>:"WPI_SolenoidRefNum Registry Get.vi"("refnum name"="Banana") -> ("SolenoidDevRef"=w1594:T5)  [unwired: 9 in, 1 out]
          n778 = call-poly <vilib>:"WPI_SolenoidSet.vi"("Value"=WPI_SolenoidValue."On", "SolenoidDevRef"=w1594) -> ()  [unwired: 8 in, 2 out]
          n779 = call "ReadFile.vi"("Name"="/home/lvuser/RightPegPathBoiler.txt") -> ("Array - Numeric"=w1599:dbl[][])
          n780 = global write "Robot Global Data.vi" "PathPlanningv1"(w1599) -> ()
          n781 = call <vilib>:"WPI_SolenoidRefNum Registry Get.vi"("refnum name"="GearGate") -> ("error out"=w1598:errorcluster, "SolenoidDevRef"=w1597:T5)  [unwired: 9 in]
          n782 = call-poly <vilib>:"WPI_SolenoidSet.vi"("error in (no error)"=w1598, "Value"=WPI_SolenoidValue."On", "SolenoidDevRef"=w1597) -> ()  [unwired: 7 in, 2 out]
        }
        frame #1 {
          # "Position PID or Velocity PID"
          n783 = call <vilib>:"WPI_SolenoidRefNum Registry Get.vi"("refnum name"="Banana") -> ("SolenoidDevRef"=w1619:T5)  [unwired: 9 in, 1 out]
          n784 = call-poly <vilib>:"WPI_SolenoidSet.vi"("Value"=WPI_SolenoidValue."On", "SolenoidDevRef"=w1619) -> ()  [unwired: 8 in, 2 out]
          n785 = call <vilib>:"WPI_EncoderRefNum Registry Get.vi"("refnum name"="Encoder 0") -> ("error out"=w1613:errorcluster, "EncoderDevRef"=w1612:T7)  [unwired: 9 in]
          n786 = call <vilib>:"WPI_EncoderRefNum Registry Get.vi"("refnum name"="Encoder 1") -> ("error out"=w1615:errorcluster, "EncoderDevRef"=w1614:T7)  [unwired: 9 in]
          n787 = call "Z900_navX_RefNum_Get.vi"("refnum name"="navX") -> ("error out"=w1604:errorcluster, "navX Device"=w1605:T11)  [unwired: 9 in]
          n788 = call "Z900_navX_Set_ZeroYaw.vi"("error in (no error)"=w1604, "navX Device"=w1605) -> ("error out"=w1602:errorcluster, "navX Device"=w1603:T11)  [unwired: 8 in]
          n789 = call <vilib>:"WPI_EncoderReset.vi"("error in (no error)"=w1613, "EncoderDevRef"=w1612) -> ("error out"=w1609:errorcluster, "EncoderDevRef"=w1610:T7)  [unwired: 8 in]
          n790 = call <vilib>:"WPI_EncoderReset.vi"("error in (no error)"=w1615, "EncoderDevRef"=w1614) -> ("error out"=w1608:errorcluster, "EncoderDevRef"=w1611:T7)  [unwired: 8 in]
          n791 = Array Size(array=w1624) -> (size(s)=w1628:i32[])
          n792 = call <vilib>:"WPI_RobotDriveRefNum Registry Get.vi"("refnum name"="RobotDrive") -> ("RobotDriveDevRef"=w1625:T13)  [unwired: 9 in, 1 out]
          n793 = Index Array(array=w1628, index=0) -> (element=w1616:i32)
          n794 = for {
            N: w1616 -> [_]
            tunnel: w1624 -> [w1647]
            tunnel: w1620 -> [w1644]
            tunnel: w1622 -> [w1643]
            tunnel: w1623 -> [w1642]
            tunnel: w1625 -> [w1641]
            tunnel: w1621 -> [w1640]
            tunnel: w1611 -> [w1639]
            tunnel: w1610 -> [w1638]
            tunnel: w1609 -> [w1637]
            tunnel: w1608 -> [w1636]
            tunnel: w1603 -> [w1633]
            tunnel: w1602 -> [w1632]
            i -> [w1646]
            n795 = Index Array(array=w1647, index (row)=w1646) -> (element=w1631:dbl[])  [unwired: 1 in]
            n796 = Index Array(array=w1631, index=0) -> (element=w1634:dbl)
            n797 = Index Array(array=w1631, index=1) -> (element=w1635:dbl)
            n798 = Index Array(array=w1631, index=2) -> (element=w1629:dbl)
            n799 = for {
              N: 10 -> [_]
              tunnel: w1644 -> [w1671]
              tunnel: w1643 -> [w1685]
              tunnel: w1642 -> [w1656]
              tunnel: w1641 -> [w1686]
              tunnel: w1640 -> [w1672]
              tunnel: w1639 -> [w1666]
              tunnel: w1638 -> [w1665]
              tunnel: w1637 -> [w1662]
              tunnel: w1636 -> [w1661]
              tunnel: w1634 -> [w1660]
              tunnel: w1635 -> [w1659]
              tunnel: w1633 -> [w1655]
              tunnel: w1632 -> [w1654]
              tunnel: w1629 -> [w1650]
              w1667 = 0.0011393 ("x")
              n800 = call <vilib>:"WPI_EncoderGet.vi"("error in (no error)"=w1661, "EncoderDevRef"=w1666) -> ("Distance"=w1663:dbl)  [unwired: 4 in, 5 out]
              n801 = call <vilib>:"WPI_EncoderGet.vi"("error in (no error)"=w1662, "EncoderDevRef"=w1665) -> ("Distance"=w1664:dbl)  [unwired: 4 in, 5 out]
              n802 = Multiply(x=w1667, y=w1664) -> (x*y=w1668:dbl)
              n803 = Divide(x=w1668, y=w1672) -> (x/y=w1670:dbl)
              n804 = Multiply(x=w1667, y=w1663) -> (x*y=w1669:dbl)
              n805 = Divide(x=w1669, y=w1672) -> (x/y=w1682:dbl)
              n806 = call-poly <vilib>:"PID.vi"("output range"=w1656, "PID gains"=w1685, "process variable"=w1682, "setpoint"=w1660) -> ("output"=w1657:dbl)  [unwired: 6 in, 1 out]
              n807 = call-poly <vilib>:"PID.vi"("output range"=w1656, "PID gains"=w1671, "process variable"=w1670, "setpoint"=w1659) -> ("output"=w1658:dbl)  [unwired: 6 in, 1 out]
              n808 = call "Z900_navX_Get_YPRHfH.vi"("error in (no error)"=w1654, "navX Device"=w1655) -> ("YRPHfH"=w1653:T18)  [unwired: 6 in, 3 out]
              n809 = Bundle("output"=w1658, w1670, "Numeric"=w1659) -> (→"Left V 4":cluster{"output":dbl, dbl, "Numeric":dbl})  [unwired: 1 in]
              n810 = Unbundle By Name(w1653) -> ("Yaw"=w1651:dbl)
              n811 = call <vilib>:"WPI_SolenoidRefNum Registry Get.vi"("refnum name"="GearGate") -> ("error out"=w1681:errorcluster, "SolenoidDevRef"=w1680:T5)  [unwired: 9 in]
              n812 = call <vilib>:"WPI_RobotDriveTankDrive.vi"("Right axis value"=w1658, "Left axis value"=w1657, "RobotDriveDevRef"=w1686) -> ()  [unwired: 6 in, 3 out]
              n813 = call-poly <vilib>:"WPI_SolenoidSet.vi"("error in (no error)"=w1681, "Value"=WPI_SolenoidValue."On", "SolenoidDevRef"=w1680) -> ()  [unwired: 7 in, 2 out]
              n814 = Divide(x=10, y=w1672) -> (x/y=w1673:dbl)
              n815 = call <vilib>:"WPI_SolenoidRefNum Registry Get.vi"("refnum name"="Banana") -> ("SolenoidDevRef"=w1677:T5)  [unwired: 9 in, 1 out]
              n816 = Bundle("Numeric"=w1650, "Yaw"=w1651) -> (→"Yaw 4":cluster{"Numeric":dbl, "Yaw":dbl})  [unwired: 1 in]
              n817 = Bundle("output"=w1657, w1682, "Numeric"=w1660) -> (→"Right V 4":cluster{"output":dbl, dbl, "Numeric":dbl})  [unwired: 1 in]
              n818 = Wait (ms)(milliseconds to wait=w1673) -> ()  [unwired: 1 out]
              n819 = call-poly <vilib>:"WPI_SolenoidSet.vi"("Value"=WPI_SolenoidValue."On", "SolenoidDevRef"=w1677) -> ()  [unwired: 8 in, 2 out]
            }
          }
        }
        frame #2 {
          w1688 = 0.0 ("Right axis value")
          n820 = call <vilib>:"WPI_RobotDriveRefNum Registry Get.vi"("refnum name"="RobotDrive") -> ("RobotDriveDevRef"=w1689:T13)  [unwired: 9 in, 1 out]
          n821 = call <vilib>:"WPI_RobotDriveTankDrive.vi"("Right axis value"=w1688, "Left axis value"=w1688, "RobotDriveDevRef"=w1689) -> ()  [unwired: 6 in, 3 out]
        }
        frame #3 {
          n822 = for {
            N: 10 -> [_]
            tunnel: w1692 -> [w1696]
            tunnel: w1691 -> [w1695]
            tunnel: w1690 -> [w1694]
            n823 = global read "Robot Global Data.vi" "TargetsFound"() -> (w1699:bool)
            n824 = case shown="False" w1699 {
              tunnel: [w1707 w1715] -> w1698
              tunnel: [w1707 w1714] -> w1697
              tunnel: w1696 -> [_ w1710]
              tunnel: w1695 -> [_ w1709]
              tunnel: w1694 -> [_ w1708]
              frame False {
                w1707 = 0.0
              }
              frame True {
                n825 = global read "Robot Global Data.vi" "Mid"() -> (w1718:dbl)
                n826 = Subtract(x=w1718, y=w1709) -> (x-y=w1712:dbl)
                n827 = Absolute Value(x=w1712) -> (abs(x)=w1717:dbl)
                n828 = Less?(x=w1717, y=w1708) -> (x < y?=w1716:bool)
                n829 = Greater?(x=w1712, y=0.0) -> (0:w1713:bool)
                n830 = case shown="True" w1713 {
                  tunnel: w1716 -> [w1721 w1734]
                  tunnel: [w1719 w1732] -> w1715
                  tunnel: [w1720 w1733] -> w1714
                  tunnel: w1710 -> [w1722 w1731]
                  frame False {
                    n831 = case shown="True" w1721 {
                      tunnel: [w1727 w1730] -> w1720
                      tunnel: [w1725 w1730] -> w1719
                      tunnel: w1722 -> [w1723 w1728]
                      frame False {
                        n832 = Multiply(x=w1723, y=-1.0) -> (x*y=w1727:dbl)
                        n833 = Multiply(x=w1723, y=1.2) -> (x*y=w1725:dbl)
                      }
                      frame True {
                        n834 = Multiply(x=w1728, y=1.2) -> (x*y=w1730:dbl)
                      }
                    }
                  }
                  frame True {
                    n835 = case shown="False" w1734 {
                      tunnel: [w1739 w1742] -> w1733
                      tunnel: [w1737 w1742] -> w1732
                      tunnel: w1731 -> [w1735 w1740]
                      frame False {
                        n836 = Multiply(x=w1735, y=-1.0) -> (x*y=w1737:dbl)
                        n837 = Multiply(x=w1735, y=1.0) -> (x*y=w1739:dbl)
                      }
                      frame True {
                        n838 = Multiply(x=w1740, y=1.0) -> (x*y=w1742:dbl)
                      }
                    }
                  }
                }
              }
            }
            n839 = call <vilib>:"WPI_SolenoidRefNum Registry Get.vi"("refnum name"="Banana") -> ("SolenoidDevRef"=w1702:T5)  [unwired: 9 in, 1 out]
            n840 = call-poly <vilib>:"WPI_SolenoidSet.vi"("Value"=WPI_SolenoidValue."On", "SolenoidDevRef"=w1702) -> ()  [unwired: 8 in, 2 out]
            n841 = call <vilib>:"WPI_RobotDriveRefNum Registry Get.vi"("refnum name"="RobotDrive") -> ("error out"=w1705:errorcluster, "RobotDriveDevRef"=w1706:T13)  [unwired: 9 in]
            n842 = Wait (ms)(milliseconds to wait=100) -> ()  [unwired: 1 out]
            n843 = call <vilib>:"WPI_RobotDriveTankDrive.vi"("error in (no error)"=w1705, "Right axis value"=w1698, "Left axis value"=w1697, "RobotDriveDevRef"=w1706) -> ()  [unwired: 5 in, 3 out]
          }
        }
        frame #4 {
          w1751 = 0.0 ("Left axis value")
          n844 = call <vilib>:"WPI_SolenoidRefNum Registry Get.vi"("refnum name"="Banana") -> ("SolenoidDevRef"=w1745:T5)  [unwired: 9 in, 1 out]
          n845 = call <vilib>:"WPI_RobotDriveRefNum Registry Get.vi"("refnum name"="RobotDrive") -> ("error out"=w1752:errorcluster, "RobotDriveDevRef"=w1753:T13)  [unwired: 9 in]
          n846 = call <vilib>:"WPI_SolenoidRefNum Registry Get.vi"("refnum name"="GearGate") -> ("error out"=w1749:errorcluster, "SolenoidDevRef"=w1748:T5)  [unwired: 9 in]
          n847 = call-poly <vilib>:"WPI_SolenoidSet.vi"("Value"=WPI_SolenoidValue."On", "SolenoidDevRef"=w1745) -> ()  [unwired: 8 in, 2 out]
          n848 = call <vilib>:"WPI_RobotDriveTankDrive.vi"("error in (no error)"=w1752, "Right axis value"=w1751, "Left axis value"=w1751, "RobotDriveDevRef"=w1753) -> ()  [unwired: 5 in, 3 out]
          n849 = call-poly <vilib>:"WPI_SolenoidSet.vi"("error in (no error)"=w1749, "Value"=WPI_SolenoidValue."On", "SolenoidDevRef"=w1748) -> ()  [unwired: 7 in, 2 out]
        }
        frame #5 {
          n850 = for {
            N: 3 -> [_]
            n851 = flat-sequence {
              frame #0 {
                n852 = call <vilib>:"WPI_SolenoidRefNum Registry Get.vi"("refnum name"="Gears") -> ("error out"=w1766:errorcluster, "SolenoidDevRef"=w1765:T5)  [unwired: 9 in]
                n853 = call <vilib>:"WPI_SolenoidRefNum Registry Get.vi"("refnum name"="GearGate") -> ("error out"=w1761:errorcluster, "SolenoidDevRef"=w1760:T5)  [unwired: 9 in]
                n854 = call-poly <vilib>:"WPI_SolenoidSet.vi"("error in (no error)"=w1766, "Value"=WPI_SolenoidValue."On", "SolenoidDevRef"=w1765) -> ()  [unwired: 7 in, 2 out]
                n855 = Wait (ms)(milliseconds to wait=166) -> ()  [unwired: 1 out]
                n856 = call-poly <vilib>:"WPI_SolenoidSet.vi"("error in (no error)"=w1761, "Value"=WPI_SolenoidValue."On", "SolenoidDevRef"=w1760) -> ()  [unwired: 7 in, 2 out]
              }
              frame #1 {
                n857 = call <vilib>:"WPI_SolenoidRefNum Registry Get.vi"("refnum name"="Gears") -> ("error out"=w1775:errorcluster, "SolenoidDevRef"=w1774:T5)  [unwired: 9 in]
                n858 = call <vilib>:"WPI_SolenoidRefNum Registry Get.vi"("refnum name"="GearGate") -> ("error out"=w1770:errorcluster, "SolenoidDevRef"=w1769:T5)  [unwired: 9 in]
                n859 = Wait (ms)(milliseconds to wait=166) -> ()  [unwired: 1 out]
                n860 = call-poly <vilib>:"WPI_SolenoidSet.vi"("error in (no error)"=w1775, "Value"=WPI_SolenoidValue."Off", "SolenoidDevRef"=w1774) -> ()  [unwired: 7 in, 2 out]
                n861 = call-poly <vilib>:"WPI_SolenoidSet.vi"("error in (no error)"=w1770, "Value"=WPI_SolenoidValue."On", "SolenoidDevRef"=w1769) -> ()  [unwired: 7 in, 2 out]
              }
            }
          }
          n862 = call <vilib>:"WPI_SolenoidRefNum Registry Get.vi"("refnum name"="Banana") -> ("SolenoidDevRef"=w1756:T5)  [unwired: 9 in, 1 out]
          n863 = call-poly <vilib>:"WPI_SolenoidSet.vi"("Value"=WPI_SolenoidValue."On", "SolenoidDevRef"=w1756) -> ()  [unwired: 8 in, 2 out]
        }
        frame #6 {
          w1778 = -0.7 ("Left axis value")
          n864 = call <vilib>:"WPI_RobotDriveRefNum Registry Get.vi"("refnum name"="RobotDrive") -> ("error out"=w1779:errorcluster, "RobotDriveDevRef"=w1780:T13)  [unwired: 9 in]
          n865 = call <vilib>:"WPI_RobotDriveTankDrive.vi"("error in (no error)"=w1779, "Right axis value"=w1778, "Left axis value"=w1778, "RobotDriveDevRef"=w1780) -> ()  [unwired: 5 in, 3 out]
          n866 = Wait (ms)(milliseconds to wait=1000) -> ()  [unwired: 1 out]
        }
        frame #7 {
          w1786 = 0.0 ("Left axis value")
          n867 = call <vilib>:"WPI_RobotDriveRefNum Registry Get.vi"("refnum name"="RobotDrive") -> ("error out"=w1787:errorcluster, "RobotDriveDevRef"=w1788:T13)  [unwired: 9 in]
          n868 = call <vilib>:"WPI_SolenoidRefNum Registry Get.vi"("refnum name"="GearGate") -> ("error out"=w1784:errorcluster, "SolenoidDevRef"=w1783:T5)  [unwired: 9 in]
          n869 = call <vilib>:"WPI_RobotDriveTankDrive.vi"("error in (no error)"=w1787, "Right axis value"=w1786, "Left axis value"=w1786, "RobotDriveDevRef"=w1788) -> ()  [unwired: 5 in, 3 out]
          n870 = call-poly <vilib>:"WPI_SolenoidSet.vi"("error in (no error)"=w1784, "Value"=WPI_SolenoidValue."Off", "SolenoidDevRef"=w1783) -> ()  [unwired: 7 in, 2 out]
        }
        frame #8 {
          n871 = call "Z900_navX_RefNum_Get.vi"("refnum name"="navX") -> ("error out"=w1793:errorcluster, "navX Device"=w1794:T11)  [unwired: 9 in]
          n872 = call "Z900_navX_Set_ZeroYaw.vi"("error in (no error)"=w1793, "navX Device"=w1794) -> ("error out"=w1790:errorcluster, "navX Device"=w1791:T11)  [unwired: 8 in]
          n873 = call <vilib>:"WPI_SolenoidRefNum Registry Get.vi"("refnum name"="GearGate") -> ("error out"=w1798:errorcluster, "SolenoidDevRef"=w1797:T5)  [unwired: 9 in]
          n874 = call-poly <vilib>:"WPI_SolenoidSet.vi"("error in (no error)"=w1798, "Value"=WPI_SolenoidValue."On", "SolenoidDevRef"=w1797) -> ()  [unwired: 7 in, 2 out]
          n875 = while {
            tunnel: w1791 -> [w1808]
            tunnel: w1790 -> [w1807]
            tunnel: w1789 -> [_]
            i -> [w1812]
            stop <- w1809 stop-if-true
            w1799 = 0.5
            w1825 = 0.0
            n876 = call "Z900_navX_Get_YPRHfH.vi"("error in (no error)"=w1807, "navX Device"=w1808) -> ("YRPHfH"=w1806:T18)  [unwired: 6 in, 3 out]
            n877 = Unbundle By Name(w1806) -> ("Yaw"=w1805:dbl)
            n878 = Subtract(x=w1805, y=-60.0) -> (x-y=w1803:dbl)
            n879 = Absolute Value(x=w1803) -> (abs(x)=w1802:dbl)
            n880 = Subtract(x=w1825, y=w1799) -> (x-y=w1823:dbl)
            n881 = Add(x=w1825, y=w1799) -> (x+y=w1822:dbl)
            n882 = call <vilib>:"WPI_RobotDriveRefNum Registry Get.vi"("refnum name"="RobotDrive") -> ("RobotDriveDevRef"=w1827:T13)  [unwired: 9 in, 1 out]
            n883 = Less?(x=w1802, y=0.5) -> (x < y?=w1800:bool)
            n884 = Greater?(x=w1812, y=200) -> (0:w1810:bool)
            n885 = call <vilib>:"WPI_SolenoidRefNum Registry Get.vi"("refnum name"="GearGate") -> ("error out"=w1819:errorcluster, "SolenoidDevRef"=w1818:T5)  [unwired: 9 in]
            n886 = call <vilib>:"WPI_RobotDriveTankDrive.vi"("Right axis value"=w1822, "Left axis value"=w1823, "RobotDriveDevRef"=w1827) -> ()  [unwired: 6 in, 3 out]
            n887 = call-poly <vilib>:"WPI_SolenoidSet.vi"("error in (no error)"=w1819, "Value"=WPI_SolenoidValue."On", "SolenoidDevRef"=w1818) -> ()  [unwired: 7 in, 2 out]
            n888 = Or(x=w1800, y=w1810) -> (x .or. y?=w1809:bool)
            n889 = Build Array(w1823, w1822, w1805) -> (w1820:dbl[])
            n890 = Array To Cluster(array=w1820) -> (cluster=→"DriveStraight 7":T1)
            n891 = call <vilib>:"WPI_SolenoidRefNum Registry Get.vi"("refnum name"="Banana") -> ("SolenoidDevRef"=w1815:T5)  [unwired: 9 in, 1 out]
            n892 = call-poly <vilib>:"WPI_SolenoidSet.vi"("Value"=WPI_SolenoidValue."On", "SolenoidDevRef"=w1815) -> ()  [unwired: 8 in, 2 out]
            n893 = Wait (ms)(milliseconds to wait=10) -> ()  [unwired: 1 out]
          }
        }
        frame #9 {
          n894 = call <vilib>:"WPI_EncoderRefNum Registry Get.vi"("refnum name"="Encoder 1") -> ("error out"=w1840:errorcluster, "EncoderDevRef"=w1842:T7)  [unwired: 9 in]
          n895 = call <vilib>:"WPI_EncoderRefNum Registry Get.vi"("refnum name"="Encoder 0") -> ("error out"=w1841:errorcluster, "EncoderDevRef"=w1843:T7)  [unwired: 9 in]
          n896 = call <vilib>:"WPI_SolenoidRefNum Registry Get.vi"("refnum name"="GearGate") -> ("error out"=w1839:errorcluster, "SolenoidDevRef"=w1838:T5)  [unwired: 9 in]
          n897 = call-poly <vilib>:"NT Read Value.vi"("Default Value"=14.0, "Name"="Circumference") -> ("Numeric"=w1829:dbl)  [unwired: 8 in, 1 out]
          n898 = call-poly <vilib>:"WPI_SolenoidSet.vi"("error in (no error)"=w1839, "Value"=WPI_SolenoidValue."On", "SolenoidDevRef"=w1838) -> ()  [unwired: 7 in, 2 out]
          n899 = call <vilib>:"WPI_EncoderReset.vi"("error in (no error)"=w1841, "EncoderDevRef"=w1843) -> ("error out"=w1834:errorcluster, "EncoderDevRef"=w1835:T7)  [unwired: 8 in]
          n900 = call <vilib>:"WPI_EncoderReset.vi"("error in (no error)"=w1840, "EncoderDevRef"=w1842) -> ("error out"=w1832:errorcluster, "EncoderDevRef"=w1833:T7)  [unwired: 8 in]
          n901 = while {
            tunnel: w1835 -> [w1865]
            tunnel: w1834 -> [w1864]
            tunnel: w1833 -> [w1863]
            tunnel: w1832 -> [w1862]
            tunnel: w1829 -> [w1847]
            tunnel: w1828 -> [w1846]
            i -> [w1852]
            stop <- w1848 stop-if-true
            w1880 = 0.7
            n902 = call <vilib>:"WPI_EncoderGet.vi"("error in (no error)"=w1864, "EncoderDevRef"=w1865) -> ("Distance"=w1861:dbl)  [unwired: 4 in, 5 out]
            n903 = call <vilib>:"WPI_EncoderGet.vi"("error in (no error)"=w1862, "EncoderDevRef"=w1863) -> ("Distance"=w1860:dbl)  [unwired: 4 in, 5 out]
            n904 = Subtract(x=w1861, y=w1860) -> (x-y=w1874:dbl)
            n905 = Add(x=w1861, y=w1860) -> (x+y=w1859:dbl)
            n906 = call-poly <vilib>:"PID.vi"("output range"=cluster{"output high":dbl, "output low":dbl} {"output high"=0.5, "output low"=-0.5}, "PID gains"=w1846, "process variable"=w1874, "setpoint"=0.0) -> ("output"=w1881:dbl)  [unwired: 6 in, 1 out]
            n907 = Divide(x=w1859, y=2.0) -> (x/y=w1854:dbl)
            n908 = Subtract(x=w1880, y=w1881) -> (x-y=w1876:dbl)
            n909 = Add(x=w1880, y=w1881) -> (x+y=w1875:dbl)
            n910 = call <vilib>:"WPI_RobotDriveRefNum Registry Get.vi"("refnum name"="RobotDrive") -> ("RobotDriveDevRef"=w1883:T13)  [unwired: 9 in, 1 out]
            n911 = Greater?(x=w1852, y=400) -> (0:w1849:bool)
            n912 = Divide(x=48.0, y=w1847) -> (x/y=w1856:dbl)
            n913 = call <vilib>:"WPI_SolenoidRefNum Registry Get.vi"("refnum name"="GearGate") -> ("error out"=w1872:errorcluster, "SolenoidDevRef"=w1871:T5)  [unwired: 9 in]
            n914 = call <vilib>:"WPI_RobotDriveTankDrive.vi"("Right axis value"=w1875, "Left axis value"=w1876, "RobotDriveDevRef"=w1883) -> ()  [unwired: 6 in, 3 out]
            n915 = Multiply(x=w1856, y=1024.0) -> (x*y=w1853:dbl)
            n916 = Greater Or Equal?(x=w1854, y=w1853) -> (x >= y?=w1850:bool)
            n917 = call-poly <vilib>:"WPI_SolenoidSet.vi"("error in (no error)"=w1872, "Value"=WPI_SolenoidValue."On", "SolenoidDevRef"=w1871) -> ()  [unwired: 7 in, 2 out]
            n918 = Or(x=w1850, y=w1849) -> (x .or. y?=w1848:bool)
            n919 = Build Array(w1876, w1875, w1874) -> (w1873:dbl[])
            n920 = Array To Cluster(array=w1873) -> ()  [unwired: 1 out]
            n921 = call <vilib>:"WPI_SolenoidRefNum Registry Get.vi"("refnum name"="Banana") -> ("SolenoidDevRef"=w1868:T5)  [unwired: 9 in, 1 out]
            n922 = call-poly <vilib>:"WPI_SolenoidSet.vi"("Value"=WPI_SolenoidValue."On", "SolenoidDevRef"=w1868) -> ()  [unwired: 8 in, 2 out]
            n923 = Wait (ms)(milliseconds to wait=10) -> ()  [unwired: 1 out]
          }
        }
      }
    }
    frame "Nothing" {
    }
  }
  n924 = disable-structure shown="Disabled" {
    frame Disabled {
      n925 = call <vilib>:"WPI_SolenoidRefNum Registry Get.vi"("refnum name"="Banana") -> ("SolenoidDevRef"=w1885:T5)  [unwired: 9 in, 1 out]
      n926 = call-poly <vilib>:"WPI_SolenoidSet.vi"("Value"=WPI_SolenoidValue."On", "SolenoidDevRef"=w1885) -> ()  [unwired: 8 in, 2 out]
    }
    frame Enabled {
    }
  }
